vi "MultiOpto_1.4_Host.vi"() -> ()   [LabVIEW 2018]
uses:
  D:/NI LabVIEW/MultiOpto/MultiOpto_1.4/AT lib/Spels.AutomationTools.Utility.Wcf.dll
  AT lib/Spels.AutomationTools.Utility.Wcf.dll
  D:/NI LabVIEW/MultiOpto/MultiOpto_1.4/AT lib/AmateurStepperMotor.dll
  AT lib/AmateurStepperMotor.dll
  <instrlib>/niDCPower/nidcpower.llb/niDCPower Measurement Type.ctl
  <instrlib>/niDMM/nidmm.llb/niDMM Resolution in Digits.ctl
  <instrlib>/niDMM/nidmm.llb/niDMM Function.ctl
  <instrlib>/niDMM/nidmm.llb/niDMM Configure Measurement Digits.vi
  <instrlib>/niScope/Configure/Trigger/niScope Configure Trigger Window.vi
  <instrlib>/niScope/Acquire/Fetch/niScope Multi Fetch Cluster.vi
  <instrlib>/niScope/Acquire/Fetch/niScope Fetch.vi
panel:
  in  "POWER":bool
  in  "DC POWER 2":refnum<k15>="PXI1Slot3_3" caption="PRBS"
  in  "DC POWER 1":refnum<k15>="PXI1Slot2_2" caption="VСС_+5"
  in  "Tab DC Power 4":enum32{"DC Power 4", "System Panel"}(tab)
  in  "P4 CH2":bool
  out "P4 CH2_char":dbl(graph)=-2.6497095286784e-07
  in  "P4 CH2, V":dbl caption="voltage level" min=-20.0 max=0.0 format="%_6p"
  out "P4 CH2_cur, A":dbl=-2.6497095286784e-07 caption="measurement" format="%_6g"
  in  "P4 CH2_curlim, A":dbl=0.015 caption="current limit" min=0.01 max=1.0 format="%_6p"
  in  "P4 CH1":bool
  out "P4 CH1_char":dbl(graph)=-6.586231837824974e-06
  in  "P4 CH1, V":dbl=20.0 caption="voltage level" min=0.0 max=20.0 format="%_6p"
  out "P4 CH1_cur, A":dbl=-6.586231837824974e-06 caption="measurement" format="%_6g"
  in  "P4 CH1_curlim, A":dbl=0.1 caption="current limit" min=0.01 max=1.0 format="%_6p"
  in  "P4 CH0":bool
  out "P4 CH0_char":dbl(graph)=0.00011627237241327378
  in  "P4 CH0, V":dbl=1.2000000000000002 caption="voltage level" min=0.0 max=6.0 format="%_6p"
  out "P4 CH0_cur, A":dbl=0.00011627237241327378 caption="measurement" format="%_6g"
  in  "P4 CH0_curlim, A":dbl=0.04 caption="current limit" min=0.01 max=1.0 format="%_6p"
  in  "P4 CH0_selcur, A":dbl=0.2 caption="current limit" format="%_6p"
  out "P4 CH0_warning":bool caption="VCC_warning"
  out "P4 CH0_counter":u32 caption="VCC_counter"
  in  "P4 CH1_selcur, A":dbl=0.2 caption="current limit" format="%_6p"
  out "P4 CH1_warning":bool caption="VCC_warning"
  out "P4 CH1_counter":u32 caption="VCC_counter"
  in  "P4 CH2_selcur, A":dbl=0.2 caption="current limit" format="%_6p"
  out "P4 CH2_warning":bool caption="VCC_warning"
  out "P4 CH2_counter":u32 caption="VCC_counter"
  in  "P4 CH2 Used":bool caption="CH2"
  in  "P4 CH0 Used":bool caption="CH0"
  in  "P4 CH1 Used":bool caption="CH1"
  out "DC Power 4 error out":errorcluster
  in  "Tab DC Power 3":enum32{"DC Power 3", "System Panel"}(tab)
  in  "P3 CH2":bool
  out "P3 CH2_char":dbl(graph)=-2.6497095286784e-07
  in  "P3 CH2, V":dbl caption="voltage level" min=-20.0 max=0.0 format="%_6p"
  out "P3 CH2_cur, A":dbl=-2.6497095286784e-07 caption="measurement" format="%_6g"
  in  "P3 CH2_curlim, A":dbl=0.015 caption="current limit" min=0.01 max=1.0 format="%_6p"
  in  "P3 CH1":bool
  out "P3 CH1_char":dbl(graph)=-6.586231837824974e-06
  in  "P3 CH1, V":dbl=20.0 caption="voltage level" min=0.0 max=20.0 format="%_6p"
  out "P3 CH1_cur, A":dbl=-6.586231837824974e-06 caption="measurement" format="%_6g"
  in  "P3 CH1_curlim, A":dbl=0.1 caption="current limit" min=0.01 max=1.0 format="%_6p"
  in  "P3 CH0":bool
  out "P3 CH0_char":dbl(graph)=0.00011627237241327378
  in  "P3 CH0, V":dbl=1.2000000000000002 caption="voltage level" min=0.0 max=6.0 format="%_6p"
  out "P3 CH0_cur, A":dbl=0.00011627237241327378 caption="measurement" format="%_6g"
  in  "P3 CH0_curlim, A":dbl=0.04 caption="current limit" min=0.01 max=1.0 format="%_6p"
  in  "P3 CH2_selcur, A":dbl=0.2 caption="current limit" format="%_6p"
  out "P3 CH2_warning":bool caption="VCC_warning"
  out "P3 CH2_counter":u32 caption="VCC_counter"
  in  "P3 CH1_selcur, A":dbl=0.2 caption="current limit" format="%_6p"
  out "P3 CH1_warning":bool caption="VCC_warning"
  out "P3 CH1_counter":u32 caption="VCC_counter"
  in  "P3 CH0_selcur, A":dbl=0.2 caption="current limit" format="%_6p"
  out "P3 CH0_warning":bool caption="VCC_warning"
  out "P3 CH0_counter":u32 caption="VCC_counter"
  in  "P3 CH2 Used":bool caption="CH2"
  in  "P3 CH1 Used":bool caption="CH1"
  in  "P3 CH0 Used":bool caption="CH0"
  out "DC Power 3 error out":errorcluster
  in  "DC POWER 4":refnum<k15>="PXI1Slot5_3" caption="PRBS"
  in  "DC POWER 3":refnum<k15>="PXI1Slot4_3" caption="PRBS"
  in  "Desicion Panel":enum32{"Decision Panel", "System Panel"}(tab)
  in  "HMI Stop":bool
  out "SEU":bool caption="SEL"
  out "SEL":bool
  out "DC Power 4 Status":bool caption="DC Power 4"
  out "DC Power 3 Status":bool caption="DC Power 3"
  out "DC Power 1 Status":bool caption="DC Power 1"
  out "DC Power 2 Status":bool caption="DC Power 2"
  out "NI DMM 1 Status":bool caption="NI DMM 1"
  out "NI DMM 2 Status":bool caption="NI DMM 2"
  out "NI DMM 3 Status":bool caption="NI DMM 3"
  out "NI Scope Status":bool caption="NI Scope"
  out "Stepper Motor Status":bool caption="Stepper Motor"
  out "Ophir 2 Status":bool caption="Ophir 2"
  out "Ophir 1 Status":bool caption="Ophir 1"
  in  "SEL Time Cycle":u32=100
  in  "SEL path":path=path "D:/NI LabVIEW/MultiOpto/MultiOpto_1.2/Logs/SEL" caption="SEL Path"
  in  "SIM_SEL":bool
  in  "Считать SIM_SEL":bool
  in  "System Stop":bool
  out "Ready Status":bool
  out "Power OFF":bool
  in  "Tab DC Power 2":enum32{"DC Power 2", "System Panel"}(tab)
  in  "P2 CH2_selcur, A":dbl=0.2 caption="current limit" format="%_6p"
  out "P2 CH2_warning":bool caption="VCC_warning"
  out "P2 CH2_counter":u32 caption="VCC_counter"
  in  "P2 CH2 Used":bool caption="CH2"
  in  "P2 CH2_curlim, A":dbl=0.015 caption="current limit" min=0.01 max=1.0 format="%_6p"
  out "P2 CH2_cur, A":dbl=-2.6497095286784e-07 caption="measurement" format="%_6g"
  in  "P2 CH2, V":dbl caption="voltage level" min=-20.0 max=0.0 format="%_6p"
  out "P2 CH2_char":dbl(graph)=-2.6497095286784e-07
  in  "P2 CH2":bool
  in  "P2 CH0 Used":bool caption="CH0"
  out "P2 CH0_char":dbl(graph)=0.00011627237241327378
  in  "P2 CH0, V":dbl=1.2000000000000002 caption="voltage level" min=0.0 max=6.0 format="%_6p"
  out "P2 CH0_cur, A":dbl=0.00011627237241327378 caption="measurement" format="%_6g"
  in  "P2 CH0_curlim, A":dbl=0.04 caption="current limit" min=0.01 max=1.0 format="%_6p"
  in  "P2 CH0":bool
  out "P2 CH0_warning":bool caption="VCC_warning"
  out "P2 CH0_counter":u32 caption="VCC_counter"
  in  "P2 CH0_selcur, A":dbl=0.2 caption="current limit" format="%_6p"
  in  "P2 CH1_curlim, A":dbl=0.1 caption="current limit" min=0.01 max=1.0 format="%_6p"
  out "P2 CH1_cur, A":dbl=-6.586231837824974e-06 caption="measurement" format="%_6g"
  in  "P2 CH1, V":dbl=20.0 caption="voltage level" min=0.0 max=20.0 format="%_6p"
  out "P2 CH1_char":dbl(graph)=-6.586231837824974e-06
  in  "P2 CH1":bool
  in  "P2 CH1 Used":bool caption="CH1"
  in  "P2 CH1_selcur, A":dbl=0.2 caption="current limit" format="%_6p"
  out "P2 CH1_counter":u32 caption="VCC_counter"
  out "P2 CH1_warning":bool caption="VCC_warning"
  out "DC Power 2 error out":errorcluster
  in  "Tab DC Power 1":enum32{"DC Power 1", "System Panel"}(tab)
  out "P1 CH2_counter":u32 caption="VCC_counter"
  out "P1 CH2_warning":bool caption="VCC_warning"
  in  "P1 CH2_selcur, A":dbl=0.2 caption="current limit" format="%_6p"
  in  "P1 CH2 Used":bool caption="CH2"
  in  "P1 CH2_curlim, A":dbl=0.01 caption="current limit" min=0.01 max=1.0 format="%_6p"
  out "P1 CH2_cur, A":dbl=1.4003158139382402e-06 caption="measurement" format="%_6g"
  in  "P1 CH2, V":dbl=-5.0 caption="voltage level" min=-20.0 max=0.0 format="%_6p"
  out "P1 CH2_char":dbl(graph)=1.4003158139382402e-06
  in  "P1 CH2":bool
  in  "P1 CH1 Used":bool caption="CH1"
  in  "P1 CH0 Used":bool caption="CH0"
  out "P1 CH0_char":dbl(graph)=8.200132019086688e-05
  in  "P1 CH0, V":dbl=3.3000000000000003 caption="voltage level" min=0.0 max=6.0 format="%_6p"
  out "P1 CH0_cur, A":dbl=8.200132019086688e-05 caption="measurement" format="%_6g"
  in  "P1 CH0_curlim, A":dbl=0.08 caption="current limit" min=0.01 max=1.0 format="%_6p"
  out "P1 CH1_char":dbl(graph)=9.464711192498274e-07
  in  "P1 CH1, V":dbl=2.0 caption="voltage level" min=0.0 max=20.0 format="%_6p"
  out "P1 CH1_cur, A":dbl=9.464711192498274e-07 caption="measurement" format="%_6g"
  in  "P1 CH1_curlim, A":dbl=0.1 caption="current limit" min=0.01 max=1.0 format="%_6p"
  in  "P1 CH0":bool
  in  "P1 CH1":bool
  out "P1 CH0_warning":bool caption="VCC_warning"
  out "P1 CH0_counter":u32 caption="VCC_counter"
  out "P1 CH1_warning":bool caption="VCC_warning"
  out "P1 CH1_counter":u32 caption="VCC_counter"
  in  "P1 CH1_selcur, A":dbl=0.2 caption="current limit" format="%_6p"
  in  "P1 CH0_selcur, A":dbl=0.2 caption="current limit" format="%_6p"
  out "DC Power 1 error out":errorcluster
  out "SEL output file refnum":refnum<file>
  in  "Table Tab":enum32{"Glass Table", "Var", "Log"}(tab)
  in  "Add Log Remark":bool
  in  "Glass Table":string[][](table)=[["", "455 nm", "808 nm", "1550 nm"], ["Glass 1 (H-ZLaF90)", "", "", ""], ["Glass 2 (H-K9L)", "", "", ""], ["Glass 3 (H-ZF7LA)", "", "", ""], ["Glass 4 (H-LaK7A)", "", "", ""]]
  in  "Clear Table":bool
  out "Num of Meas":u32
  in  "Log Remark":string
  out "WL 808":dbl format="%#_4g"
  out "WL 455":dbl format="%#_4g"
  out "WL 1550":dbl format="%#_4g"
  out "WL 1550 Ref":dbl=1.0 format="%#_4g"
  out "WL 455 Ref":dbl=1.0 format="%#_4g"
  out "WL 808 Ref":dbl=1.0 format="%#_4g"
  out "WL 455 Absolute/Reference":string="-" caption="WL 455 Abs/Ref"
  out "WL 808 Absolute/Reference":string="-" caption="WL 808 Abs/Ref"
  out "WL 1550 Absolute/Reference":string="-" caption="WL 1550 Abs/Ref"
  in  "Set Last Meas As Ref":bool
  out "Образец №":string="0"
  in  "All Glass Path":path=path "D:/NI LabVIEW/MultiOpto/MultiOpto_1.2/Logs/All Glass"
  in  "NI Scope":refnum<k15>="PXI1Slot9_2" caption="Scope"
  in  "NI DMM 3":refnum<k15>="PXI1Slot6_3" caption="NI DMM 2"
  in  "Stepper Motor Control":enum32{"Stepper Motor", "System Panel", "Var"}(tab)
  out "Текущая позиция":dbl
  in  "Куда едем?":T1(ring)
  in  "Glass Meas":bool caption="Glass Measurement"
  out "Meas Running":bool
  out "Glass Meas Cycle Running":bool caption="Cycle Running"
  in  "Погнали!":bool
  out "Готово":bool
  in  "Glass Meas Cycle":bool caption="Glass Measament Cycle"
  out "Meas Progress Bar":u8(slide) caption="Measurement Progress Bar" scale=0.0..100.0
  in  "StepDivisor":i32(ring)=8 items=["D1"=1, "D2"=2, "D4"=4, "D8"=8, "D16"=16, "D32"=32]
  in  "Speed":dbl=1000.0
  in  "StepMultiplicationFactor":dbl=1.0
  in  "Стоп_тест":bool
  in  "Тест":bool
  in  "Стоп GoTo":bool
  in  "Meas Wait":u32=500
  out "Av Cur Data String":string="0,000016350563\t"
  out "Glass Num Output File":refnum<file>
  out "Glass 1 Output File":refnum<file>
  out "CH Data String":string="1,200000000000\t0,040047418764\t"
  out "All Cur Data String":string="0,000016366024\t0,000016373619\t0,000016386890\t0,000016310874\t0,000016315407\t"
  out "Meas Time String":string="19:17:01:,978\t"
  out "Glass Meas Path":refnum<file>
  out "Glass 2 Output File":refnum<file>
  out "Glass 3 Output File":refnum<file>
  out "Glass 4 Output File":refnum<file>
  out "Glass Full Log Output File":refnum<file>
  out "Save Glass Log Done":bool=TRUE
  in  "Save Glass Log Data":bool
  out "WL-i":i32
  out "Single Meas Output File":refnum<file>
  in  "NI DMM 3 Tab":enum32{"Amp", "Ohm", "System Panel", "Var"}(tab)
  in  "NI DMM 3 Ampermeter path":path=path "D:/NI LabVIEW/MultiOpto/MultiOpto_1.2/Logs/DMM 3" caption="Ampermeter Path"
  out "NI DMM 3 Current Char":dbl(graph)=0.00060711613514286
  in  "NI DMM 3 Current Wait":u32=100 caption="Wait"
  out "NI DMM 3 Current":dbl=0.00060711613514286 caption="Current" format="%_6g"
  in  "NI DMM 3 units":string(combo)="1000000" caption="Units"
  in  "NI DMM 3 Current Range":string(combo)="-1" caption="Range"
  in  "NI DMM 3 Ohmmeter path":path=path "D:/NI LabVIEW/MultiOpto/MultiOpto_1.2/Logs/DMM 3" caption="Ohmmeter Path"
  out "NI DMM 3 Resistance Char":dbl(graph)=6.67426339573744e-05
  in  "NI DMM 3 Resistance Wait":u32=100 caption="Wait"
  out "NI DMM 3 Resistance":dbl caption="Resistance" format="%_6g"
  in  "NI DMM 3 Resistance units":string(combo)="1" caption="Units"
  in  "NI DMM 3 Resistance Range":string(combo)="-1" caption="Range"
  out "NI DMM 3 Current output file":refnum<file>
  out "NI DMM 3 Resistance output file":refnum<file>
  in  "NI DMM 3 error in":errorcluster
  out "NI DMM 3 Option Return":enum32{"Ampermeter button", "Ohmmeter button"}(ring)
  out "NI DMM 3 error out":errorcluster
  out "DMM 3 Real Current":dbl=6.0711613514286e-10 format="%.15f"
  in  "NI DMM 1":refnum<k15>="PXI1Slot4"
  in  "NI DMM 2":refnum<k15>="PXI1Slot5"
  in  "Ophir 2 Tab":T2(tab)
  out "Ophir 2 Initialization":bool caption="Initialization"
  in  "Ophir 2 Clear":bool caption="Clear"
  out "Ophir 2 MAX":dbl caption="MAX" format="%#_5g"
  out "Ophir 2 Optical Power":dbl caption="Power" format="%#_4g"
  in  "Ophir 2 units":string(combo)="1000" caption="Units"
  in  "Ophir 2 Info":u16(ring)=1 caption="Info" items=["Device : JUNO; s/n:903794", "Head : PD300-IRG-v1; s/n:908004"]
  in  "Ophir 2 Wait":u32=100 caption="Wait"
  out "Ophir 2 Char":dbl(graph)=6.67426339573744e-05
  out "Ophir 2 Over Range":bool caption="Over Range"
  out "Ophir 2 dup Visa Session":refnum<visa-resource-name>="USB0::0x0BD3::0x0777::NI-VISA-10003::RAW" caption="dup Visa Session"
  in  "Ophir 2 GPIB Address (10)":string="10" caption="GPIB Address (10)"
  in  "Ophir 2 Select Communication Protocol":u16(ring) caption="Select Communication Protocol" items=["USB", "RS232", "GPIB"]
  in  "Ophir 2 usb channel":i16 caption="usb channel"
  in  "Ophir 2 Baud Rate (3:9600)":i16(ring)=3 caption="Baud Rate (3:9600)" items=["300", "1200", "4800", "9600", "19200", "38400"]
  in  "Ophir 2 Port Number (default 2)":i16=2 caption="Port Number (default 2)" min=0 max=20
  out "Ophir 2 Real Optical Power":dbl format="%.6e"
  out "Ophir 2 error out":errorcluster caption="error out"
  in  "Ophir 2 error in (no error)":errorcluster caption="error in (no error)"
  in  "Ophir 1 Tab":T3(tab)
  out "Ophir 1 Initialization":bool caption="Initialization"
  in  "Ophir 1 units":string(combo)="1000" caption="Units"
  out "Ophir 1 Optical Power":dbl caption="Power" format="%#_4g"
  out "Ophir 1 MAX":dbl caption="MAX" format="%#_5g"
  in  "Ophir 1 Clear":bool caption="Clear"
  in  "Ophir 1 Info":u16(ring)=1 caption="Info" items=["Device : JUNO; s/n:903795", "Head : PD300R-IR   ; s/n:873888"]
  in  "Ophir 1 Wait":u32=100 caption="Wait"
  out "Ophir 1 Char":dbl(graph)=6.67426339573744e-05
  out "Ophir 1 Over Range":bool caption="Over Range"
  in  "Ophir 1 Select Communication Protocol":u16(ring) caption="Select Communication Protocol" items=["USB", "RS232", "GPIB"]
  in  "Ophir 1 usb channel":i16 caption="usb channel"
  in  "Ophir 1 Port Number (default 2)":i16=1 caption="Port Number (default 2)" min=0 max=20
  in  "Ophir 1 Baud Rate (3:9600)":i16(ring)=3 caption="Baud Rate (3:9600)" items=["300", "1200", "4800", "9600", "19200", "38400"]
  in  "Ophir 1 GPIB Address (10)":string="10" caption="GPIB Address (10)"
  out "Ophir 1 dup Visa Session":refnum<visa-resource-name>="USB0::0x0BD3::0x0777::NI-VISA-10003::RAW" caption="dup Visa Session"
  out "Ophir 1 Real Optical Power":dbl format="%.6e"
  out "Ophir 1 error out":errorcluster caption="error out"
  in  "Ophir 1 error in (no error)":errorcluster caption="error in (no error)"
  in  "NI DMM 2 Tab":enum32{"Amp", "Ohm", "System Panel", "Var"}(tab)
  out "NI DMM 2 Current":dbl=0.7074877999002638 caption="Current" format="%_4g"
  out "NI DMM 2 Current Char":dbl(graph)=0.7074877999002638
  in  "NI DMM 2 Ampermeter path":path=path "D:/NI LabVIEW/MultiOpto/MultiOpto_1.2/Logs/DMM 2" caption="Ampermeter Path"
  in  "NI DMM 2 units":string(combo)="1000000" caption="Units"
  in  "NI DMM 2 Current Range":string(combo)="-1" caption="Range"
  in  "NI DMM 2 Current Wait":u32=100 caption="Wait"
  in  "NI DMM 2 Ohmmeter path":path=path "D:/NI LabVIEW/MultiOpto/MultiOpto_1.2/Logs/DMM 2" caption="Ohmmeter Path"
  out "NI DMM 2 Resistance":dbl caption="Resistance" format="%_6g"
  out "NI DMM 2 Resistance Char":dbl(graph)=6.67426339573744e-05
  in  "NI DMM 2 Resistance units":string(combo)="1" caption="Units"
  in  "NI DMM 2 Resistance Range":string(combo)="-1" caption="Range"
  in  "NI DMM 2 Resistance Wait":u32=100 caption="Wait"
  out "NI DMM 2 Current output file":refnum<file>
  out "NI DMM 2 error out":errorcluster
  in  "NI DMM 2 error in":errorcluster
  out "NI DMM 2 Option Return":enum32{"Ampermeter button", "Ohmmeter button"}(ring)
  out "NI DMM 2 Resistance output file":refnum<file>
  out "DMM 2 Real Current":dbl=7.074877999002638e-07 format="%.15f"
  in  "NI DMM 1 Tab":enum32{"Amp", "Ohm", "System Panel", "Var"}(tab)
  out "NI DMM 1 Current Char":dbl(graph)=0.6705812438667635
  out "NI DMM 1 Current":dbl=0.6705812438667635 caption="Current" format="%_6g"
  in  "NI DMM 1 Ampermeter path":path=path "D:/NI LabVIEW/MultiOpto/MultiOpto_1.2/Logs/DMM 1" caption="Ampermeter Path"
  in  "NI DMM 1 units":string(combo)="1000000" caption="Units"
  in  "NI DMM 1 Current Range":string(combo)="-1" caption="Range"
  in  "NI DMM 1 Current Wait":u32=100 caption="Wait"
  in  "NI DMM 1 Ohmmeter path":path=path "D:/NI LabVIEW/MultiOpto/MultiOpto_1.2/Logs/DMM 1" caption="Ohmmeter Path"
  out "NI DMM 1 Resistance":dbl caption="Resistance" format="%_6g"
  out "NI DMM 1 Resistance Char":dbl(graph)=6.67426339573744e-05
  in  "NI DMM 1 Resistance units":string(combo)="1" caption="Units"
  in  "NI DMM 1 Resistance Range":string(combo)="-1" caption="Range"
  in  "NI DMM 1 Resistance Wait":u32=100 caption="Wait"
  out "NI DMM 1 Current output file":refnum<file>
  out "NI DMM 1 error out":errorcluster
  in  "NI DMM 1 error in":errorcluster
  out "NI DMM 1 Option Return":enum32{"Ampermeter button", "Ohmmeter button"}(ring)
  out "NI DMM 1 Resistance output file":refnum<file>
  out "DMM 1 Real Current":dbl=6.705812438667635e-07 format="%.15f"
  in  "NI Scope Tab":enum32{"NI Scope", "System Panel"}(tab)
  in  "vertical range":dbl=2.0 caption="Vertical Range" format="%.2f"
  out "RealTime Waveform":T4(graph) caption="PC_MON Waveform"
  out "SEU Waveform":T4(graph) caption="SHUTDOWN Waveform"
  in  "Low Level":dbl=0.35 format="%.2f"
  in  "High Level":dbl=0.65 format="%.2f"
  in  "AC/DC/Groun":i32(ring)=1 items=["AC", "DC", "Ground"]
  in  "Trigger Source":string(combo)="0"
  in  "SEU path":path=path "D:/NI LabVIEW/MultiOpto 1.1/Logs/SEU" caption="SEU Path"
  in  "Channel for SEU":T5(radio)
  out "SEU Last Level":dbl
  out "SEU_Counter":u32 caption="SEU counter"
  out "SEU_warning":bool caption="Find SEL"
  out "SEU output file refnum":refnum<file>
  out "NI Scope error out":errorcluster
  in  "NI Scope error in":errorcluster
  # "Отожми кнопку для\nединичного промера!"
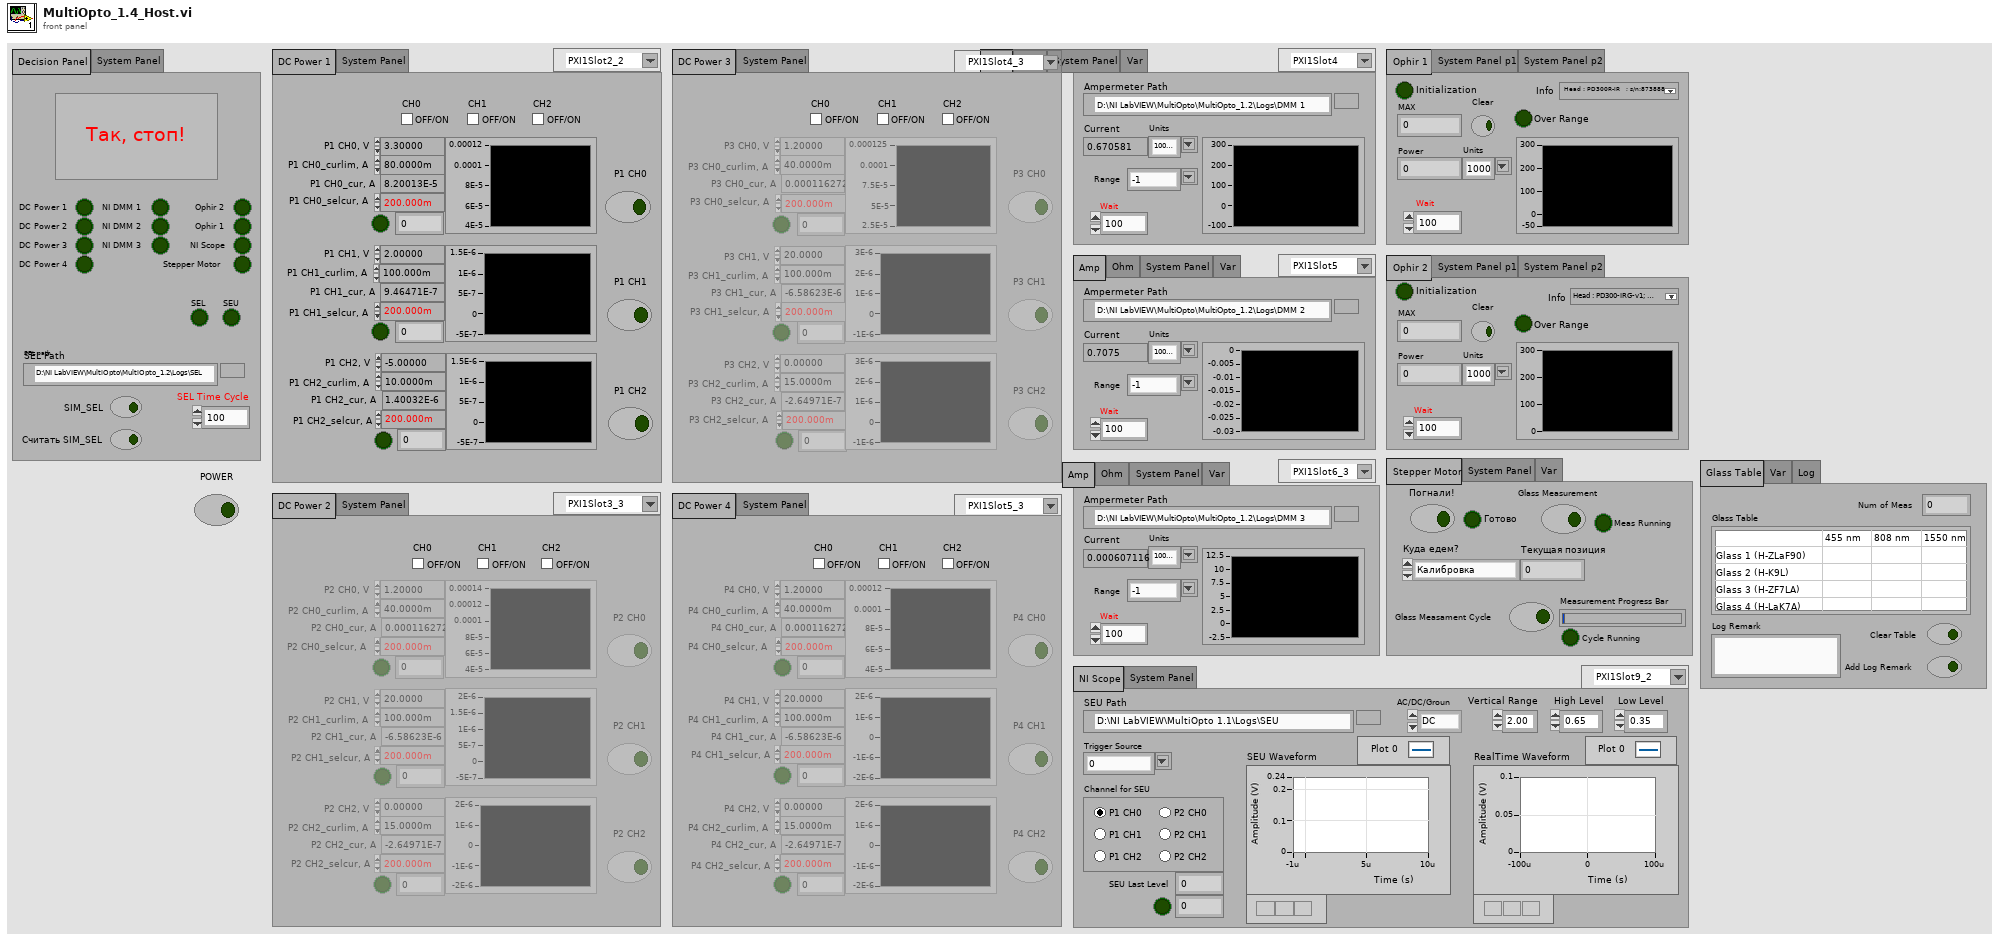
[diagram p1: front panel]
types:
  T1 = enum16{"Калибровка", "Первое стекло", "Второе стекло", "Третье стекло", "Четвертое стекло"}
  T2 = enum32{"Ophir 2", "System Panel p1", "System Panel p2"}
  T3 = enum32{"Ophir 1", "System Panel p1", "System Panel p2"}
  T4 = cluster{"relativeInitialX":dbl, "xIncrement":dbl, "wfm":dbl[]}[]
  T5 = enum32{"Radio Selection P1 CH0", "Radio Selection P1 CH1", "Radio Selection P2 CH0", "Radio Selection P2 CH1", "Radio Selection P2 CH2", "Radio Selection P1 CH2"}
  T6 = enum16{"open", "replace", "create", "open or create", "replace or create", "replace or create with confirmation"}
  T7 = enum8{"Enabled", "Disabled", "Disabled and Grayed Out"}
  T8 = typedef "niDMM Function.ctl" = enum16{"DC Volts", "AC Volts", "DC Current", "AC Current", "2-wire Resistance", "4-wire Resistance", "Diode", "Frequency", "Period", "AC Volts DC Coupled", "Capacitance", "Inductance", "Temperature"}
  T9 = typedef "niDMM Resolution in Digits.ctl" = dbl
  T10 = typedef "niDCPower Measurement Type.ctl" = i32
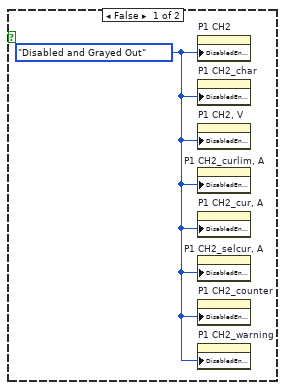
[diagram p3: hidden frame]
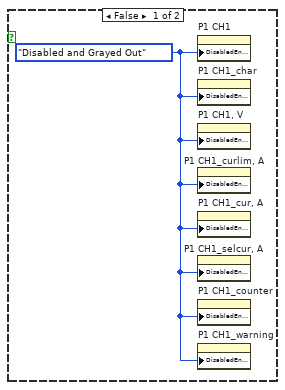
[diagram p4: hidden frame]
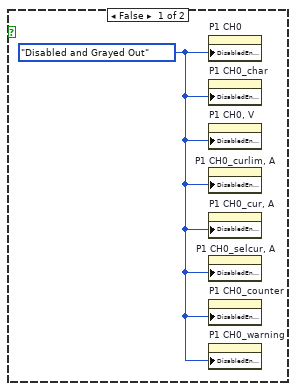
[diagram p5: hidden frame]
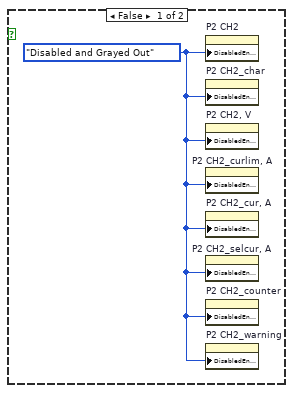
[diagram p7: hidden frame]
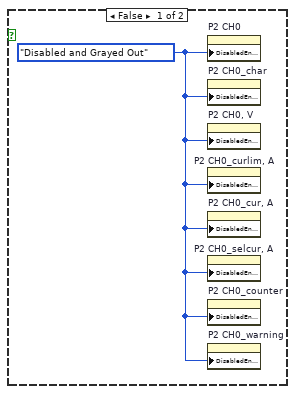
[diagram p8: hidden frame]
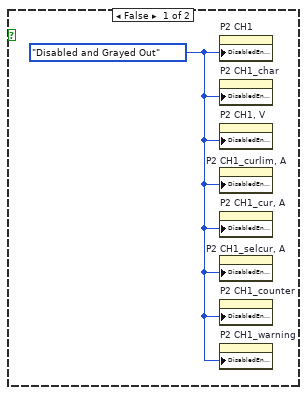
[diagram p9: hidden frame]
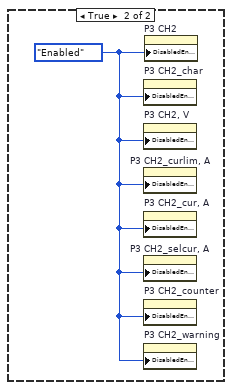
[diagram p11: hidden frame]
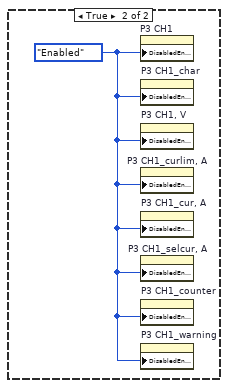
[diagram p12: hidden frame]
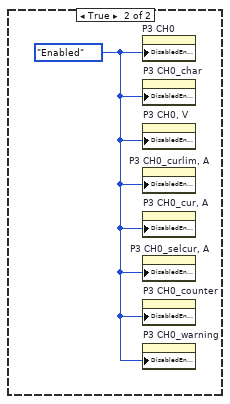
[diagram p13: hidden frame]
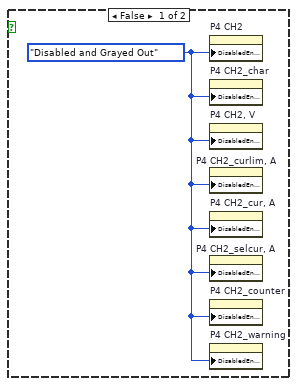
[diagram p15: hidden frame]
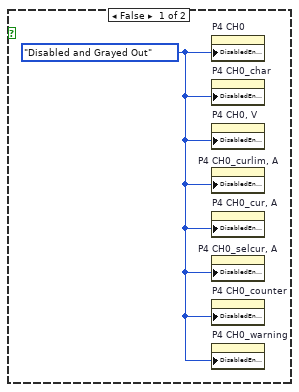
[diagram p16: hidden frame]
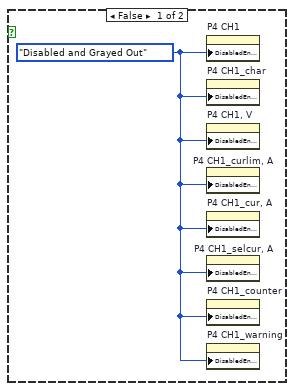
[diagram p17: hidden frame]
diagram:
  w12 = FALSE ("P1 CH0")
  w7 = FALSE
  # "DMM 3"
  # "DMM 2"
  # "DMM 1"
  n1 = stacked-sequence {
    tunnel: [_ _ _ _ _ w354 _ _ _ _ _ _] -> w50
    tunnel: [_ _ _ _ _ w353 _ _ _ _ _ _] -> w48
    tunnel: [_ _ _ _ _ w352 _ _ _ _ _ _] -> w29
    tunnel: [_ _ _ _ _ _ _ _ _ _ _ w727] -> w1
    tunnel: [_ _ _ _ _ _ _ _ _ _ _ w727] -> w2
    tunnel: [_ _ _ _ _ _ w401 _ _ _ _ _] -> w47
    tunnel: [_ _ _ _ _ _ _ w460 _ _ _ _] -> w46
    tunnel: [_ _ _ _ _ _ _ w463 _ _ _ _] -> w45
    tunnel: [_ _ _ _ _ _ w400 _ _ _ _ _] -> w44
    tunnel: [_ _ _ _ _ _ _ w459 _ _ _ _] -> w43
    tunnel: [_ _ _ _ _ _ _ w458 _ _ _ _] -> w42
    tunnel: [_ _ _ _ _ _ w399 _ _ _ _ _] -> w41
    tunnel: [_ _ _ _ _ _ _ w462 _ _ _ _] -> w40
    tunnel: [_ _ _ _ _ _ _ w461 _ _ _ _] -> w39
    tunnel: [_ _ _ _ _ _ _ _ w656 _ _ _] -> w38
    tunnel: [_ _ _ _ _ _ _ _ _ w679 _ _] -> w37
    tunnel: [_ _ _ _ _ _ _ w457 _ _ _ _] -> w30
    tunnel: [_ _ _ _ _ _ _ w456 _ _ _ _] -> w36
    tunnel: [_ _ _ _ _ _ _ w455 _ _ _ _] -> w35
    tunnel: [_ _ _ _ _ _ _ _ _ _ w705 _] -> w34
    tunnel: [_ _ _ _ _ _ _ _ _ _ w704 _] -> w33
    tunnel: [_ _ _ _ _ _ _ _ _ _ w703 _] -> w32
    tunnel: [_ _ _ _ _ _ _ _ _ _ w702 _] -> w31
    tunnel: [_ _ _ _ _ w351 _ _ _ _ _ _] -> w28
    tunnel: [_ _ _ _ _ w346 _ _ _ _ _ _] -> w25
    tunnel: [_ _ _ _ _ w345 _ _ _ _ _ _] -> w24
    tunnel: [_ _ _ _ _ w350 _ _ _ _ _ _] -> w22
    tunnel: [_ _ _ _ _ w349 _ _ _ _ _ _] -> w21
    tunnel: [_ _ _ _ _ w344 _ _ _ _ _ _] -> w16
    tunnel: [_ _ _ _ _ w348 _ _ _ _ _ _] -> w15
    tunnel: [_ _ _ _ _ w347 _ _ _ _ _ _] -> w14
    tunnel: [_ _ _ _ _ w343 _ _ _ _ _ _] -> w13
    tunnel: [_ _ _ _ _ w346 _ _ _ _ _ _] -> w3
    tunnel: [_ _ _ _ _ w345 _ _ _ _ _ _] -> w4
    tunnel: [_ _ _ _ _ w344 _ _ _ _ _ _] -> w5
    tunnel: [_ _ _ _ _ w343 _ _ _ _ _ _] -> w6
    frame #0 {
      w53 = FALSE ("Ready Status")
      w55 = FALSE ("Clear Table")
      w58 = "-" ("WL 455 Absolute/Reference")
      w59 = 0.0 ("WL 455 Ref")
      w60 = 1.0 ("WL 455")
      w62 = "\t" ("Meas Time String")
      w63 = FALSE ("Save Glass Log Done")
      w65 = FALSE ("Погнали!")
      w69 = FALSE
      w68 = FALSE ("NI Scope Status")
      w72 = u32 0 ("SEU_Counter")
      w54 = FALSE ("STOP")
      # "Начальная конфигурация переменных"
      n2 = local write "Текущая позиция"(0.0 ("Текущая позиция")) -> ()
      n3 = local write "Куда едем?"(T1."Калибровка" ("Куда едем?")) -> ()
      n4 = local write "Погнали!"(w65) -> ()
      n5 = local write "Тест"(w65) -> ()
      n6 = local write "Стоп GoTo"(w65) -> ()
      n7 = local write "Стоп_тест"(w65) -> ()
      n8 = local write "Готово"(w65) -> ()
      n9 = local write "Num of Meas"(u32 0 ("Num of Meas")) -> ()
      n10 = local write "WL 455"(w60) -> ()
      n11 = local write "WL 808"(w60) -> ()
      n12 = local write "WL 1550"(w60) -> ()
      n13 = local write "WL 455 Ref"(w59) -> ()
      n14 = local write "WL 808 Ref"(w59) -> ()
      n15 = local write "WL 1550 Ref"(w59) -> ()
      n16 = local write "WL 455 Absolute/Reference"(w58) -> ()
      n17 = local write "WL 808 Absolute/Reference"(w58) -> ()
      n18 = local write "WL 1550 Absolute/Reference"(w58) -> ()
      n19 = local write "Ophir 2 Over Range"(w69) -> ()
      n20 = local write "Ophir 1 Over Range"(w69) -> ()
      n21 = local write "Ophir 1 Initialization"(w69) -> ()
      n22 = local write "Ophir 2 Initialization"(w69) -> ()
      n23 = local write "Ophir 1 Clear"(w69) -> ()
      n24 = local write "Ophir 2 Clear"(w69) -> ()
      n25 = local write "Meas Time String"(w62) -> ()
      n26 = local write "All Cur Data String"(w62) -> ()
      n27 = local write "Av Cur Data String"(w62) -> ()
      n28 = local write "CH Data String"(w62) -> ()
      n29 = local write "WL-i"(0 ("i-WL")) -> ()
      n30 = local write "Save Glass Log Data"(w63) -> ()
      n31 = local write "Save Glass Log Done"(w63) -> ()
      n32 = local write "Glass Meas Cycle"(w63) -> ()
      n33 = local write "Glass Meas"(w63) -> ()
      n34 = local write "Meas Running"(w63) -> ()
      n35 = local write "Glass Meas Cycle Running"(w63) -> ()
      n36 = local write "P2 CH2_warning"(w54) -> ()
      n37 = local write "HMI Stop"(w54) -> ()
      n38 = local write "System Stop"(w54) -> ()
      n39 = local write "P1 CH0"(w54) -> ()
      n40 = local write "P1 CH1"(w54) -> ()
      n41 = local write "P1 CH2"(w54) -> ()
      n42 = local write "P2 CH0"(w54) -> ()
      n43 = local write "P2 CH1"(w54) -> ()
      n44 = local write "P2 CH2"(w54) -> ()
      n45 = local write "Power OFF"(w54) -> ()
      n46 = local write "P1 CH0 Used"(w54) -> ()
      n47 = local write "P1 CH1 Used"(w54) -> ()
      n48 = local write "P1 CH2 Used"(w54) -> ()
      n49 = local write "P2 CH0 Used"(w54) -> ()
      n50 = local write "P2 CH1 Used"(w54) -> ()
      n51 = local write "P2 CH2 Used"(w54) -> ()
      n52 = local write "SEL"(w54) -> ()
      n53 = local write "Считать SIM_SEL"(w54) -> ()
      n54 = local write "SEU"(w54) -> ()
      n55 = local write "SEU_warning"(w54) -> ()
      n56 = local write "P1 CH0_warning"(w54) -> ()
      n57 = local write "P1 CH1_warning"(w54) -> ()
      n58 = local write "P1 CH2_warning"(w54) -> ()
      n59 = local write "P2 CH0_warning"(w54) -> ()
      n60 = local write "P2 CH1_warning"(w54) -> ()
      n61 = local write "SEU_warning"(w54) -> ()
      n62 = local write "Log Remark"("" ("Log Remark")) -> ()
      n63 = local write "Set Last Meas As Ref"(w55) -> ()
      n64 = local write "Clear Table"(w55) -> ()
      n65 = local write "Add Log Remark"(w55) -> ()
      n66 = local write "SEU Last Level"(0.0 ("SEU Level")) -> ()
      n67 = local write "SEU_Counter"(w72) -> ()
      n68 = local write "P1 CH0_counter"(w72) -> ()
      n69 = local write "P1 CH1_counter"(w72) -> ()
      n70 = local write "P2 CH0_counter"(w72) -> ()
      n71 = local write "P2 CH1_counter"(w72) -> ()
      n72 = local write "Образец №"("" ("Образец №")) -> ()
      n73 = local write "Ready Status"(FALSE ("Ready Status")) -> ()
      n74 = local write "NI Scope Status"(w68) -> ()
      n75 = local write "NI DMM 2 Status"(w68) -> ()
      n76 = local write "NI DMM 1 Status"(w68) -> ()
      n77 = local write "NI DMM 3 Status"(w68) -> ()
      n78 = local write "Ophir 1 Status"(w68) -> ()
      n79 = local write "Ophir 2 Status"(w68) -> ()
      n80 = local write "Stepper Motor Status"(w68) -> ()
      n81 = local write "P3 CH0"(w53) -> ()
      n82 = local write "P3 CH1"(w53) -> ()
      n83 = local write "P3 CH2"(w53) -> ()
      n84 = local write "P4 CH0"(w53) -> ()
      n85 = local write "P4 CH1"(w53) -> ()
      n86 = local write "P4 CH2"(w53) -> ()
      n87 = local write "P3 CH0 Used"(w53) -> ()
      n88 = local write "P3 CH1 Used"(w53) -> ()
      n89 = local write "P3 CH2 Used"(w53) -> ()
      n90 = local write "P4 CH0 Used"(w53) -> ()
      n91 = local write "P4 CH1 Used"(w53) -> ()
      n92 = local write "P4 CH2 Used"(w53) -> ()
      n93 = local write "P3 CH0_warning"(w53) -> ()
      n94 = local write "P3 CH1_warning"(w53) -> ()
      n95 = local write "P4 CH0_warning"(w53) -> ()
      n96 = local write "P4 CH1_warning"(w53) -> ()
      n97 = local write "P3 CH2_warning"(w53) -> ()
      n98 = local write "P4 CH2_warning"(w53) -> ()
      "Meas Progress Bar" <- u8 0 ("Measuering Progress Bar")
    }
    frame #1 {
      n99 = stacked-sequence {
        frame #0 {
          w74 = T7."Disabled and Grayed Out" ("Disabled")
          n100 = property on="P3 CH0" class="Bool (strict)"("DisabledEnum"=w74) -> ()  [unwired: 2 in, 2 out]
          n101 = property on="P3 CH0_char" class="WFChart (strict)"("DisabledEnum"=w74) -> ()  [unwired: 2 in, 2 out]
          n102 = property on="P3 CH0, V" class="DigNum (strict)"("DisabledEnum"=w74) -> ()  [unwired: 2 in, 2 out]
          n103 = property on="P3 CH0_curlim, A" class="DigNum (strict)"("DisabledEnum"=w74) -> ()  [unwired: 2 in, 2 out]
          n104 = property on="P3 CH0_cur, A" class="DigNum (strict)"("DisabledEnum"=w74) -> ()  [unwired: 2 in, 2 out]
          n105 = property on="P3 CH0_selcur, A" class="DigNum (strict)"("DisabledEnum"=w74) -> ()  [unwired: 2 in, 2 out]
          n106 = property on="P3 CH0_counter" class="DigNum (strict)"("DisabledEnum"=w74) -> ()  [unwired: 2 in, 2 out]
          n107 = property on="P3 CH0_warning" class="Bool (strict)"("DisabledEnum"=w74) -> ()  [unwired: 2 in, 2 out]
        }
        frame #1 {
          w75 = T7."Disabled and Grayed Out" ("Disabled")
          n108 = property on="P3 CH1" class="Bool (strict)"("DisabledEnum"=w75) -> ()  [unwired: 2 in, 2 out]
          n109 = property on="P3 CH1_char" class="WFChart (strict)"("DisabledEnum"=w75) -> ()  [unwired: 2 in, 2 out]
          n110 = property on="P3 CH1, V" class="DigNum (strict)"("DisabledEnum"=w75) -> ()  [unwired: 2 in, 2 out]
          n111 = property on="P3 CH1_curlim, A" class="DigNum (strict)"("DisabledEnum"=w75) -> ()  [unwired: 2 in, 2 out]
          n112 = property on="P3 CH1_cur, A" class="DigNum (strict)"("DisabledEnum"=w75) -> ()  [unwired: 2 in, 2 out]
          n113 = property on="P3 CH1_selcur, A" class="DigNum (strict)"("DisabledEnum"=w75) -> ()  [unwired: 2 in, 2 out]
          n114 = property on="P3 CH1_counter" class="DigNum (strict)"("DisabledEnum"=w75) -> ()  [unwired: 2 in, 2 out]
          n115 = property on="P3 CH1_warning" class="Bool (strict)"("DisabledEnum"=w75) -> ()  [unwired: 2 in, 2 out]
        }
        frame #2 {
          w76 = T7."Disabled and Grayed Out" ("Disabled")
          n116 = property on="P3 CH2_char" class="WFChart (strict)"("DisabledEnum"=w76) -> ()  [unwired: 2 in, 2 out]
          n117 = property on="P3 CH2, V" class="DigNum (strict)"("DisabledEnum"=w76) -> ()  [unwired: 2 in, 2 out]
          n118 = property on="P3 CH2_curlim, A" class="DigNum (strict)"("DisabledEnum"=w76) -> ()  [unwired: 2 in, 2 out]
          n119 = property on="P3 CH2_cur, A" class="DigNum (strict)"("DisabledEnum"=w76) -> ()  [unwired: 2 in, 2 out]
          n120 = property on="P3 CH2_selcur, A" class="DigNum (strict)"("DisabledEnum"=w76) -> ()  [unwired: 2 in, 2 out]
          n121 = property on="P3 CH2_counter" class="DigNum (strict)"("DisabledEnum"=w76) -> ()  [unwired: 2 in, 2 out]
          n122 = property on="P3 CH2_warning" class="Bool (strict)"("DisabledEnum"=w76) -> ()  [unwired: 2 in, 2 out]
          n123 = property on="P3 CH2" class="Bool (strict)"("DisabledEnum"=w76) -> ()  [unwired: 2 in, 2 out]
        }
        frame #3 {
          w77 = T7."Disabled and Grayed Out" ("Disabled")
          n124 = property on="P4 CH0" class="Bool (strict)"("DisabledEnum"=w77) -> ()  [unwired: 2 in, 2 out]
          n125 = property on="P4 CH0_char" class="WFChart (strict)"("DisabledEnum"=w77) -> ()  [unwired: 2 in, 2 out]
          n126 = property on="P4 CH0, V" class="DigNum (strict)"("DisabledEnum"=w77) -> ()  [unwired: 2 in, 2 out]
          n127 = property on="P4 CH0_curlim, A" class="DigNum (strict)"("DisabledEnum"=w77) -> ()  [unwired: 2 in, 2 out]
          n128 = property on="P4 CH0_cur, A" class="DigNum (strict)"("DisabledEnum"=w77) -> ()  [unwired: 2 in, 2 out]
          n129 = property on="P4 CH0_selcur, A" class="DigNum (strict)"("DisabledEnum"=w77) -> ()  [unwired: 2 in, 2 out]
          n130 = property on="P4 CH0_counter" class="DigNum (strict)"("DisabledEnum"=w77) -> ()  [unwired: 2 in, 2 out]
          n131 = property on="P4 CH0_warning" class="Bool (strict)"("DisabledEnum"=w77) -> ()  [unwired: 2 in, 2 out]
        }
        frame #4 {
          w78 = T7."Disabled and Grayed Out" ("Disabled")
          n132 = property on="P4 CH1" class="Bool (strict)"("DisabledEnum"=w78) -> ()  [unwired: 2 in, 2 out]
          n133 = property on="P4 CH1_char" class="WFChart (strict)"("DisabledEnum"=w78) -> ()  [unwired: 2 in, 2 out]
          n134 = property on="P4 CH1, V" class="DigNum (strict)"("DisabledEnum"=w78) -> ()  [unwired: 2 in, 2 out]
          n135 = property on="P4 CH1_curlim, A" class="DigNum (strict)"("DisabledEnum"=w78) -> ()  [unwired: 2 in, 2 out]
          n136 = property on="P4 CH1_cur, A" class="DigNum (strict)"("DisabledEnum"=w78) -> ()  [unwired: 2 in, 2 out]
          n137 = property on="P4 CH1_selcur, A" class="DigNum (strict)"("DisabledEnum"=w78) -> ()  [unwired: 2 in, 2 out]
          n138 = property on="P4 CH1_counter" class="DigNum (strict)"("DisabledEnum"=w78) -> ()  [unwired: 2 in, 2 out]
          n139 = property on="P4 CH1_warning" class="Bool (strict)"("DisabledEnum"=w78) -> ()  [unwired: 2 in, 2 out]
        }
        frame #5 {
          w79 = T7."Disabled and Grayed Out" ("Disabled")
          n140 = property on="P4 CH2" class="Bool (strict)"("DisabledEnum"=w79) -> ()  [unwired: 2 in, 2 out]
          n141 = property on="P4 CH2_char" class="WFChart (strict)"("DisabledEnum"=w79) -> ()  [unwired: 2 in, 2 out]
          n142 = property on="P4 CH2, V" class="DigNum (strict)"("DisabledEnum"=w79) -> ()  [unwired: 2 in, 2 out]
          n143 = property on="P4 CH2_curlim, A" class="DigNum (strict)"("DisabledEnum"=w79) -> ()  [unwired: 2 in, 2 out]
          n144 = property on="P4 CH2_cur, A" class="DigNum (strict)"("DisabledEnum"=w79) -> ()  [unwired: 2 in, 2 out]
          n145 = property on="P4 CH2_selcur, A" class="DigNum (strict)"("DisabledEnum"=w79) -> ()  [unwired: 2 in, 2 out]
          n146 = property on="P4 CH2_counter" class="DigNum (strict)"("DisabledEnum"=w79) -> ()  [unwired: 2 in, 2 out]
          n147 = property on="P4 CH2_warning" class="Bool (strict)"("DisabledEnum"=w79) -> ()  [unwired: 2 in, 2 out]
        }
        frame #6 {
          w80 = T7."Enabled" ("Disabled")
          n148 = property on="P3 CH0 Used" class="Bool (strict)"("DisabledEnum"=w80) -> ()  [unwired: 2 in, 2 out]
          n149 = property on="P3 CH1 Used" class="Bool (strict)"("DisabledEnum"=w80) -> ()  [unwired: 2 in, 2 out]
          n150 = property on="P3 CH2 Used" class="Bool (strict)"("DisabledEnum"=w80) -> ()  [unwired: 2 in, 2 out]
          n151 = property on="P4 CH0 Used" class="Bool (strict)"("DisabledEnum"=w80) -> ()  [unwired: 2 in, 2 out]
          n152 = property on="P4 CH1 Used" class="Bool (strict)"("DisabledEnum"=w80) -> ()  [unwired: 2 in, 2 out]
          n153 = property on="P4 CH2 Used" class="Bool (strict)"("DisabledEnum"=w80) -> ()  [unwired: 2 in, 2 out]
        }
      }
      n154 = stacked-sequence {
        frame #0 {
          w81 = T7."Disabled and Grayed Out" ("Disabled")
          n155 = property on="P1 CH0" class="Bool (strict)"("DisabledEnum"=w81) -> ()  [unwired: 2 in, 2 out]
          n156 = property on="P1 CH0_char" class="WFChart (strict)"("DisabledEnum"=w81) -> ()  [unwired: 2 in, 2 out]
          n157 = property on="P1 CH0, V" class="DigNum (strict)"("DisabledEnum"=w81) -> ()  [unwired: 2 in, 2 out]
          n158 = property on="P1 CH0_curlim, A" class="DigNum (strict)"("DisabledEnum"=w81) -> ()  [unwired: 2 in, 2 out]
          n159 = property on="P1 CH0_cur, A" class="DigNum (strict)"("DisabledEnum"=w81) -> ()  [unwired: 2 in, 2 out]
          n160 = property on="P1 CH0_selcur, A" class="DigNum (strict)"("DisabledEnum"=w81) -> ()  [unwired: 2 in, 2 out]
          n161 = property on="P1 CH0_counter" class="DigNum (strict)"("DisabledEnum"=w81) -> ()  [unwired: 2 in, 2 out]
          n162 = property on="P1 CH0_warning" class="Bool (strict)"("DisabledEnum"=w81) -> ()  [unwired: 2 in, 2 out]
        }
        frame #1 {
          w82 = T7."Disabled and Grayed Out" ("Disabled")
          n163 = property on="P1 CH1" class="Bool (strict)"("DisabledEnum"=w82) -> ()  [unwired: 2 in, 2 out]
          n164 = property on="P1 CH1_char" class="WFChart (strict)"("DisabledEnum"=w82) -> ()  [unwired: 2 in, 2 out]
          n165 = property on="P1 CH1, V" class="DigNum (strict)"("DisabledEnum"=w82) -> ()  [unwired: 2 in, 2 out]
          n166 = property on="P1 CH1_curlim, A" class="DigNum (strict)"("DisabledEnum"=w82) -> ()  [unwired: 2 in, 2 out]
          n167 = property on="P1 CH1_cur, A" class="DigNum (strict)"("DisabledEnum"=w82) -> ()  [unwired: 2 in, 2 out]
          n168 = property on="P1 CH1_selcur, A" class="DigNum (strict)"("DisabledEnum"=w82) -> ()  [unwired: 2 in, 2 out]
          n169 = property on="P1 CH1_counter" class="DigNum (strict)"("DisabledEnum"=w82) -> ()  [unwired: 2 in, 2 out]
          n170 = property on="P1 CH1_warning" class="Bool (strict)"("DisabledEnum"=w82) -> ()  [unwired: 2 in, 2 out]
        }
        frame #2 {
          w83 = T7."Disabled and Grayed Out" ("Disabled")
          n171 = property on="P1 CH2" class="Bool (strict)"("DisabledEnum"=w83) -> ()  [unwired: 2 in, 2 out]
          n172 = property on="P1 CH2_char" class="WFChart (strict)"("DisabledEnum"=w83) -> ()  [unwired: 2 in, 2 out]
          n173 = property on="P1 CH2, V" class="DigNum (strict)"("DisabledEnum"=w83) -> ()  [unwired: 2 in, 2 out]
          n174 = property on="P1 CH2_curlim, A" class="DigNum (strict)"("DisabledEnum"=w83) -> ()  [unwired: 2 in, 2 out]
          n175 = property on="P1 CH2_cur, A" class="DigNum (strict)"("DisabledEnum"=w83) -> ()  [unwired: 2 in, 2 out]
          n176 = property on="P1 CH2_selcur, A" class="DigNum (strict)"("DisabledEnum"=w83) -> ()  [unwired: 2 in, 2 out]
          n177 = property on="P1 CH2_counter" class="DigNum (strict)"("DisabledEnum"=w83) -> ()  [unwired: 2 in, 2 out]
          n178 = property on="P1 CH2_warning" class="Bool (strict)"("DisabledEnum"=w83) -> ()  [unwired: 2 in, 2 out]
        }
        frame #3 {
          w84 = T7."Disabled and Grayed Out" ("Disabled")
          n179 = property on="P2 CH0" class="Bool (strict)"("DisabledEnum"=w84) -> ()  [unwired: 2 in, 2 out]
          n180 = property on="P2 CH0_char" class="WFChart (strict)"("DisabledEnum"=w84) -> ()  [unwired: 2 in, 2 out]
          n181 = property on="P2 CH0, V" class="DigNum (strict)"("DisabledEnum"=w84) -> ()  [unwired: 2 in, 2 out]
          n182 = property on="P2 CH0_curlim, A" class="DigNum (strict)"("DisabledEnum"=w84) -> ()  [unwired: 2 in, 2 out]
          n183 = property on="P2 CH0_cur, A" class="DigNum (strict)"("DisabledEnum"=w84) -> ()  [unwired: 2 in, 2 out]
          n184 = property on="P2 CH0_selcur, A" class="DigNum (strict)"("DisabledEnum"=w84) -> ()  [unwired: 2 in, 2 out]
          n185 = property on="P2 CH0_counter" class="DigNum (strict)"("DisabledEnum"=w84) -> ()  [unwired: 2 in, 2 out]
          n186 = property on="P2 CH0_warning" class="Bool (strict)"("DisabledEnum"=w84) -> ()  [unwired: 2 in, 2 out]
        }
        frame #4 {
          w85 = T7."Disabled and Grayed Out" ("Disabled")
          n187 = property on="P2 CH1" class="Bool (strict)"("DisabledEnum"=w85) -> ()  [unwired: 2 in, 2 out]
          n188 = property on="P2 CH1_char" class="WFChart (strict)"("DisabledEnum"=w85) -> ()  [unwired: 2 in, 2 out]
          n189 = property on="P2 CH1, V" class="DigNum (strict)"("DisabledEnum"=w85) -> ()  [unwired: 2 in, 2 out]
          n190 = property on="P2 CH1_curlim, A" class="DigNum (strict)"("DisabledEnum"=w85) -> ()  [unwired: 2 in, 2 out]
          n191 = property on="P2 CH1_cur, A" class="DigNum (strict)"("DisabledEnum"=w85) -> ()  [unwired: 2 in, 2 out]
          n192 = property on="P2 CH1_selcur, A" class="DigNum (strict)"("DisabledEnum"=w85) -> ()  [unwired: 2 in, 2 out]
          n193 = property on="P2 CH1_counter" class="DigNum (strict)"("DisabledEnum"=w85) -> ()  [unwired: 2 in, 2 out]
          n194 = property on="P2 CH1_warning" class="Bool (strict)"("DisabledEnum"=w85) -> ()  [unwired: 2 in, 2 out]
        }
        frame #5 {
          w86 = T7."Disabled and Grayed Out" ("Disabled")
          n195 = property on="P2 CH2" class="Bool (strict)"("DisabledEnum"=w86) -> ()  [unwired: 2 in, 2 out]
          n196 = property on="P2 CH2_char" class="WFChart (strict)"("DisabledEnum"=w86) -> ()  [unwired: 2 in, 2 out]
          n197 = property on="P2 CH2, V" class="DigNum (strict)"("DisabledEnum"=w86) -> ()  [unwired: 2 in, 2 out]
          n198 = property on="P2 CH2_curlim, A" class="DigNum (strict)"("DisabledEnum"=w86) -> ()  [unwired: 2 in, 2 out]
          n199 = property on="P2 CH2_cur, A" class="DigNum (strict)"("DisabledEnum"=w86) -> ()  [unwired: 2 in, 2 out]
          n200 = property on="P2 CH2_selcur, A" class="DigNum (strict)"("DisabledEnum"=w86) -> ()  [unwired: 2 in, 2 out]
          n201 = property on="P2 CH2_counter" class="DigNum (strict)"("DisabledEnum"=w86) -> ()  [unwired: 2 in, 2 out]
          n202 = property on="P2 CH2_warning" class="Bool (strict)"("DisabledEnum"=w86) -> ()  [unwired: 2 in, 2 out]
        }
        frame #6 {
          w87 = T7."Enabled" ("Disabled")
          n203 = property on="P1 CH0 Used" class="Bool (strict)"("DisabledEnum"=w87) -> ()  [unwired: 2 in, 2 out]
          n204 = property on="P1 CH1 Used" class="Bool (strict)"("DisabledEnum"=w87) -> ()  [unwired: 2 in, 2 out]
          n205 = property on="P1 CH2 Used" class="Bool (strict)"("DisabledEnum"=w87) -> ()  [unwired: 2 in, 2 out]
          n206 = property on="P2 CH0 Used" class="Bool (strict)"("DisabledEnum"=w87) -> ()  [unwired: 2 in, 2 out]
          n207 = property on="P2 CH1 Used" class="Bool (strict)"("DisabledEnum"=w87) -> ()  [unwired: 2 in, 2 out]
          n208 = property on="P2 CH2 Used" class="Bool (strict)"("DisabledEnum"=w87) -> ()  [unwired: 2 in, 2 out]
          n209 = property on="Glass Meas" class="Bool (strict)"("DisabledEnum"=w87) -> ()  [unwired: 2 in, 2 out]
        }
      }
    }
    frame #2 {
      n210 = call "MultiOpto_1.4_Begin.vi"() -> ("NI DMM 3 option return"=→"NI DMM 3 Option Return":enum32{"Ampermeter button", "Ohmmeter button"}, "NI DMM 2 option return"=→"NI DMM 2 Option Return":enum32{"Ampermeter button", "Ohmmeter button"}, "NI DMM 1 option return"=→"NI DMM 1 Option Return":enum32{"Ampermeter button", "Ohmmeter button"}, "Stepper Motor Status"=→"Stepper Motor Status":bool, "Ophir 2 Status"=→"Ophir 2 Status":bool, "Текущий Образец №"=→"Образец №":string, "Ophir 1 Status"=→"Ophir 1 Status":bool, "DC Power 1 Status"=→"DC Power 1 Status":bool, "DC Power 2 Status"=→"DC Power 2 Status":bool, "DC Power 3 Status"=→"DC Power 3 Status":bool, "DC Power 4 Status"=→"DC Power 4 Status":bool, "NI DMM 1 Status"=→"NI DMM 1 Status":bool, "NI DMM 2 Status"=→"NI DMM 2 Status":bool, "NI DMM 3 Status"=→"NI DMM 3 Status":bool, "NI Scope Status"=→"NI Scope Status":bool)  [unwired: 13 in]
    }
    frame #3 {
      n211 = disable-structure shown="Disabled" {
        frame Disabled {
          n212 = local read "Образец №"() -> (w108:string)
          n213 = Build Path(base path="All Glass Path", name or relative path=w108) -> (appended path=w105:path)
          n214 = call <vilib>:"Check if File or Folder Exists.vi"("path"=w105) -> ("file or folder exists?"=w106:bool, "dup path"=w107:path)  [unwired: 8 in, 1 out]
          n215 = case shown="False" w106 {
            tunnel: w107 -> [w110 w111]
            tunnel: [w109 w111] -> w104
            frame False {
              n216 = Create Folder(path (use dialog)=w110) -> (created path=w109:path)  [unwired: 2 in, 2 out]
            }
            frame True {
            }
          }
          n217 = stacked-sequence {
            tunnel: w104 -> [w164 w194 w241]
            frame #0 {
              w162 = "\t"
              w114 = "\t"
              n218 = local read "Glass Table"() -> (w120:string[][])
              n219 = Index Array(array=w120, index (row)=4 ("disabled index (row)"), index (col)=0 ("disabled index (col)")) -> (element=w118:string)
              n220 = local read "Glass Table"() -> (w125:string[][])
              n221 = Index Array(array=w125, index (row)=3 ("disabled index (row)"), index (col)=0 ("disabled index (col)")) -> (element=w119:string)
              n222 = local read "Glass Table"() -> (w131:string[][])
              n223 = Index Array(array=w131, index (row)=2 ("disabled index (row)"), index (col)=0 ("disabled index (col)")) -> (element=w130:string)
              n224 = Build Path(base path=w164, name or relative path="Full Log") -> (appended path=w181:path)
              n225 = Get Date/Time In Seconds() -> (seconds since 1Jan1904=w177:timestamp)
              n226 = local read "Glass Table"() -> (w129:string[][])
              n227 = call <vilib>:"Check if File or Folder Exists.vi"("path"=w181) -> ("file or folder exists?"=w180:bool, "dup path"=w179:path)  [unwired: 8 in, 1 out]
              n228 = Index Array(array=w129, index (row)=1 ("disabled index (row)"), index (col)=0 ("disabled index (col)")) -> (element=w126:string)
              n229 = Format Date/Time String(time format string (%c)="Full Log %d %m %y %H.%M.%S", seconds (now)=w177) -> (date/time string=w176:string)  [unwired: 1 in]
              n230 = case shown="False" w180 {
                tunnel: w179 -> [w183 w184]
                tunnel: [w182 w184] -> w178
                frame False {
                  n231 = Create Folder(path (use dialog)=w183) -> (created path=w182:path)  [unwired: 2 in, 2 out]
                }
                frame True {
                }
              }
              n232 = Concatenate Strings(w176, ".xls" ("string")) -> (w175:string)
              n233 = Build Path(base path=w178, name or relative path=w175) -> (appended path=w174:path)
              n234 = Concatenate Strings("P1 CH0, V" ("string"), w114, "P1 CH0 Current, A" ("string"), w114, "DMM1_1" ("string"), w114, "DMM1_2" ("string"), w114, "DMM1_3" ("string"), w114, "DMM1_4" ("string"), w114, "DMM1_5" ("string"), w114, "Time" ("string"), w114, "455 nm Current Averaged, A" ("string"), w114, "P2 CH0, V" ("string"), w114, "P2 CH0 Current, A" ("string"), w114, "DMM2_1" ("string"), w114, "DMM2_2" ("string"), w114, "DMM2_3" ("string"), w114, "DMM2_4" ("string"), w114, "DMM2_5" ("string"), w114, "Time" ("string"), w114, "808 nm Current Averaged, A" ("string"), w114, "P2 CH1, V" ("string"), w114, "P2 CH2 Current, A" ("string"), w114, "DMM3_1" ("string"), w114, "DMM3_2" ("string"), w114, "DMM3_3" ("string"), w114, "DMM3_4" ("string"), w114, "DMM3_5" ("string"), w114, "Time" ("string"), w114, "1550 nm Current Averaged, A" ("string"), w114, "455 nm Absolute/Reference" ("string"), w114, "808 nm Absolute/Reference" ("string"), w114, "1550 nm Absolute/Reference" ("string"), w114) -> (w161:string)
              n235 = Open/Create/Replace File(file path (use dialog)=w174, operation (0:open)=T6."open or create", access (0:read/write)=enum16{"read/write", "read-only", "write-only"}."read/write") -> (refnum out=w173:refnum<file>)  [unwired: 3 in, 2 out]
              n236 = Set File Position(refnum=w173, from (0:start)=enum16{"start", "end", "current"}."end") -> (refnum out=w171:refnum<file>)  [unwired: 2 in, 1 out]
              n237 = Concatenate Strings(w161, w126, w162, w161, w130, w162, w161, w119, w162, w161, w118, w162, w161, "Log Remarks" ("string"), "\r\n") -> (w170:string)
              n238 = Format Into String(initial string=w171, w170) -> (resulting string=→"Glass Full Log Output File":refnum<file>)  [unwired: 2 in, 1 out]
            }
            frame #1 {
              w187 = "\t"
              n239 = Build Path(base path=w194, name or relative path="Single Measurements") -> (appended path=w236:path)
              n240 = Get Date/Time In Seconds() -> (seconds since 1Jan1904=w232:timestamp)
              n241 = call <vilib>:"Check if File or Folder Exists.vi"("path"=w236) -> ("file or folder exists?"=w235:bool, "dup path"=w234:path)  [unwired: 8 in, 1 out]
              n242 = Format Date/Time String(time format string (%c)="Single Measurements %d %m %y %H.%M.%S", seconds (now)=w232) -> (date/time string=w231:string)  [unwired: 1 in]
              n243 = case shown="False" w235 {
                tunnel: w234 -> [w238 w239]
                tunnel: [w237 w239] -> w233
                frame False {
                  n244 = Create Folder(path (use dialog)=w238) -> (created path=w237:path)  [unwired: 2 in, 2 out]
                }
                frame True {
                }
              }
              n245 = Concatenate Strings(w231, ".xls" ("string")) -> (w230:string)
              n246 = Build Path(base path=w233, name or relative path=w230) -> (appended path=w229:path)
              n247 = Concatenate Strings("P1 CH0, V" ("string"), w187, "P1 CH0 Current, A" ("string"), w187, "DMM1_1" ("string"), w187, "DMM1_2" ("string"), w187, "DMM1_3" ("string"), w187, "DMM1_4" ("string"), w187, "DMM1_5" ("string"), w187, "Time" ("string"), w187, "455 nm Current Averaged, A" ("string"), w187, "P1 CH1, V" ("string"), w187, "P1 CH1 Current, A" ("string"), w187, "DMM2_1" ("string"), w187, "DMM2_2" ("string"), w187, "DMM2_3" ("string"), w187, "DMM2_4" ("string"), w187, "DMM2_5" ("string"), w187, "Time" ("string"), w187, "808 nm Current Averaged, A" ("string"), w187, "P2 CH0, V" ("string"), w187, "P2 CH0 Current, A" ("string"), w187, "DMM3_1" ("string"), w187, "DMM3_2" ("string"), w187, "DMM3_3" ("string"), w187, "DMM3_4" ("string"), w187, "DMM3_5" ("string"), w187, "Time" ("string"), w187, "1550 nm Current Averaged, A" ("string"), w187, "455 nm Absolute/Reference" ("string"), w187, "808 nm Absolute/Reference" ("string"), w187, "1550 nm Absolute/Reference" ("string"), w187, "Log Remarks" ("string"), "\r\n") -> (w192:string)
              n248 = Open/Create/Replace File(file path (use dialog)=w229, operation (0:open)=T6."open or create", access (0:read/write)=enum16{"read/write", "read-only", "write-only"}."read/write") -> (refnum out=w228:refnum<file>)  [unwired: 3 in, 2 out]
              n249 = Set File Position(refnum=w228, from (0:start)=enum16{"start", "end", "current"}."end") -> (refnum out=w227:refnum<file>)  [unwired: 2 in, 1 out]
              n250 = Format Into String(initial string=w227, w192) -> (resulting string=→"Single Meas Output File":refnum<file>)  [unwired: 2 in, 1 out]
            }
            frame #2 {
              n251 = for {
                N: 4 -> [_]
                tunnel: w241 -> [w260]
                i -> [w252]
                w244 = "\t"
                w249 = "\t"
                n252 = local read "Glass Table"() -> (w255:string[][])
                n253 = Increment(x=w252) -> (x+1=w251:i32)
                n254 = Index Array(array=w255, index (row)=w251, index (col)=0 ("disabled index (col)")) -> (element=w254:string)
                n255 = Concatenate Strings(w254, " %d %m %y %H.%M.%S" ("time format string (%c)")) -> (w256:string)
                n256 = Build Path(base path=w260, name or relative path=w254) -> (appended path=w287:path)
                n257 = Get Date/Time In Seconds() -> (seconds since 1Jan1904=w283:timestamp)
                n258 = call <vilib>:"Check if File or Folder Exists.vi"("path"=w287) -> ("file or folder exists?"=w286:bool, "dup path"=w285:path)  [unwired: 8 in, 1 out]
                n259 = Format Date/Time String(time format string (%c)=w256, seconds (now)=w283) -> (date/time string=w282:string)  [unwired: 1 in]
                n260 = case shown="False" w286 {
                  tunnel: w285 -> [w293 w294]
                  tunnel: [w292 w294] -> w284
                  frame False {
                    n261 = Create Folder(path (use dialog)=w293) -> (created path=w292:path)  [unwired: 2 in, 2 out]
                  }
                  frame True {
                  }
                }
                n262 = Concatenate Strings("P1 CH0, V" ("string"), w249, "P1 CH0 Current, A" ("string"), w249, "Time" ("string"), w249, "455 nm Current Averaged, A" ("string"), w249, "P1 CH1, V" ("string"), w249, "P1 CH1 Current, A" ("string"), w249, "Time" ("string"), w249, "808 nm Current Averaged, A" ("string"), w249, "P2 CH0, V" ("string"), w249, "P2 CH0 Current, A" ("string"), w249, "Time" ("string"), w249, "1550 nm Current Averaged, A" ("string"), w249) -> (w250:string)
                n263 = Concatenate Strings(w282, ".xls" ("string")) -> (w281:string)
                n264 = Build Path(base path=w284, name or relative path=w281) -> (appended path=w280:path)
                n265 = Open/Create/Replace File(file path (use dialog)=w280, operation (0:open)=T6."open or create", access (0:read/write)=enum16{"read/write", "read-only", "write-only"}."read/write") -> (refnum out=w279:refnum<file>)  [unwired: 3 in, 2 out]
                n266 = Concatenate Strings(w250, "455 nm Absolute/Reference" ("string"), w244, "808 nm Absolute/Reference" ("string"), w244, "1550 nm Absolute/Reference" ("string"), w244) -> (w245:string)
                n267 = Set File Position(refnum=w279, from (0:start)=enum16{"start", "end", "current"}."end") -> (refnum out=w274:refnum<file>)  [unwired: 2 in, 1 out]
                n268 = Concatenate Strings(w245, w254, "\t", w245, "Log Remarks" ("string"), "\r\n") -> (w261:string)
                n269 = Format Into String(initial string=w274, w261) -> (resulting string=w259:refnum<file>)  [unwired: 2 in, 1 out]
                n270 = case shown="3" w252 {
                  tunnel: w259 -> [w288 w289 w290 w291]
                  frame 0, Default {
                    "Glass 1 Output File" <- w288
                  }
                  frame 1 {
                    "Glass 2 Output File" <- w289
                  }
                  frame 2 {
                    "Glass 3 Output File" <- w290
                  }
                  frame 3 {
                    "Glass 4 Output File" <- w291
                  }
                }
              }
            }
          }
        }
        frame Enabled {
        }
      }
    }
    frame #4 {
      w297 = "\t"
      # "Инициализация файла SEL"
      n271 = local read "Образец №"() -> (w324:string)
      n272 = Build Path(base path="SEL path", name or relative path=w324) -> (appended path=w339:path)
      n273 = Get Date/Time In Seconds() -> (seconds since 1Jan1904=w335:timestamp)
      n274 = call <vilib>:"Check if File or Folder Exists.vi"("path"=w339) -> ("file or folder exists?"=w338:bool, "dup path"=w337:path)  [unwired: 8 in, 1 out]
      n275 = Format Date/Time String(time format string (%c)="SEL %d %m %y %H.%M.%S", seconds (now)=w335) -> (date/time string=w334:string)  [unwired: 1 in]
      n276 = case shown="False" w338 {
        tunnel: w337 -> [w341 w342]
        tunnel: [w340 w342] -> w336
        frame False {
          n277 = Create Folder(path (use dialog)=w341) -> (created path=w340:path)  [unwired: 2 in, 2 out]
        }
        frame True {
        }
      }
      n278 = Concatenate Strings(w334, ".xls" ("string")) -> (w331:string)
      n279 = Build Path(base path=w336, name or relative path=w331) -> (appended path=w328:path)
      n280 = Open/Create/Replace File(file path (use dialog)=w328, operation (0:open)=T6."open or create", access (0:read/write)=enum16{"read/write", "read-only", "write-only"}."read/write") -> (refnum out=w327:refnum<file>)  [unwired: 3 in, 2 out]
      n281 = Set File Position(refnum=w327, from (0:start)=enum16{"start", "end", "current"}."end") -> (refnum out=w308:refnum<file>)  [unwired: 2 in, 1 out]
      n282 = Format Into String(initial string=w308, "Time" ("string"), w297, "P1 CH0, V" ("string"), w297, "P1 CH0_cur, A" ("string"), w297, "P1 CH0_counter" ("string"), w297, "!!!1_0" ("input 7"), w297, "P1 CH1, V" ("string"), w297, "P1 CH1_cur, A" ("string"), w297, "P1 CH1_counter" ("string"), w297, "!!!1_1" ("input 7"), w297, "P1 CH2, V" ("string"), w297, "P1 CH2_cur, A" ("string"), w297, "P1 CH2_counter" ("string"), w297, "!!!1_2" ("input 7"), w297, "P2 CH0, V" ("string"), w297, "P2 CH0_cur, A" ("string"), w297, "P2 CH0_counter" ("string"), w297, "!!!2_0" ("input 7"), w297, "P2 CH1, V" ("string"), w297, "P2 CH1_cur, A" ("string"), w297, "P2 CH1_counter" ("string"), w297, "!!!2_1" ("input 7"), w297, "P2 CH2, V" ("string"), w297, "P2 CH2_cur, A" ("string"), w297, "P2 CH2_counter" ("string"), w297, "!!!2_2" ("input 7"), "\r\n") -> (resulting string=→"SEL output file refnum":refnum<file>)  [unwired: 2 in, 1 out]
    }
    frame #5 {
      # "Инициализация источника"
      n283 = local read "DC Power 4 Status"() -> (w343:bool)
      n284 = case shown="True" w343 {
        tunnel: [refnum<k15> refnum ("instrument handle out") w360] -> w348
        tunnel: [errorcluster {"status"=FALSE, "code"=0, "source"=""} ("error out") w359] -> w347
        frame False {
          n285 = property on="Tab DC Power 4" class="TabCtl (strict)"("DisabledEnum"=T7."Disabled and Grayed Out" ("Disabled")) -> ()  [unwired: 2 in, 2 out]
        }
        frame True {
          n286 = call <instrlib>:"niDCPower Initialize.vi"("resource name"="DC POWER 4") -> ("error out"=w364:errorcluster, "instrument handle out"=w365:refnum<k15>)  [unwired: 3 in, 6 out]
          n287 = property on="Tab DC Power 4" class="TabCtl (strict)"("DisabledEnum"=T7."Enabled" ("Disabled")) -> ()  [unwired: 2 in, 2 out]
          n288 = call <instrlib>:"niDCPower Configure Voltage Level.vi"("error in (no error)"=w364, "voltage level"=0.0, "channel name"="0,1", "instrument handle"=w365) -> ("error out"=w359:errorcluster, "instrument handle out"=w360:refnum<k15>)  [unwired: 6 in]
        }
      }
      n289 = local read "DC Power 1 Status"() -> (w346:bool)
      n290 = local read "DC Power 2 Status"() -> (w345:bool)
      n291 = local read "DC Power 3 Status"() -> (w344:bool)
      n292 = case shown="True" w346 {
        tunnel: [refnum<k15> refnum ("instrument handle out") w382] -> w354
        tunnel: [errorcluster {"status"=FALSE, "code"=0, "source"=""} ("error out") w381] -> w353
        frame False {
          n293 = property on="Tab DC Power 1" class="TabCtl (strict)"("DisabledEnum"=T7."Disabled and Grayed Out" ("Disabled")) -> ()  [unwired: 2 in, 2 out]
        }
        frame True {
          n294 = property on="Tab DC Power 1" class="TabCtl (strict)"("DisabledEnum"=T7."Enabled" ("Disabled")) -> ()  [unwired: 2 in, 2 out]
          n295 = call <instrlib>:"niDCPower Initialize.vi"("resource name"="DC POWER 1") -> ("error out"=w386:errorcluster, "instrument handle out"=w387:refnum<k15>)  [unwired: 3 in, 6 out]
          n296 = call <instrlib>:"niDCPower Configure Voltage Level.vi"("error in (no error)"=w386, "voltage level"=0.0, "channel name"="0,1", "instrument handle"=w387) -> ("error out"=w381:errorcluster, "instrument handle out"=w382:refnum<k15>)  [unwired: 6 in]
        }
      }
      n297 = case shown="True" w345 {
        tunnel: [refnum<k15> refnum ("instrument handle out") w393] -> w351
        tunnel: [errorcluster {"status"=FALSE, "code"=0, "source"=""} ("error out") w392] -> w352
        frame False {
          n298 = property on="Tab DC Power 2" class="TabCtl (strict)"("DisabledEnum"=T7."Disabled and Grayed Out" ("Disabled")) -> ()  [unwired: 2 in, 2 out]
        }
        frame True {
          n299 = property on="Tab DC Power 2" class="TabCtl (strict)"("DisabledEnum"=T7."Enabled" ("Disabled")) -> ()  [unwired: 2 in, 2 out]
          n300 = call <instrlib>:"niDCPower Initialize.vi"("resource name"="DC POWER 2") -> ("error out"=w397:errorcluster, "instrument handle out"=w398:refnum<k15>)  [unwired: 3 in, 6 out]
          n301 = call <instrlib>:"niDCPower Configure Voltage Level.vi"("error in (no error)"=w397, "voltage level"=0.0, "channel name"="0,1", "instrument handle"=w398) -> ("error out"=w392:errorcluster, "instrument handle out"=w393:refnum<k15>)  [unwired: 6 in]
        }
      }
      n302 = case shown="True" w344 {
        tunnel: [refnum<k15> refnum ("instrument handle out") w371] -> w350
        tunnel: [errorcluster {"status"=FALSE, "code"=0, "source"=""} ("error out") w370] -> w349
        frame False {
          n303 = property on="Tab DC Power 3" class="TabCtl (strict)"("DisabledEnum"=T7."Disabled and Grayed Out" ("Disabled")) -> ()  [unwired: 2 in, 2 out]
        }
        frame True {
          n304 = call <instrlib>:"niDCPower Initialize.vi"("resource name"="DC POWER 3") -> ("error out"=w375:errorcluster, "instrument handle out"=w376:refnum<k15>)  [unwired: 3 in, 6 out]
          n305 = property on="Tab DC Power 3" class="TabCtl (strict)"("DisabledEnum"=T7."Enabled" ("Disabled")) -> ()  [unwired: 2 in, 2 out]
          n306 = call <instrlib>:"niDCPower Configure Voltage Level.vi"("error in (no error)"=w375, "voltage level"=0.0, "channel name"="0,1", "instrument handle"=w376) -> ("error out"=w370:errorcluster, "instrument handle out"=w371:refnum<k15>)  [unwired: 6 in]
        }
      }
    }
    frame #6 {
      n307 = local read "NI Scope Status"() -> (w399:bool)
      n308 = case shown="True" w399 {
        tunnel: [refnum<k15> refnum ("instrument handle out") w407] -> w401
        tunnel: [errorcluster {"status"=FALSE, "code"=0, "source"=""} ("error out") w406] -> w400
        frame False {
          n309 = Wait (ms)(milliseconds to wait=u32 1) -> ()  [unwired: 1 out]
          n310 = property on="NI Scope Tab" class="TabCtl (strict)"("DisabledEnum"=T7."Disabled and Grayed Out" ("Disabled")) -> ()  [unwired: 2 in, 2 out]
        }
        frame True {
          n311 = stacked-sequence {
            tunnel: [_ w439] -> w407
            tunnel: [_ w438] -> w406
            frame #0 {
              w418 = "\t"
              # "Инициализация файла SEU"
              n312 = local read "Образец №"() -> (w423:string)
              n313 = Build Path(base path="SEU path", name or relative path=w423) -> (appended path=w433:path)
              n314 = Get Date/Time In Seconds() -> (seconds since 1Jan1904=w429:timestamp)
              n315 = call <vilib>:"Check if File or Folder Exists.vi"("path"=w433) -> ("file or folder exists?"=w432:bool, "dup path"=w431:path)  [unwired: 8 in, 1 out]
              n316 = Format Date/Time String(time format string (%c)="SEU %d %m %y %H.%M.%S", seconds (now)=w429) -> (date/time string=w428:string)  [unwired: 1 in]
              n317 = case shown="True" w432 {
                tunnel: w431 -> [w435 w436]
                tunnel: [w434 w436] -> w430
                frame False {
                  n318 = Create Folder(path (use dialog)=w435) -> (created path=w434:path)  [unwired: 2 in, 2 out]
                }
                frame True {
                }
              }
              n319 = Concatenate Strings(w428, ".xls" ("string")) -> (w427:string)
              n320 = Build Path(base path=w430, name or relative path=w427) -> (appended path=w426:path)
              n321 = Open/Create/Replace File(file path (use dialog)=w426, operation (0:open)=T6."open or create", access (0:read/write)=enum16{"read/write", "read-only", "write-only"}."read/write") -> (refnum out=w425:refnum<file>)  [unwired: 3 in, 2 out]
              n322 = property on="NI Scope Tab" class="TabCtl (strict)"("DisabledEnum"=T7."Enabled" ("Disabled")) -> ()  [unwired: 2 in, 2 out]
              n323 = Set File Position(refnum=w425, from (0:start)=enum16{"start", "end", "current"}."end") -> (refnum out=w422:refnum<file>)  [unwired: 2 in, 1 out]
              n324 = Format Into String(initial string=w422, "Time" ("string"), w418, "Voltage, V" ("string"), w418, "Current, A" ("string"), w418, "SEU counter" ("string"), w418, "!!!" ("input 7"), "\r\n") -> (resulting string=→"SEU output file refnum":refnum<file>)  [unwired: 2 in, 1 out]
            }
            frame #1 {
              w444 = 2 items=["None"=1, "Auto Trigger"=2] ("Triggering:Trigger Modifier")
              w442 = u32 0 items=["1 mega ohm"=0, "50 ohms"=2] ("Input Impedance")
              w440 = FALSE  # Reset Device
              n325 = call <instrlib>:"niScope Initialize.vi"("resource name"="NI Scope", "reset device"=w440, "error in"="NI Scope error in") -> ("instrument handle"=w451:refnum<k15>, "error out"=w450:errorcluster)  [unwired: 11 in]
              n326 = call <instrlib>:"niScope Configure Chan Characteristics.vi"("instrument handle"=w451, "channels"="0" ("Channel Name"), "input impedance"=w442, "maximum input frequency"=20000000.0 ("Maximum Input Frequency"), "error in"=w450) -> ("instrument handle out"=w453:refnum<k15>, "error out"=w449:errorcluster)  [unwired: 9 in]
              n327 = call <instrlib>:"niScope Configure Horizontal Timing.vi"("instrument handle"=w453, "enforce realtime"=TRUE ("Enforce Realtime"), "min sample rate"=250000000.0 ("Min Sample Rate"), "reference position"=50.0 ("Reference\nPosition"), "error in"=w449, "min record length"=1000000 ("Min Record Length")) -> ("instrument handle out"=w452:refnum<k15>, "error out"=w438:errorcluster)  [unwired: 8 in]
              n328 = property on="Property Node" class="niScope"(reference=w452, "Trigger Modifier"=w444) -> (reference out=w439:refnum<k15>)  [unwired: 1 in, 1 out]
            }
          }
        }
      }
    }
    frame #7 {
      # "Инициализация DMM"
      n329 = local read "NI DMM 1 Status"() -> (w462:bool)
      n330 = local read "NI DMM 2 Status"() -> (w461:bool)
      n331 = local read "NI DMM 3 Status"() -> (w457:bool)
      n332 = case shown="True" w457 {
        tunnel: [refnum<k15> refnum ("instrument handle out") w468] -> w455
        tunnel: [errorcluster {"status"=FALSE, "code"=0, "source"=""} ("error out") w469] -> w456
        frame False {
          n333 = property on="NI DMM 3 Tab" class="TabCtl (strict)"("DisabledEnum"=T7."Disabled and Grayed Out" ("Disabled")) -> ()  [unwired: 2 in, 2 out]
        }
        frame True {
          n334 = local read "NI DMM 3 Option Return"() -> (w470:enum32{"Ampermeter button", "Ohmmeter button"})
          n335 = property on="NI DMM 3 Tab" class="TabCtl (strict)"("DisabledEnum"=T7."Enabled" ("Disabled")) -> ()  [unwired: 2 in, 2 out]
          n336 = stacked-sequence {
            tunnel: w470 -> [w471 _]
            tunnel: [_ w525] -> w469
            tunnel: [_ w524] -> w468
            frame #0 {
              n337 = case shown="\"Ampermeter button\", Default" w471 {
                frame "Ampermeter button", Default {
                  # "Инициализация файла SEU"
                  n338 = local read "Образец №"() -> (w487:string)
                  n339 = Build Path(base path="NI DMM 3 Ampermeter path", name or relative path=w487) -> (appended path=w494:path)
                  n340 = Get Date/Time In Seconds() -> (seconds since 1Jan1904=w490:timestamp)
                  n341 = call <vilib>:"Check if File or Folder Exists.vi"("path"=w494) -> ("file or folder exists?"=w493:bool, "dup path"=w492:path)  [unwired: 8 in, 1 out]
                  n342 = Format Date/Time String(time format string (%c)="NI DMM 3 %d %m %y %H.%M.%S", seconds (now)=w490) -> (date/time string=w489:string)  [unwired: 1 in]
                  n343 = case shown="True" w493 {
                    tunnel: w492 -> [w496 w497]
                    tunnel: [w495 w497] -> w491
                    frame False {
                      n344 = Create Folder(path (use dialog)=w496) -> (created path=w495:path)  [unwired: 2 in, 2 out]
                    }
                    frame True {
                    }
                  }
                  n345 = Concatenate Strings(w489, ".xls" ("string")) -> (w488:string)
                  n346 = Build Path(base path=w491, name or relative path=w488) -> (appended path=w473:path)
                  n347 = Open/Create/Replace File(file path (use dialog)=w473, operation (0:open)=T6."open or create", access (0:read/write)=enum16{"read/write", "read-only", "write-only"}."read/write") -> (refnum out=w484:refnum<file>)  [unwired: 3 in, 2 out]
                  n348 = Set File Position(refnum=w484, from (0:start)=enum16{"start", "end", "current"}."end") -> (refnum out=w476:refnum<file>)  [unwired: 2 in, 1 out]
                  n349 = Format Into String(initial string=w476, "Time" ("string"), "\t", "Current, A" ("string"), "\r\n") -> (resulting string=→"NI DMM 3 Current output file":refnum<file>)  [unwired: 2 in, 1 out]
                  n350 = local write "NI DMM 3 Tab"(enum32{"Amp", "Ohm", "System Panel"}."Amp" ("NI DMM 2 Tab")) -> ()
                }
                frame "Ohmmeter button" {
                  n351 = local read "Образец №"() -> (w513:string)
                  n352 = Build Path(base path="NI DMM 3 Ohmmeter path", name or relative path=w513) -> (appended path=w520:path)
                  n353 = Get Date/Time In Seconds() -> (seconds since 1Jan1904=w516:timestamp)
                  n354 = call <vilib>:"Check if File or Folder Exists.vi"("path"=w520) -> ("file or folder exists?"=w519:bool, "dup path"=w518:path)  [unwired: 8 in, 1 out]
                  n355 = Format Date/Time String(time format string (%c)="NI DMM 3 %d %m %y %H.%M.%S", seconds (now)=w516) -> (date/time string=w515:string)  [unwired: 1 in]
                  n356 = case shown="True" w519 {
                    tunnel: w518 -> [w522 w523]
                    tunnel: [w521 w523] -> w517
                    frame False {
                      n357 = Create Folder(path (use dialog)=w522) -> (created path=w521:path)  [unwired: 2 in, 2 out]
                    }
                    frame True {
                    }
                  }
                  n358 = Concatenate Strings(w515, ".xls" ("string")) -> (w514:string)
                  n359 = Build Path(base path=w517, name or relative path=w514) -> (appended path=w499:path)
                  n360 = Open/Create/Replace File(file path (use dialog)=w499, operation (0:open)=T6."open or create", access (0:read/write)=enum16{"read/write", "read-only", "write-only"}."read/write") -> (refnum out=w510:refnum<file>)  [unwired: 3 in, 2 out]
                  n361 = Set File Position(refnum=w510, from (0:start)=enum16{"start", "end", "current"}."end") -> (refnum out=w502:refnum<file>)  [unwired: 2 in, 1 out]
                  n362 = Format Into String(initial string=w502, "Time" ("string"), "\t", "Current, A" ("string"), "\r\n") -> (resulting string=→"NI DMM 3 Resistance output file":refnum<file>)  [unwired: 2 in, 1 out]
                  n363 = local write "NI DMM 3 Tab"(enum32{"Amp", "Ohm", "System Panel"}."Ohm" ("NI DMM 2 Tab")) -> ()
                }
              }
            }
            frame #1 {
              n364 = call <instrlib>:"niDMM Initialize.vi"("error in (no error)"="NI DMM 3 error in", "Instrument Descriptor"="NI DMM 3") -> ("error out"=w525:errorcluster, "instrument handle out"=w524:refnum<k15>)  [unwired: 8 in]
            }
          }
        }
      }
      "NI DMM 3 error out" <- w456
      n365 = case shown="True" w462 {
        tunnel: [refnum<k15> refnum ("instrument handle out") w596] -> w460
        tunnel: [errorcluster {"status"=FALSE, "code"=0, "source"=""} ("error out") w595] -> w459
        frame False {
          n366 = property on="NI DMM 1 Tab" class="TabCtl (strict)"("DisabledEnum"=T7."Disabled and Grayed Out" ("Disabled")) -> ()  [unwired: 2 in, 2 out]
        }
        frame True {
          n367 = local read "NI DMM 1 Option Return"() -> (w598:enum32{"Ampermeter button", "Ohmmeter button"})
          n368 = property on="NI DMM 1 Tab" class="TabCtl (strict)"("DisabledEnum"=T7."Enabled" ("Disabled")) -> ()  [unwired: 2 in, 2 out]
          n369 = stacked-sequence {
            tunnel: w598 -> [w599 _]
            tunnel: [_ w653] -> w596
            tunnel: [_ w652] -> w595
            frame #0 {
              n370 = case shown="\"Ampermeter button\", Default" w599 {
                frame "Ampermeter button", Default {
                  n371 = local read "Образец №"() -> (w615:string)
                  n372 = Build Path(base path="NI DMM 1 Ampermeter path", name or relative path=w615) -> (appended path=w622:path)
                  n373 = Get Date/Time In Seconds() -> (seconds since 1Jan1904=w618:timestamp)
                  n374 = call <vilib>:"Check if File or Folder Exists.vi"("path"=w622) -> ("file or folder exists?"=w621:bool, "dup path"=w620:path)  [unwired: 8 in, 1 out]
                  n375 = Format Date/Time String(time format string (%c)="NI DMM 1 %d %m %y %H.%M.%S", seconds (now)=w618) -> (date/time string=w617:string)  [unwired: 1 in]
                  n376 = case shown="True" w621 {
                    tunnel: w620 -> [w624 w625]
                    tunnel: [w623 w625] -> w619
                    frame False {
                      n377 = Create Folder(path (use dialog)=w624) -> (created path=w623:path)  [unwired: 2 in, 2 out]
                    }
                    frame True {
                    }
                  }
                  n378 = Concatenate Strings(w617, ".xls" ("string")) -> (w616:string)
                  n379 = Build Path(base path=w619, name or relative path=w616) -> (appended path=w601:path)
                  n380 = Open/Create/Replace File(file path (use dialog)=w601, operation (0:open)=T6."open or create", access (0:read/write)=enum16{"read/write", "read-only", "write-only"}."read/write") -> (refnum out=w612:refnum<file>)  [unwired: 3 in, 2 out]
                  n381 = local write "NI DMM 1 Tab"(enum32{"Amp", "Ohm", "System Panel"}."Amp" ("NI DMM 1 Tab")) -> ()
                  n382 = Set File Position(refnum=w612, from (0:start)=enum16{"start", "end", "current"}."end") -> (refnum out=w604:refnum<file>)  [unwired: 2 in, 1 out]
                  n383 = Format Into String(initial string=w604, "Time" ("string"), "\t", "Current, A" ("string"), "\r\n") -> (resulting string=→"NI DMM 1 Current output file":refnum<file>)  [unwired: 2 in, 1 out]
                }
                frame "Ohmmeter button" {
                  # "Инициализация файла SEU"
                  n384 = local read "Образец №"() -> (w641:string)
                  n385 = Build Path(base path="NI DMM 1 Ohmmeter path", name or relative path=w641) -> (appended path=w648:path)
                  n386 = Get Date/Time In Seconds() -> (seconds since 1Jan1904=w644:timestamp)
                  n387 = call <vilib>:"Check if File or Folder Exists.vi"("path"=w648) -> ("file or folder exists?"=w647:bool, "dup path"=w646:path)  [unwired: 8 in, 1 out]
                  n388 = Format Date/Time String(time format string (%c)="NI DMM 1 %d %m %y %H.%M.%S", seconds (now)=w644) -> (date/time string=w643:string)  [unwired: 1 in]
                  n389 = case shown="False" w647 {
                    tunnel: w646 -> [w650 w651]
                    tunnel: [w649 w651] -> w645
                    frame False {
                      n390 = Create Folder(path (use dialog)=w650) -> (created path=w649:path)  [unwired: 2 in, 2 out]
                    }
                    frame True {
                    }
                  }
                  n391 = Concatenate Strings(w643, ".xls" ("string")) -> (w642:string)
                  n392 = Build Path(base path=w645, name or relative path=w642) -> (appended path=w627:path)
                  n393 = Open/Create/Replace File(file path (use dialog)=w627, operation (0:open)=T6."open or create", access (0:read/write)=enum16{"read/write", "read-only", "write-only"}."read/write") -> (refnum out=w638:refnum<file>)  [unwired: 3 in, 2 out]
                  n394 = local write "NI DMM 1 Tab"(enum32{"Amp", "Ohm", "System Panel"}."Ohm" ("NI DMM 1 Tab")) -> ()
                  n395 = Set File Position(refnum=w638, from (0:start)=enum16{"start", "end", "current"}."end") -> (refnum out=w630:refnum<file>)  [unwired: 2 in, 1 out]
                  n396 = Format Into String(initial string=w630, "Time" ("string"), "\t", "Current, A" ("string"), "\r\n") -> (resulting string=→"NI DMM 1 Resistance output file":refnum<file>)  [unwired: 2 in, 1 out]
                }
              }
            }
            frame #1 {
              n397 = call <instrlib>:"niDMM Initialize.vi"("error in (no error)"="NI DMM 1 error in", "Instrument Descriptor"="NI DMM 1") -> ("error out"=w652:errorcluster, "instrument handle out"=w653:refnum<k15>)  [unwired: 8 in]
            }
          }
        }
      }
      "NI DMM 1 error out" <- w459
      n398 = case shown="True" w461 {
        tunnel: [refnum<k15> refnum ("instrument handle out") w531] -> w463
        tunnel: [errorcluster {"status"=FALSE, "code"=0, "source"=""} ("error out") w532] -> w458
        frame False {
          n399 = property on="NI DMM 2 Tab" class="TabCtl (strict)"("DisabledEnum"=T7."Disabled and Grayed Out" ("Disabled")) -> ()  [unwired: 2 in, 2 out]
        }
        frame True {
          n400 = local read "NI DMM 2 Option Return"() -> (w534:enum32{"Ampermeter button", "Ohmmeter button"})
          n401 = property on="NI DMM 2 Tab" class="TabCtl (strict)"("DisabledEnum"=T7."Enabled" ("Disabled")) -> ()  [unwired: 2 in, 2 out]
          n402 = stacked-sequence {
            tunnel: w534 -> [w535 _]
            tunnel: [_ w589] -> w532
            tunnel: [_ w588] -> w531
            frame #0 {
              n403 = case shown="\"Ampermeter button\", Default" w535 {
                frame "Ampermeter button", Default {
                  n404 = local read "Образец №"() -> (w551:string)
                  n405 = Build Path(base path="NI DMM 2 Ampermeter path", name or relative path=w551) -> (appended path=w558:path)
                  n406 = Get Date/Time In Seconds() -> (seconds since 1Jan1904=w554:timestamp)
                  n407 = call <vilib>:"Check if File or Folder Exists.vi"("path"=w558) -> ("file or folder exists?"=w557:bool, "dup path"=w556:path)  [unwired: 8 in, 1 out]
                  n408 = Format Date/Time String(time format string (%c)="NI DMM 2 %d %m %y %H.%M.%S", seconds (now)=w554) -> (date/time string=w553:string)  [unwired: 1 in]
                  n409 = case shown="True" w557 {
                    tunnel: w556 -> [w560 w561]
                    tunnel: [w559 w561] -> w555
                    frame False {
                      n410 = Create Folder(path (use dialog)=w560) -> (created path=w559:path)  [unwired: 2 in, 2 out]
                    }
                    frame True {
                    }
                  }
                  n411 = Concatenate Strings(w553, ".xls" ("string")) -> (w552:string)
                  n412 = Build Path(base path=w555, name or relative path=w552) -> (appended path=w537:path)
                  n413 = Open/Create/Replace File(file path (use dialog)=w537, operation (0:open)=T6."open or create", access (0:read/write)=enum16{"read/write", "read-only", "write-only"}."read/write") -> (refnum out=w548:refnum<file>)  [unwired: 3 in, 2 out]
                  n414 = Set File Position(refnum=w548, from (0:start)=enum16{"start", "end", "current"}."end") -> (refnum out=w540:refnum<file>)  [unwired: 2 in, 1 out]
                  n415 = Format Into String(initial string=w540, "Time" ("string"), "\t", "Current, A" ("string"), "\r\n") -> (resulting string=→"NI DMM 2 Current output file":refnum<file>)  [unwired: 2 in, 1 out]
                  n416 = local write "NI DMM 2 Tab"(enum32{"Amp", "Ohm", "System Panel"}."Amp" ("NI DMM 2 Tab")) -> ()
                }
                frame "Ohmmeter button" {
                  # "Инициализация файла SEU"
                  n417 = local read "Образец №"() -> (w577:string)
                  n418 = Build Path(base path="NI DMM 2 Ohmmeter path", name or relative path=w577) -> (appended path=w584:path)
                  n419 = Get Date/Time In Seconds() -> (seconds since 1Jan1904=w580:timestamp)
                  n420 = call <vilib>:"Check if File or Folder Exists.vi"("path"=w584) -> ("file or folder exists?"=w583:bool, "dup path"=w582:path)  [unwired: 8 in, 1 out]
                  n421 = Format Date/Time String(time format string (%c)="NI DMM 2 %d %m %y %H.%M.%S", seconds (now)=w580) -> (date/time string=w579:string)  [unwired: 1 in]
                  n422 = case shown="True" w583 {
                    tunnel: w582 -> [w586 w587]
                    tunnel: [w585 w587] -> w581
                    frame False {
                      n423 = Create Folder(path (use dialog)=w586) -> (created path=w585:path)  [unwired: 2 in, 2 out]
                    }
                    frame True {
                    }
                  }
                  n424 = Concatenate Strings(w579, ".xls" ("string")) -> (w578:string)
                  n425 = Build Path(base path=w581, name or relative path=w578) -> (appended path=w563:path)
                  n426 = Open/Create/Replace File(file path (use dialog)=w563, operation (0:open)=T6."open or create", access (0:read/write)=enum16{"read/write", "read-only", "write-only"}."read/write") -> (refnum out=w574:refnum<file>)  [unwired: 3 in, 2 out]
                  n427 = Set File Position(refnum=w574, from (0:start)=enum16{"start", "end", "current"}."end") -> (refnum out=w566:refnum<file>)  [unwired: 2 in, 1 out]
                  n428 = Format Into String(initial string=w566, "Time" ("string"), "\t", "Current, A" ("string"), "\r\n") -> (resulting string=→"NI DMM 2 Resistance output file":refnum<file>)  [unwired: 2 in, 1 out]
                  n429 = local write "NI DMM 2 Tab"(enum32{"Amp", "Ohm", "System Panel"}."Ohm" ("NI DMM 2 Tab")) -> ()
                }
              }
            }
            frame #1 {
              n430 = call <instrlib>:"niDMM Initialize.vi"("error in (no error)"="NI DMM 2 error in", "Instrument Descriptor"="NI DMM 2") -> ("error out"=w589:errorcluster, "instrument handle out"=w588:refnum<k15>)  [unwired: 8 in]
            }
          }
        }
      }
      "NI DMM 2 error out" <- w458
    }
    frame #8 {
      n431 = local read "Ophir 1 Status"() -> (w656:bool)
      n432 = case shown="True" w656 {
        frame False {
          n433 = property on="Ophir 1 Tab" class="TabCtl (strict)"("DisabledEnum"=T7."Disabled and Grayed Out" ("Disabled")) -> ()  [unwired: 2 in, 2 out]
        }
        frame True {
          n434 = call "Ophir InitCom.vi"("GPIB Address (default 10)"="Ophir 1 GPIB Address (10)", "Communication (default USB 0)"="Ophir 1 Select Communication Protocol", "USB Channel number (default 0)"="Ophir 1 usb channel", "Port Number (default 2)"="Ophir 1 Port Number (default 2)", "error in (no error)"="Ophir 1 error in (no error)", "Baud Rate (3:9600)"="Ophir 1 Baud Rate (3:9600)") -> ("dup Visa Session"=w664:refnum<visa-resource-name>, "error out"=w663:errorcluster)  [unwired: 1 out]
          n435 = call "Ophir InstrInfo.vi"("Visa Session"=w664, "error in (no error)"=w663) -> ("dup Visa Session"=w677:refnum<visa-resource-name>, "Instrument Info"=w673:string, "error out"=w675:errorcluster)
          n436 = call "Ophir HeadInfo.vi"("Visa Session"=w677, "error in (no error)"=w675) -> ("error out"=w674:errorcluster, "dup Visa Session"=w676:refnum<visa-resource-name>, "Head Info"=w672:string)  [unwired: 6 out]
          n437 = call "Ophir InfoStrings.vi"("error in (no error)"=w674, "Head Info"=w672, "Instrument Info"=w673) -> ("error out"=w671:errorcluster, "Strings Array"=w670:string[])
          n438 = property on="Ophir 1 Info" class="Ring (strict)"("Strings []"=w670) -> ()  [unwired: 2 in, 2 out]
          n439 = property on="Ophir 1 Tab" class="TabCtl (strict)"("DisabledEnum"=T7."Enabled" ("Disabled")) -> ()  [unwired: 2 in, 2 out]
          n440 = call "Ophir ConfigDevice.vi"("Visa Session"=w676, "Measure Choice (0:Power)"=u16 0, "error in (no error)"=w671) -> ("dup Visa Session"=→"Ophir 1 dup Visa Session":refnum<visa-resource-name>, "OK ?"=→"Ophir 1 Initialization":bool, "error out"=→"Ophir 1 error out":errorcluster)  [unwired: 1 out]
        }
      }
    }
    frame #9 {
      n441 = local read "Ophir 2 Status"() -> (w679:bool)
      n442 = case shown="True" w679 {
        frame False {
          n443 = property on="Ophir 2 Tab" class="TabCtl (strict)"("DisabledEnum"=T7."Disabled and Grayed Out" ("Disabled")) -> ()  [unwired: 2 in, 2 out]
        }
        frame True {
          n444 = call "Ophir InitCom.vi"("GPIB Address (default 10)"="Ophir 2 GPIB Address (10)", "Communication (default USB 0)"="Ophir 2 Select Communication Protocol", "USB Channel number (default 0)"="Ophir 2 usb channel", "Port Number (default 2)"="Ophir 2 Port Number (default 2)", "error in (no error)"="Ophir 2 error in (no error)", "Baud Rate (3:9600)"="Ophir 2 Baud Rate (3:9600)") -> ("dup Visa Session"=w687:refnum<visa-resource-name>, "error out"=w686:errorcluster)  [unwired: 1 out]
          n445 = call "Ophir InstrInfo.vi"("Visa Session"=w687, "error in (no error)"=w686) -> ("dup Visa Session"=w700:refnum<visa-resource-name>, "Instrument Info"=w696:string, "error out"=w698:errorcluster)
          n446 = call "Ophir HeadInfo.vi"("Visa Session"=w700, "error in (no error)"=w698) -> ("error out"=w697:errorcluster, "dup Visa Session"=w699:refnum<visa-resource-name>, "Head Info"=w695:string)  [unwired: 6 out]
          n447 = call "Ophir InfoStrings.vi"("error in (no error)"=w697, "Head Info"=w695, "Instrument Info"=w696) -> ("error out"=w694:errorcluster, "Strings Array"=w693:string[])
          n448 = property on="Ophir 2 Info" class="Ring (strict)"("Strings []"=w693) -> ()  [unwired: 2 in, 2 out]
          n449 = property on="Ophir 2 Tab" class="TabCtl (strict)"("DisabledEnum"=T7."Enabled" ("Disabled")) -> ()  [unwired: 2 in, 2 out]
          n450 = call "Ophir ConfigDevice.vi"("Visa Session"=w699, "Measure Choice (0:Power)"=u16 0, "error in (no error)"=w694) -> ("dup Visa Session"=→"Ophir 2 dup Visa Session":refnum<visa-resource-name>, "OK ?"=→"Ophir 2 Initialization":bool, "error out"=→"Ophir 2 error out":errorcluster)  [unwired: 1 out]
        }
      }
    }
    frame #10 {
      n451 = local read "Stepper Motor Status"() -> (w705:bool)
      n452 = case shown="True" w705 {
        tunnel: [_ w714] -> w704
        tunnel: [_ w713] -> w703
        tunnel: [_ w712] -> w702
        frame False {
          n453 = property on="Stepper Motor Control" class="TabCtl (strict)"("DisabledEnum"=T7."Disabled and Grayed Out" ("Disabled")) -> ()  [unwired: 2 in, 2 out]
          n454 = property on="Table Tab" class="TabCtl (strict)"("DisabledEnum"=T7."Disabled and Grayed Out" ("Disabled")) -> ()  [unwired: 2 in, 2 out]
        }
        frame True {
          n455 = property on="Stepper Motor Control" class="TabCtl (strict)"("DisabledEnum"=T7."Enabled" ("Disabled")) -> ()  [unwired: 2 in, 2 out]
          n456 = constructor class="NetTcpUrl"("host"="localhost", "port"=u32 8001, "urlPath"="AmateurStepperMotorInternal") -> (reference out=w725:refnum<k24>)  [unwired: 3 in, 5 out]
          n457 = constructor class="AmateurStepperMotorWcfClient"("serviceUrl"=w725) -> (reference out=w726:refnum<k24>)  [unwired: 3 in, 3 out]
          n458 = invoke class="AmateurStepperMotorWcfClient" method="RefreshParameters"(reference=w726) -> (reference out=w715:refnum<k24>)  [unwired: 2 in, 2 out]
          n459 = property on="Table Tab" class="TabCtl (strict)"("DisabledEnum"=T7."Enabled" ("Disabled")) -> ()  [unwired: 2 in, 2 out]
          n460 = property on="Glass Meas" class="Bool (strict)"("DisabledEnum"=T7."Enabled" ("Disabled")) -> ()  [unwired: 2 in, 2 out]
          n461 = property on="Погнали!" class="Bool (strict)"("DisabledEnum"=T7."Enabled" ("Disabled")) -> ()  [unwired: 2 in, 2 out]
          n462 = property class="AmateurStepperMotorWcfClient"(reference=w715, "Speed"="Speed", "StepDivisor"="StepDivisor", "StepMultiplicationFactor"="StepMultiplicationFactor", "AccelerationTime"=0.5, "DecelerationTime"=0.5, "HoldOn"=FALSE) -> (reference out=w714:refnum<k24>, "Position"=w713:dbl, "PositioningPrecision"=w712:dbl)  [unwired: 1 in, 1 out]
        }
      }
    }
    frame #11 {
      w727 = TRUE ("Boolean")
      "Ready Status" <- w727
    }
  }
  n463 = case shown="True" w34 {
    tunnel: w33 -> [_ w733]
    tunnel: w32 -> [_ w732]
    tunnel: w31 -> [_ w731]
    tunnel: w2 -> [_ _]
    frame False {
    }
    frame True {
      n464 = flat-sequence {
        frame #0 {
          n465 = local read "WL 455 Ref"() -> (w754:dbl)
          n466 = local read "WL 808 Ref"() -> (w753:dbl)
          n467 = local read "WL 1550 Ref"() -> (w752:dbl)
          n468 = while {
            shift-right: ["Save Glass Log Data"] -> _
            shift-left: FALSE ("Погнали!") -> [w764]
            shift-right: [w761] -> _
            shift-left: w754 -> [w757]
            shift-right: [w760] -> _
            shift-left: w753 -> [w758]
            shift-right: [w759] -> _
            shift-left: w752 -> [w756]
            stop <- w762 stop-if-true
            n469 = Wait (ms)(milliseconds to wait=u32 1) -> ()  [unwired: 1 out]
            n470 = Greater?(x="Save Glass Log Data", y=w764) -> (0:w765:bool)
            n471 = case shown="True" w765 {
              tunnel: [w769 w778] -> w761
              tunnel: [w768 w777] -> w760
              tunnel: [w767 w776] -> w759
              tunnel: w758 -> [w768 w775]
              tunnel: w757 -> [w769 w774]
              tunnel: w756 -> [w767 w773]
              frame False {
              }
              frame True {
                n472 = flat-sequence {
                  tunnel: w774 -> [w786]
                  tunnel: w775 -> [w785]
                  tunnel: w773 -> [w784]
                  tunnel: [w782] -> w772
                  tunnel: [w781] -> w771
                  tunnel: [w780] -> w770
                  tunnel: [w975] -> w778
                  tunnel: [w974] -> w777
                  tunnel: [w973] -> w776
                  tunnel: w772 -> [w975]
                  tunnel: w771 -> [w974]
                  tunnel: w770 -> [w973]
                  frame #0 {
                    "Save Glass Log Done" <- FALSE ("Save Glass Log Done")
                  }
                  frame #1 {
                    n473 = local read "Glass Meas Cycle Running"() -> (w787:bool)
                    n474 = case shown="True" w787 {
                      tunnel: w786 -> [w794 w839]
                      tunnel: w785 -> [w793 w838]
                      tunnel: w784 -> [w792 w837]
                      tunnel: "Set Last Meas As Ref" -> [w791 _]
                      tunnel: [w790 w839] -> w782
                      tunnel: [w789 w838] -> w781
                      tunnel: [w788 w837] -> w780
                      frame False {
                        n475 = local read "WL-i"() -> (w795:i32)
                        n476 = case shown="False" w791 {
                          tunnel: w794 -> [_ w808]
                          tunnel: w793 -> [_ w807]
                          tunnel: w792 -> [_ w806]
                          tunnel: [w805 w808] -> w790
                          tunnel: [w804 w807] -> w789
                          tunnel: [w803 w806] -> w788
                          frame False {
                            n477 = local read "WL 455"() -> (w805:dbl)
                            n478 = local read "WL 808"() -> (w804:dbl)
                            n479 = local read "WL 1550"() -> (w803:dbl)
                          }
                          frame True {
                            n480 = local write "WL 455 Ref"(w808) -> ()
                            n481 = local write "WL 808 Ref"(w807) -> ()
                            n482 = local write "WL 1550 Ref"(w806) -> ()
                          }
                        }
                        n483 = Wait (ms)(milliseconds to wait=u32 5) -> ()  [unwired: 1 out]
                        n484 = local read "Single Meas Output File"() -> (w799:refnum<file>)
                        n485 = local read "CH Data String"() -> (w800:string)
                        n486 = local read "All Cur Data String"() -> (w801:string)
                        n487 = local read "Meas Time String"() -> (w802:string)
                        n488 = local read "Av Cur Data String"() -> (w797:string)
                        n489 = case shown="0, Default" w795 {
                          tunnel: [w811 w817 w832] -> w796
                          tunnel: w797 -> [w811 w817 w826]
                          frame 0, Default {
                            n490 = local read "WL 455 Ref"() -> (w809:dbl)
                            n491 = local read "WL 455"() -> (w812:dbl)
                            n492 = Divide(x=w812, y=w809) -> (x/y=w814:dbl)
                            n493 = Number To Fractional String(number=w814, precision (6)=i16 3) -> (F-format string=w810:string)  [unwired: 2 in]
                            n494 = local write "WL 455 Absolute/Reference"(w810) -> ()
                          }
                          frame 1 {
                            n495 = local read "WL 808 Ref"() -> (w815:dbl)
                            n496 = local read "WL 808"() -> (w820:dbl)
                            n497 = Divide(x=w820, y=w815) -> (x/y=w819:dbl)
                            n498 = Number To Fractional String(number=w819, precision (6)=i16 3) -> (F-format string=w816:string)  [unwired: 2 in]
                            n499 = local write "WL 808 Absolute/Reference"(w816) -> ()
                          }
                          frame 2 {
                            w823 = "\t"
                            n500 = local read "Add Log Remark"() -> (w824:bool)
                            n501 = case shown="True" w824 {
                              tunnel: ["\r\n" w836] -> w822
                              frame False {
                              }
                              frame True {
                                n502 = local read "Log Remark"() -> (w834:string)
                                n503 = Concatenate Strings(w834, "\r\n") -> (w836:string)
                              }
                            }
                            n504 = local read "WL 455 Absolute/Reference"() -> (w828:string)
                            n505 = local read "WL 808 Absolute/Reference"() -> (w827:string)
                            n506 = local read "WL 1550 Ref"() -> (w821:dbl)
                            n507 = local read "WL 1550"() -> (w831:dbl)
                            n508 = Divide(x=w831, y=w821) -> (x/y=w830:dbl)
                            n509 = Number To Fractional String(number=w830, precision (6)=i16 3) -> (F-format string=w825:string)  [unwired: 2 in]
                            n510 = Concatenate Strings(w826, w828, w823, w827, w823, w825, w823, w822) -> (w832:string)
                            n511 = local write "WL 1550 Absolute/Reference"(w825) -> ()
                          }
                        }
                        n512 = Format Into String(initial string=w799, w800, w801, w802, w796) -> ()  [unwired: 2 in, 2 out]
                      }
                      frame True {
                        n513 = local read "WL-i"() -> (w844:i32)
                        n514 = local read "Куда едем?"() -> (w843:T1)
                        n515 = Wait (ms)(milliseconds to wait=u32 1) -> ()  [unwired: 1 out]
                        n516 = Equal?(x=w843, y=T1."Калибровка") -> (x = y?=w842:bool)
                        n517 = case shown="False" w842 {
                          tunnel: w844 -> [w845 w925]
                          tunnel: w843 -> [w846 _]
                          frame False {
                            n518 = stacked-sequence {
                              tunnel: w846 -> [w849 w886]
                              tunnel: w845 -> [w848 w887]
                              frame #0 {
                                n519 = case shown="2" w848 {
                                tunnel: [w863 w869 w881] -> w854
                                tunnel: [w860 w864 w873] -> w847
                                frame 0, Default {
                                n520 = local read "Av Cur Data String"() -> (w863:string)
                                n521 = local read "WL 455 Ref"() -> (w858:dbl)
                                n522 = local read "WL 455"() -> (w859:dbl)
                                n523 = Divide(x=w859, y=w858) -> (x/y=w862:dbl)
                                n524 = Number To Fractional String(number=w862, precision (6)=i16 3) -> (F-format string=w860:string)  [unwired: 2 in]
                                "WL 455 Absolute/Reference" <- w860
                                }
                                frame 1 {
                                n525 = local read "Av Cur Data String"() -> (w869:string)
                                n526 = local read "WL 808"() -> (w868:dbl)
                                n527 = local read "WL 808 Ref"() -> (w867:dbl)
                                n528 = Divide(x=w868, y=w867) -> (x/y=w866:dbl)
                                n529 = Number To Fractional String(number=w866, precision (6)=i16 3) -> (F-format string=w864:string)  [unwired: 2 in]
                                "WL 808 Absolute/Reference" <- w864
                                }
                                frame 2 {
                                w872 = "\t"
                                n530 = local read "Add Log Remark"() -> (w870:bool)
                                n531 = local read "Av Cur Data String"() -> (w876:string)
                                n532 = local read "WL 455 Absolute/Reference"() -> (w875:string)
                                n533 = local read "WL 808 Absolute/Reference"() -> (w874:string)
                                n534 = case shown="True" w870 {
                                tunnel: ["\r\n" w885] -> w871
                                frame False {
                                }
                                frame True {
                                n535 = local read "Log Remark"() -> (w883:string)
                                n536 = Concatenate Strings(w883, "\r\n") -> (w885:string)
                                }
                                }
                                n537 = local read "WL 1550 Ref"() -> (w879:dbl)
                                n538 = local read "WL 1550"() -> (w880:dbl)
                                n539 = Divide(x=w880, y=w879) -> (x/y=w878:dbl)
                                n540 = Number To Fractional String(number=w878, precision (6)=i16 3) -> (F-format string=w873:string)  [unwired: 2 in]
                                "WL 1550 Absolute/Reference" <- w873
                                n541 = Concatenate Strings(w876, w875, w872, w874, w872, w873, w872, w871) -> (w881:string)
                                }
                                }
                                n542 = local read "CH Data String"() -> (w857:string)
                                n543 = local read "Meas Time String"() -> (w856:string)
                                n544 = local read "Glass Meas Path"() -> (w855:refnum<file>)
                                n545 = Format Into String(initial string=w855, w857, w856, w854) -> ()  [unwired: 2 in, 2 out]
                                n546 = To Long Integer(number=w849) -> (32bit integer=w851:i32)
                                n547 = Increment(x=w848) -> (x+1=w850:i32)
                                n548 = Replace Array Subset(array="Glass Table", new element=w847, index (row)=w851, index (col)=w850) -> (w852:string[][])
                                n549 = local write "Glass Table"(w852) -> ()
                              }
                              frame #1 {
                                n550 = local read "Av Cur Data String"() -> (w889:string)
                                n551 = case shown="2" w887 {
                                tunnel: w886 -> [_ _ w904]
                                tunnel: [w894 w895 w903] -> w888
                                tunnel: w889 -> [w894 w895 w899]
                                frame 0, Default {
                                }
                                frame 1 {
                                }
                                frame 2 {
                                w896 = "\t"
                                n552 = local read "WL 1550 Absolute/Reference"() -> (w902:string)
                                n553 = local read "WL 455 Absolute/Reference"() -> (w900:string)
                                n554 = local read "WL 808 Absolute/Reference"() -> (w901:string)
                                n555 = Equal?(x=w904, y=T1."Четвертое стекло") -> (x = y?=w906:bool)
                                n556 = case shown="True" w906 {
                                tunnel: ["\t" w910] -> w905
                                frame False {
                                }
                                frame True {
                                n557 = case shown="True" "Add Log Remark" {
                                selector: "Add Log Remark" -> [_ w915]
                                tunnel: ["\r\n" w916] -> w910
                                tunnel: [w912 w914] -> w909
                                frame False {
                                n558 = local read "Add Log Remark"() -> (w912:bool)
                                }
                                frame True {
                                n559 = Not(x=w915) -> (.not. x?=w914:bool)
                                n560 = Concatenate Strings("Log Remark", "\r\n") -> (w916:string)
                                }
                                }
                                n561 = local write "Add Log Remark"(w909) -> ()
                                }
                                }
                                n562 = Concatenate Strings(w900, w896, w901, w896, w902, w896) -> (w898:string)
                                n563 = Concatenate Strings(w899, w898) -> (w897:string)
                                n564 = Concatenate Strings(w897, w905) -> (w903:string)
                                }
                                }
                                n565 = local read "Glass Full Log Output File"() -> (w892:refnum<file>)
                                n566 = local read "CH Data String"() -> (w890:string)
                                n567 = local read "All Cur Data String"() -> (w891:string)
                                n568 = local read "Meas Time String"() -> (w893:string)
                                n569 = Format Into String(initial string=w892, w890, w891, w893, w888) -> ()  [unwired: 2 in, 2 out]
                              }
                            }
                          }
                          frame True {
                            n570 = local read "CH Data String"() -> (w933:string)
                            n571 = local read "Meas Time String"() -> (w932:string)
                            n572 = local read "Glass 1 Output File"() -> (w931:refnum<file>)
                            n573 = local read "Glass 2 Output File"() -> (w930:refnum<file>)
                            n574 = local read "Glass 3 Output File"() -> (w929:refnum<file>)
                            n575 = local read "Glass 4 Output File"() -> (w928:refnum<file>)
                            n576 = local read "Glass Full Log Output File"() -> (w923:refnum<file>)
                            n577 = local read "CH Data String"() -> (w921:string)
                            n578 = local read "All Cur Data String"() -> (w922:string)
                            n579 = local read "Meas Time String"() -> (w924:string)
                            n580 = local read "Av Cur Data String"() -> (w920:string)
                            n581 = case shown="0, Default" w925 {
                              tunnel: [w937 w948 w956] -> w926
                              tunnel: w920 -> [w935 w947 w957]
                              tunnel: [w935 w947 w956] -> w919
                              frame 0, Default {
                                n582 = local read "Av Cur Data String"() -> (w937:string)
                                n583 = flat-sequence {
                                tunnel: [w938] -> w936
                                tunnel: w936 -> [w944]
                                tunnel: [w940] -> w934
                                frame #0 {
                                n584 = local read "WL 455 Ref"() -> (w938:dbl)
                                n585 = Wait (ms)(milliseconds to wait=u32 1) -> ()  [unwired: 1 out]
                                }
                                frame #1 {
                                n586 = local read "WL 455"() -> (w943:dbl)
                                "WL 455 Ref" <- w943
                                n587 = Divide(x=w944, y=w943) -> (x/y=w941:dbl)
                                n588 = Number To Fractional String(number=w941, precision (6)=i16 3) -> (F-format string=w940:string)  [unwired: 2 in]
                                }
                                }
                                n589 = local write "WL 455 Absolute/Reference"(w934) -> ()
                              }
                              frame 1 {
                                n590 = local read "Av Cur Data String"() -> (w948:string)
                                n591 = flat-sequence {
                                tunnel: [w949] -> w946
                                tunnel: w946 -> [w953]
                                tunnel: [w951] -> w945
                                frame #0 {
                                n592 = local read "WL 808 Ref"() -> (w949:dbl)
                                n593 = Wait (ms)(milliseconds to wait=u32 1) -> ()  [unwired: 1 out]
                                }
                                frame #1 {
                                n594 = local read "WL 808"() -> (w952:dbl)
                                "WL 808 Ref" <- w952
                                n595 = Divide(x=w953, y=w952) -> (x/y=w954:dbl)
                                n596 = Number To Fractional String(number=w954, precision (6)=i16 3) -> (F-format string=w951:string)  [unwired: 2 in]
                                }
                                }
                                n597 = local write "WL 808 Absolute/Reference"(w945) -> ()
                              }
                              frame 2 {
                                n598 = flat-sequence {
                                tunnel: [w959] -> w958
                                tunnel: w958 -> [w963]
                                tunnel: w957 -> [w968]
                                tunnel: [w967] -> w956
                                frame #0 {
                                n599 = local read "WL 1550 Ref"() -> (w959:dbl)
                                n600 = Wait (ms)(milliseconds to wait=u32 1) -> ()  [unwired: 1 out]
                                }
                                frame #1 {
                                n601 = local read "WL 1550"() -> (w962:dbl)
                                "WL 1550 Ref" <- w962
                                n602 = Divide(x=w963, y=w962) -> (x/y=w964:dbl)
                                n603 = Number To Fractional String(number=w964, precision (6)=i16 3) -> (F-format string=w961:string)  [unwired: 2 in]
                                n604 = local write "WL 1550 Absolute/Reference"(w961) -> ()
                                }
                                frame #2 {
                                w966 = "\t"
                                w969 = "\t"
                                n605 = local read "WL 455 Absolute/Reference"() -> (w972:string)
                                n606 = local read "WL 808 Absolute/Reference"() -> (w971:string)
                                n607 = local read "WL 1550 Absolute/Reference"() -> (w970:string)
                                n608 = Concatenate Strings(w968, w972, w969, w971, w969, w970, w966, w966) -> (w967:string)
                                }
                                }
                              }
                            }
                            n609 = Concatenate Strings(w933, w932, w926) -> (w927:string)
                            n610 = Format Into String(initial string=w931, w927) -> ()  [unwired: 2 in, 2 out]
                            n611 = Format Into String(initial string=w930, w927) -> ()  [unwired: 2 in, 2 out]
                            n612 = Format Into String(initial string=w929, w927) -> ()  [unwired: 2 in, 2 out]
                            n613 = Format Into String(initial string=w928, w927) -> ()  [unwired: 2 in, 2 out]
                            n614 = Format Into String(initial string=w923, w921, w922, w924, w919) -> ()  [unwired: 2 in, 2 out]
                          }
                        }
                      }
                    }
                  }
                  frame #2 {
                    n615 = local write "Save Glass Log Done"(TRUE ("Save Glass Log Done")) -> ()
                  }
                }
              }
            }
            n616 = local read "System Stop"() -> (w762:bool)
          }
        }
        frame #1 {
          n617 = local read "Glass Full Log Output File"() -> (w978:refnum<file>)
          n618 = local read "Glass 1 Output File"() -> (w982:refnum<file>)
          n619 = local read "Glass 2 Output File"() -> (w981:refnum<file>)
          n620 = local read "Glass 3 Output File"() -> (w980:refnum<file>)
          n621 = local read "Glass 4 Output File"() -> (w979:refnum<file>)
          n622 = local read "Single Meas Output File"() -> (w977:refnum<file>)
          n623 = Close File(refnum=w978) -> ()  [unwired: 1 in, 2 out]
          n624 = Close File(refnum=w982) -> ()  [unwired: 1 in, 2 out]
          n625 = Close File(refnum=w981) -> ()  [unwired: 1 in, 2 out]
          n626 = Close File(refnum=w980) -> ()  [unwired: 1 in, 2 out]
          n627 = Close File(refnum=w979) -> ()  [unwired: 1 in, 2 out]
          n628 = Close File(refnum=w977) -> ()  [unwired: 1 in, 2 out]
        }
      }
      n629 = while {
        stop <- w984 stop-if-true
        n630 = Wait (ms)(milliseconds to wait=u32 1) -> ()  [unwired: 1 out]
        n631 = case shown="True" "Glass Meas Cycle" {
          frame False {
          }
          frame True {
            n632 = while {
              stop <- w989 stop-if-true
              n633 = stacked-sequence {
                tunnel: [_ _ _ w1052] -> w987
                frame #0 {
                  n634 = flat-sequence {
                    tunnel: [w998] -> w993
                    tunnel: [w997] -> w990
                    tunnel: [w1001] -> w994
                    tunnel: w993 -> [w1001]
                    tunnel: [w1000] -> w991
                    tunnel: w990 -> [w1000]
                    tunnel: [w1005] -> w995
                    tunnel: w994 -> [w1005]
                    tunnel: [w1004] -> w992
                    tunnel: w991 -> [w1004]
                    tunnel: w995 -> [w1009]
                    tunnel: w992 -> [w1008]
                    frame #0 {
                      n635 = local read "P2 CH1 Used"() -> (w998:bool)
                      n636 = local read "P2 CH1"() -> (w997:bool)
                      "Glass Meas Cycle Running" <- TRUE ("Cycle Running")
                    }
                    frame #1 {
                      n637 = local write "Meas Progress Bar"(u8 0 ("Measuering Progress Bar")) -> ()
                      n638 = property on="Glass Meas" class="Bool (strict)"("DisabledEnum"=T7."Disabled and Grayed Out" ("Disabled")) -> ()  [unwired: 2 in, 2 out]
                      n639 = property on="Погнали!" class="Bool (strict)"("DisabledEnum"=T7."Disabled and Grayed Out" ("Disabled")) -> ()  [unwired: 2 in, 2 out]
                    }
                    frame #2 {
                      n640 = local write "P2 CH1 Used"(TRUE ("P1 CH0 Used")) -> ()
                      n641 = local write "P2 CH1"(TRUE ("P1 CH0")) -> ()
                    }
                    frame #3 {
                      n642 = Not(x=w1009) -> (.not. x?=w1011:bool)
                      n643 = Not(x=w1008) -> (.not. x?=w1010:bool)
                      n644 = Or(x=w1011, y=w1010) -> (x .or. y?=w1012:bool)
                      n645 = case shown="True" w1012 {
                        frame False {
                        }
                        frame True {
                          n646 = Wait (ms)(milliseconds to wait=u32 100) -> ()  [unwired: 1 out]
                        }
                      }
                    }
                  }
                }
                frame #1 {
                  n647 = for {
                    N: 5 -> [_]
                    i -> [w1015]
                    n648 = flat-sequence {
                      tunnel: w1015 -> [w1016]
                      tunnel: w1015 -> [w1025]
                      tunnel: w1015 -> [w1039]
                      frame #0 {
                        n649 = local write "Куда едем?"(w1016) -> ()
                      }
                      frame #1 {
                        n650 = local write "Погнали!"(TRUE ("Погнали!")) -> ()
                        n651 = Wait (ms)(milliseconds to wait=u32 200) -> ()  [unwired: 1 out]
                      }
                      frame #2 {
                        n652 = while {
                          stop <- w1020 stop-if-true
                          n653 = local read "System Stop"() -> (w1021:bool)
                          n654 = local read "Готово"() -> (w1022:bool)
                          n655 = Wait (ms)(milliseconds to wait=u32 1) -> ()  [unwired: 1 out]
                          n656 = Compound Arithmetic op=OR(w1022, w1021) -> (w1020:bool)
                        }
                      }
                      frame #3 {
                        n657 = local write "Погнали!"(FALSE ("Погнали!")) -> ()
                        n658 = Wait (ms)(milliseconds to wait=u32 200) -> ()  [unwired: 1 out]
                      }
                      frame #4 {
                        n659 = case shown="1" w1025 {
                          frame 0, Default {
                          }
                          frame 1 {
                            n660 = local read "Glass 1 Output File"() -> (→"Glass Num Output File":refnum<file>)
                          }
                          frame 2 {
                            n661 = local read "Glass 2 Output File"() -> (w1027:refnum<file>)
                            n662 = local write "Glass Num Output File"(w1027) -> ()
                          }
                          frame 3 {
                            n663 = local read "Glass 3 Output File"() -> (w1028:refnum<file>)
                            n664 = local write "Glass Num Output File"(w1028) -> ()
                          }
                          frame 4 {
                            n665 = local read "Glass 4 Output File"() -> (w1029:refnum<file>)
                            n666 = local write "Glass Num Output File"(w1029) -> ()
                          }
                        }
                      }
                      frame #5 {
                        n667 = local write "Glass Meas"(TRUE ("Glass Measure")) -> ()
                        n668 = Wait (ms)(milliseconds to wait=u32 50) -> ()  [unwired: 1 out]
                      }
                      frame #6 {
                        n669 = while {
                          stop <- w1035 stop-if-true
                          n670 = local read "Meas Running"() -> (w1032:bool)
                          n671 = local read "System Stop"() -> (w1036:bool)
                          n672 = Wait (ms)(milliseconds to wait=u32 1) -> ()  [unwired: 1 out]
                          n673 = Not(x=w1032) -> (.not. x?=w1033:bool)
                          n674 = Compound Arithmetic op=OR(w1033, w1036) -> (w1035:bool)
                        }
                      }
                      frame #7 {
                        n675 = local write "Glass Meas"(FALSE ("Glass Measure")) -> ()
                      }
                      frame #8 {
                        n676 = Increment(x=w1039) -> (x+1=w1040:i32)
                        n677 = Multiply(x=w1040, y=18) -> (x*y=w1041:i32)
                        n678 = To Unsigned Byte Integer(number=w1041) -> (unsigned 8bit integer=w1042:u8)
                        n679 = local write "Meas Progress Bar"(w1042) -> ()
                        n680 = Wait (ms)(milliseconds to wait=u32 100) -> ()  [unwired: 1 out]
                      }
                    }
                  }
                }
                frame #2 {
                  n681 = flat-sequence {
                    frame #0 {
                      n682 = local write "Куда едем?"(T1."Калибровка" ("Куда едем?")) -> ()
                    }
                    frame #1 {
                      n683 = local write "Погнали!"(TRUE ("Погнали!")) -> ()
                    }
                    frame #2 {
                      n684 = Wait (ms)(milliseconds to wait=u32 100) -> ()  [unwired: 1 out]
                    }
                    frame #3 {
                      n685 = local write "Погнали!"(FALSE ("Погнали!")) -> ()
                    }
                    frame #4 {
                      n686 = while {
                        stop <- w1048 stop-if-true
                        n687 = local read "System Stop"() -> (w1049:bool)
                        n688 = local read "Готово"() -> (w1050:bool)
                        n689 = Compound Arithmetic op=OR(w1050, w1049) -> (w1048:bool)
                      }
                    }
                    frame #5 {
                      n690 = Wait (ms)(milliseconds to wait=u32 200) -> ()  [unwired: 1 out]
                    }
                  }
                }
                frame #3 {
                  n691 = flat-sequence {
                    tunnel: [w1064] -> w1052
                    frame #0 {
                      n692 = local read "Glass Meas Cycle"() -> (w1053:bool)
                      n693 = case shown="False" w1053 {
                        frame False {
                          n694 = local write "P2 CH1 Used"(FALSE ("P1 CH0 Used")) -> ()
                        }
                        frame True {
                        }
                      }
                    }
                    frame #1 {
                      n695 = local read "Num of Meas"() -> (w1056:u32)
                      n696 = local read "Meas Progress Bar"() -> (w1060:u8)
                      n697 = Increment(x=w1056) -> (x+1=→"Num of Meas":u32)
                      n698 = Add(x=w1060, y=u8 10) -> (x+y=w1059:u8)
                      n699 = local write "Meas Progress Bar"(w1059) -> ()
                      n700 = Wait (ms)(milliseconds to wait=u32 100) -> ()  [unwired: 1 out]
                    }
                    frame #2 {
                      n701 = local write "Glass Meas Cycle Running"(FALSE ("Glass Meas Cycle Running")) -> ()
                      n702 = property on="Glass Meas" class="Bool (strict)"("DisabledEnum"=T7."Enabled" ("Disabled")) -> ()  [unwired: 2 in, 2 out]
                      n703 = property on="Погнали!" class="Bool (strict)"("DisabledEnum"=T7."Enabled" ("Disabled")) -> ()  [unwired: 2 in, 2 out]
                    }
                    frame #3 {
                      n704 = local read "Glass Meas Cycle"() -> (w1065:bool)
                      n705 = Not(x=w1065) -> (.not. x?=w1064:bool)
                    }
                  }
                }
              }
              n706 = Wait (ms)(milliseconds to wait=u32 1) -> ()  [unwired: 1 out]
              n707 = local read "System Stop"() -> (w988:bool)
              n708 = Or(x=w987, y=w988) -> (x .or. y?=w989:bool)
            }
          }
        }
        n709 = local read "System Stop"() -> (w984:bool)
      }
      n710 = while {
        shift-right: ["Glass Meas"] -> _
        shift-left: FALSE ("Glass Measure") -> [w1067]
        stop <- w1070 stop-if-true
        n711 = Wait (ms)(milliseconds to wait=u32 1) -> ()  [unwired: 1 out]
        n712 = Greater?(x="Glass Meas", y=w1067) -> (0:w1068:bool)
        n713 = case shown="True" w1068 {
          frame False {
          }
          frame True {
            n714 = stacked-sequence {
              frame #0 {
                n715 = flat-sequence {
                  frame #0 {
                    w1071 = T7."Disabled and Grayed Out" ("Disabled")
                    n716 = property on="P1 CH0 Used" class="Bool (strict)"("DisabledEnum"=w1071) -> ()  [unwired: 2 in, 2 out]
                    n717 = property on="P1 CH1 Used" class="Bool (strict)"("DisabledEnum"=w1071) -> ()  [unwired: 2 in, 2 out]
                    n718 = property on="P1 CH2 Used" class="Bool (strict)"("DisabledEnum"=w1071) -> ()  [unwired: 2 in, 2 out]
                    n719 = property on="P2 CH0 Used" class="Bool (strict)"("DisabledEnum"=w1071) -> ()  [unwired: 2 in, 2 out]
                    n720 = property on="P2 CH1 Used" class="Bool (strict)"("DisabledEnum"=w1071) -> ()  [unwired: 2 in, 2 out]
                    n721 = property on="P2 CH2 Used" class="Bool (strict)"("DisabledEnum"=w1071) -> ()  [unwired: 2 in, 2 out]
                    "Meas Running" <- TRUE ("Done")
                  }
                  frame #1 {
                    n722 = local write "P1 CH2 Used"(TRUE ("P1 CH0 Used")) -> ()
                    n723 = local write "P1 CH2"(TRUE ("P1 CH2")) -> ()
                    n724 = Wait (ms)(milliseconds to wait=u32 100) -> ()  [unwired: 1 out]
                  }
                }
              }
              frame #1 {
                n725 = for {
                  N: 3 -> [_]
                  i -> [w1078]
                  n726 = flat-sequence {
                    tunnel: w1078 -> [w1083]
                    tunnel: w1078 -> [w1087]
                    tunnel: w1078 -> [w1096]
                    tunnel: [w1094] -> w1077
                    tunnel: [w1114] -> w1081
                    tunnel: [w1113] -> w1080
                    tunnel: [w1112] -> w1079
                    tunnel: w1078 -> [w1110]
                    tunnel: w1077 -> [w1109]
                    tunnel: w1081 -> [w1149]
                    tunnel: w1080 -> [w1147]
                    tunnel: w1079 -> [w1138]
                    tunnel: w1078 -> [w1136]
                    tunnel: w1078 -> [w1155]
                    frame #0 {
                      n727 = case shown="0, Default" w1083 {
                        frame 0, Default {
                          n728 = local write "P1 CH0 Used"(TRUE ("P1 CH0 Used")) -> ()
                        }
                        frame 1 {
                          n729 = local write "P1 CH1 Used"(TRUE ("P1 CH0 Used")) -> ()
                        }
                        frame 2 {
                          n730 = local write "P2 CH0 Used"(TRUE ("P1 CH0 Used")) -> ()
                        }
                      }
                      n731 = Wait (ms)(milliseconds to wait=u32 100) -> ()  [unwired: 1 out]
                    }
                    frame #1 {
                      n732 = case shown="2" w1087 {
                        frame 0, Default {
                          n733 = local write "P1 CH0"(TRUE ("P1 CH0")) -> ()
                          n734 = Wait (ms)(milliseconds to wait=u32 2000) -> ()  [unwired: 1 out]
                        }
                        frame 1 {
                          n735 = local write "P1 CH1"(TRUE ("P1 CH0")) -> ()
                          n736 = Wait (ms)(milliseconds to wait=u32 2000) -> ()  [unwired: 1 out]
                        }
                        frame 2 {
                          n737 = local write "P2 CH0"(TRUE ("P1 CH0")) -> ()
                          n738 = Wait (ms)(milliseconds to wait=u32 12000) -> ()  [unwired: 1 out]
                        }
                      }
                    }
                    frame #2 {
                      w1102 = "\t"
                      w1097 = i16 12 ("precision (6)")
                      n739 = case shown="0, Default" w1096 {
                        tunnel: [w1104 w1106 w1108] -> w1101
                        tunnel: [w1103 w1105 w1107] -> w1099
                        frame 0, Default {
                          n740 = local read "P1 CH0, V"() -> (w1104:dbl)
                          n741 = local read "P1 CH0_cur, A"() -> (w1103:dbl)
                        }
                        frame 1 {
                          n742 = local read "P1 CH1_cur, A"() -> (w1105:dbl)
                          n743 = local read "P1 CH1, V"() -> (w1106:dbl)
                        }
                        frame 2 {
                          n744 = local read "P2 CH0_cur, A"() -> (w1107:dbl)
                          n745 = local read "P2 CH0, V"() -> (w1108:dbl)
                        }
                      }
                      n746 = local read "Glass Meas Cycle Running"() -> (w1094:bool)
                      n747 = Number To Fractional String(number=w1101, precision (6)=w1097) -> (F-format string=w1100:string)  [unwired: 2 in]
                      n748 = Number To Fractional String(number=w1099, precision (6)=w1097) -> (F-format string=w1098:string)  [unwired: 2 in]
                      n749 = Concatenate Strings(w1100, w1102, w1098, w1102) -> (→"CH Data String":string)
                    }
                    frame #3 {
                      w1113 = 5
                      n750 = for {
                        N: w1113 -> [_]
                        shift-right: [w1130] -> w1112
                        shift-left: "" -> [w1129]
                        shift-right: [w1126] -> w1114
                        shift-left: 0.0 -> [w1124]
                        tunnel: w1110 -> [w1123]
                        n751 = case shown="0, Default" w1123 {
                          tunnel: [w1132 w1133 w1134] -> w1125
                          frame 0, Default {
                            n752 = local read "DMM 1 Real Current"() -> (w1132:dbl)
                          }
                          frame 1 {
                            n753 = local read "DMM 2 Real Current"() -> (w1133:dbl)
                          }
                          frame 2 {
                            n754 = local read "DMM 3 Real Current"() -> (w1134:dbl)
                          }
                        }
                        n755 = Wait (ms)(milliseconds to wait="Meas Wait") -> ()  [unwired: 1 out]
                        n756 = Add(x=w1124, y=w1125) -> (x+y=w1126:dbl)
                        n757 = Number To Fractional String(number=w1125, precision (6)=i16 12) -> (F-format string=w1128:string)  [unwired: 2 in]
                        n758 = Concatenate Strings(w1129, w1128, "\t") -> (w1130:string)
                      }
                      n759 = case shown="False" w1109 {
                        tunnel: w1110 -> [w1116 _]
                        frame False {
                          n760 = local read "Set Last Meas As Ref"() -> (w1117:bool)
                          n761 = case shown="False" w1117 {
                            tunnel: w1116 -> [w1118 _]
                            frame False {
                              n762 = case shown="0, Default" w1118 {
                                frame 0, Default {
                                n763 = local read "WL 455"() -> (w1119:dbl)
                                n764 = local write "WL 455 Ref"(w1119) -> ()
                                }
                                frame 1 {
                                n765 = local read "WL 808"() -> (w1120:dbl)
                                n766 = local write "WL 808 Ref"(w1120) -> ()
                                }
                                frame 2 {
                                n767 = local read "WL 1550"() -> (w1121:dbl)
                                n768 = local write "WL 1550 Ref"(w1121) -> ()
                                }
                              }
                            }
                            frame True {
                            }
                          }
                        }
                        frame True {
                        }
                      }
                    }
                    frame #4 {
                      n769 = local read "Glass Meas Cycle Running"() -> (w1137:bool)
                      n770 = To Double Precision Float(number=w1147) -> (double precision float=w1148:dbl)
                      n771 = Divide(x=w1149, y=w1148) -> (x/y=w1146:dbl)
                      n772 = Wait (ms)(milliseconds to wait=u32 1) -> ()  [unwired: 1 out]
                      n773 = Number To Fractional String(number=w1146, precision (6)=i16 12) -> (F-format string=w1141:string)  [unwired: 2 in]
                      n774 = case shown="2" w1136 {
                        tunnel: w1146 -> [w1151 w1152 w1153]
                        frame 0, Default {
                          "WL 455" <- w1151
                        }
                        frame 1 {
                          "WL 808" <- w1152
                        }
                        frame 2 {
                          "WL 1550" <- w1153
                        }
                      }
                      n775 = case shown="True" w1137 {
                        frame False {
                        }
                        frame True {
                          n776 = local read "Glass Num Output File"() -> (→"Glass Meas Path":refnum<file>)
                        }
                      }
                      n777 = Concatenate Strings(w1141, "\t") -> (→"Av Cur Data String":string)
                      n778 = Format Date/Time String(time format string (%c)="%H:%M:%S:%3u") -> (date/time string=w1144:string)  [unwired: 2 in]
                      n779 = Concatenate Strings(w1144, "\t") -> (→"Meas Time String":string)
                      "All Cur Data String" <- w1138
                    }
                    frame #5 {
                      n780 = case shown="0, Default" w1155 {
                        frame 0, Default {
                          n781 = local write "P1 CH0 Used"(FALSE ("P1 CH0 Used")) -> ()
                        }
                        frame 1 {
                          n782 = local write "P1 CH1 Used"(FALSE ("P1 CH0 Used")) -> ()
                        }
                        frame 2 {
                          n783 = local write "P2 CH0 Used"(FALSE ("P1 CH0 Used")) -> ()
                        }
                      }
                      n784 = Wait (ms)(milliseconds to wait=u32 500) -> ()  [unwired: 1 out]
                    }
                    frame #6 {
                      n785 = local write "Save Glass Log Data"(TRUE ("Save Glass Log Data")) -> ()
                      n786 = Wait (ms)(milliseconds to wait=u32 50) -> ()  [unwired: 1 out]
                    }
                    frame #7 {
                      n787 = while {
                        stop <- w1163 stop-if-true
                        n788 = local read "System Stop"() -> (w1164:bool)
                        n789 = local read "Save Glass Log Done"() -> (w1165:bool)
                        n790 = Wait (ms)(milliseconds to wait=u32 1) -> ()  [unwired: 1 out]
                        n791 = Compound Arithmetic op=OR(w1165, w1164) -> (w1163:bool)
                      }
                    }
                    frame #8 {
                      n792 = local write "Save Glass Log Data"(FALSE ("Save Glass Log Data")) -> ()
                    }
                  }
                  "WL-i" <- w1078
                }
              }
              frame #2 {
                n793 = flat-sequence {
                  frame #0 {
                    n794 = local write "P1 CH2 Used"(FALSE ("P1 CH0 Used")) -> ()
                    n795 = Wait (ms)(milliseconds to wait=u32 100) -> ()  [unwired: 1 out]
                  }
                  frame #1 {
                    w1169 = T7."Enabled" ("Disabled")
                    n796 = local write "Meas Running"(FALSE ("Done")) -> ()
                    n797 = property on="P1 CH0 Used" class="Bool (strict)"("DisabledEnum"=w1169) -> ()  [unwired: 2 in, 2 out]
                    n798 = property on="P1 CH1 Used" class="Bool (strict)"("DisabledEnum"=w1169) -> ()  [unwired: 2 in, 2 out]
                    n799 = property on="P1 CH2 Used" class="Bool (strict)"("DisabledEnum"=w1169) -> ()  [unwired: 2 in, 2 out]
                    n800 = property on="P2 CH0 Used" class="Bool (strict)"("DisabledEnum"=w1169) -> ()  [unwired: 2 in, 2 out]
                    n801 = property on="P2 CH1 Used" class="Bool (strict)"("DisabledEnum"=w1169) -> ()  [unwired: 2 in, 2 out]
                    n802 = property on="P2 CH2 Used" class="Bool (strict)"("DisabledEnum"=w1169) -> ()  [unwired: 2 in, 2 out]
                  }
                }
              }
            }
          }
        }
        n803 = local read "System Stop"() -> (w1070:bool)
      }
      n804 = while {
        tunnel: w733 -> [w1217]
        shift-right: [w1207] -> _
        shift-left: FALSE ("Погнали!") -> [w1218]
        tunnel: [w1216] -> w734
        shift-right: [w1214] -> _
        shift-left: w732 -> [w1215]
        tunnel: w731 -> [w1213]
        stop <- w1210 stop-if-true
        n805 = Wait (ms)(milliseconds to wait=u32 1) -> ()  [unwired: 1 out]
        n806 = case shown="True" "Погнали!" {
          selector: "Погнали!" -> [w1219 _]
          tunnel: [w1219 w1220] -> w1207
          frame False {
          }
          frame True {
            n807 = local read "P2 CH1"() -> (w1221:bool)
            n808 = case shown="True" w1221 {
              selector: w1221 -> [_ w1225]
              tunnel: [w1222 w1225] -> w1220
              frame False {
                n809 = One Button Dialog(message="Power up the stepper motor.") -> (true=w1223:bool)  [unwired: 1 in]
                n810 = Not(x=w1223) -> (.not. x?=w1222:bool)
                n811 = local write "Погнали!"(w1222) -> ()
              }
              frame True {
              }
            }
          }
        }
        n812 = local read "System Stop"() -> (w1210:bool)
        n813 = case shown="\"Первое стекло\"" "Куда едем?" {
          tunnel: [0.0 -1550.0 -2700.0 -4100.0 -5250.0] -> w1211
          frame "Калибровка", Default {
          }
          frame "Первое стекло" {
          }
          frame "Второе стекло" {
          }
          frame "Третье стекло" {
          }
          frame "Четвертое стекло" {
          }
        }
        n814 = Greater?(x=w1207, y=w1218) -> (0:w1206:bool)
        n815 = case shown="True" w1206 {
          tunnel: w1211 -> [_ w1238]
          tunnel: w1217 -> [w1232 w1237]
          tunnel: [w1232 w1236] -> w1216
          tunnel: w1215 -> [w1231 _]
          tunnel: [w1231 w1235] -> w1214
          tunnel: w1213 -> [_ w1234]
          frame False {
            n816 = Wait (ms)(milliseconds to wait=u32 1) -> ()  [unwired: 1 out]
            "Текущая позиция" <- w1231
          }
          frame True {
            n817 = while {
              tunnel: w1238 -> [w1243]
              tunnel: w1237 -> [w1246]
              tunnel: [w1240] -> w1236
              tunnel: [w1245] -> w1235
              tunnel: w1234 -> [w1242]
              stop <- w1244 stop-if-true
              n818 = invoke class="AmateurStepperMotorWcfClient" method="GoTo"(reference=w1246, "destinationPosition"=w1243) -> (reference out=w1248:refnum<k24>, "GoTo"=w1249:refnum<k24>)  [unwired: 2 in, 2 out]
              n819 = invoke class="Task" method="ConfigureAwait"(reference=w1249, "continueOnCapturedContext"=FALSE) -> ()  [unwired: 2 in, 4 out]
              n820 = Wait (ms)(milliseconds to wait=u32 1) -> ()  [unwired: 1 out]
              n821 = while {
                tunnel: [w1252] -> w1245
                tunnel: w1248 -> [w1260]
                tunnel: [w1259] -> w1241
                tunnel: [w1251] -> w1244
                tunnel: w1243 -> [w1257]
                tunnel: w1242 -> [w1255]
                stop <- w1251 stop-if-true
                n822 = property class="AmateurStepperMotorWcfClient"(reference=w1260) -> (reference out=w1259:refnum<k24>, "Position"=w1252:dbl)  [unwired: 1 in, 1 out]
                n823 = Subtract(x=w1252, y=w1257) -> (x-y=w1258:dbl)
                n824 = Wait (ms)(milliseconds to wait=u32 1) -> ()  [unwired: 1 out]
                n825 = Absolute Value(x=w1258) -> (abs(x)=w1256:dbl)
                n826 = Less Or Equal?(x=w1256, y=w1255) -> (x <= y?=w1254:bool)
                n827 = local write "Текущая позиция"(w1252) -> ()
                n828 = Or(x=w1254, y="Стоп GoTo") -> (x .or. y?=w1251:bool)
                "Готово" <- w1251
              }
              n829 = invoke class="AmateurStepperMotorWcfClient" method="Stop"(reference=w1241) -> (reference out=w1240:refnum<k24>)  [unwired: 2 in, 2 out]
            }
          }
        }
      }
      n830 = while {
        stop <- w740 stop-if-true
        n831 = Wait (ms)(milliseconds to wait=u32 1) -> ()  [unwired: 1 out]
        n832 = case shown="True" "Clear Table" {
          frame False {
          }
          frame True {
            n833 = for {
              N: 4 -> [_]
              i -> [w743]
              n834 = for {
                N: 3 -> [_]
                tunnel: w743 -> [w745]
                i -> [w748]
                n835 = Increment(x=w745) -> (x+1=w746:i32)
                n836 = local read "Glass Table"() -> (w750:string[][])
                n837 = Increment(x=w748) -> (x+1=w747:i32)
                n838 = Replace Array Subset(array=w750, new element="" ("new element/subarray"), index (row)=w746, index (col)=w747) -> (w749:string[][])
                n839 = local write "Glass Table"(w749) -> ()
              }
            }
          }
        }
        n840 = local read "System Stop"() -> (w740:bool)
      }
      n841 = while {
        shift-right: [w1171] -> _
        shift-left: 0 ("t") -> [w1172]
        stop <- w1175 stop-if-true
        n842 = Wait (ms)(milliseconds to wait=u32 5) -> ()  [unwired: 1 out]
        n843 = case shown="True" "Тест" {
          tunnel: w1172 -> [w1178 w1185]
          tunnel: [w1178 w1182] -> w1171
          frame False {
          }
          frame True {
            n844 = flat-sequence {
              tunnel: w1185 -> [w1187]
              tunnel: [w1186] -> w1180
              tunnel: [w1192] -> w1181
              tunnel: w1180 -> [w1192]
              tunnel: [w1194] -> w1183
              tunnel: w1181 -> [w1194]
              tunnel: [w1195] -> w1184
              tunnel: w1183 -> [w1195]
              tunnel: w1184 -> [w1200]
              tunnel: [w1198] -> w1179
              tunnel: [w1205] -> w1182
              tunnel: w1179 -> [w1205]
              frame #0 {
                n845 = while {
                  tunnel: w1187 -> [w1190]
                  tunnel: [w1190] -> w1186
                  stop <- w1189 stop-if-true
                  n846 = local read "Готово"() -> (w1189:bool)
                  n847 = Wait (ms)(milliseconds to wait=u32 1) -> ()  [unwired: 1 out]
                }
              }
              frame #1 {
                n848 = local write "Куда едем?"(w1192) -> ()
                n849 = Wait (ms)(milliseconds to wait=u32 500) -> ()  [unwired: 1 out]
              }
              frame #2 {
                n850 = local write "Погнали!"(TRUE ("Погнали!")) -> ()
              }
              frame #3 {
                n851 = Wait (ms)(milliseconds to wait=u32 50) -> ()  [unwired: 1 out]
              }
              frame #4 {
                n852 = local write "Погнали!"(FALSE ("Погнали!")) -> ()
                n853 = Equal?(x=4, y=w1200) -> (x = y?=w1202:bool)
                n854 = Increment(x=w1200) -> (x+1=w1199:i32)
                n855 = Select(t=0, s=w1202, f=w1199) -> (s? t:f=w1198:i32)
              }
              frame #5 {
                n856 = Wait (ms)(milliseconds to wait=u32 50) -> ()  [unwired: 1 out]
              }
            }
          }
        }
        n857 = local read "System Stop"() -> (w1174:bool)
        n858 = Or(x=w1174, y="Стоп_тест") -> (x .or. y?=w1175:bool)
      }
      n859 = invoke class="AmateurStepperMotorWcfClient" method="Stop"(reference=w734) -> (reference out=w737:refnum<k24>, "Stop"=w738:refnum<k24>)  [unwired: 2 in, 1 out]
      n860 = invoke class="Task" method="Wait"(reference=w738) -> ()  [unwired: 2 in, 3 out]
      n861 = property class="AmateurStepperMotorWcfClient"(reference=w737, "HoldOn"=FALSE) -> (reference out=w736:refnum<k24>)  [unwired: 1 in, 1 out]
      n862 = invoke class="AmateurStepperMotorWcfClient" method="Dispose"(reference=w736) -> ()  [unwired: 2 in, 3 out]
    }
  }
  n863 = case shown="True" w40 {
    tunnel: w46 -> [_ w1267]
    tunnel: w2 -> [_ _]
    tunnel: w43 -> [_ w1264]
    frame False {
    }
    frame True {
      n864 = local read "NI DMM 1 Option Return"() -> (w1261:enum32{"Ampermeter button", "Ohmmeter button"})
      n865 = case shown="\"Ohmmeter button\"" w1261 {
        tunnel: w1267 -> [w1272 w1318]
        tunnel: [w1271 w1317] -> w1266
        tunnel: [w1270 w1316] -> w1265
        tunnel: w1264 -> [w1269 w1319]
        tunnel: [w1268 w1315] -> w1263
        frame "Ampermeter button", Default {
          n866 = while {
            tunnel: w1272 -> [w1284]
            tunnel: [w1282] -> w1271
            tunnel: [w1281] -> w1270
            tunnel: w1269 -> [w1279]
            tunnel: [w1275] -> w1268
            stop <- w1280 stop-if-true
            n867 = flat-sequence {
              tunnel: [w1290] -> w1285
              tunnel: w1284 -> [w1288]
              tunnel: w1279 -> [w1292]
              tunnel: [w1289] -> w1278
              tunnel: w1285 -> [w1295]
              tunnel: [w1300] -> w1283
              tunnel: w1278 -> [w1299]
              tunnel: [w1298] -> w1277
              tunnel: [w1294] -> w1273
              tunnel: w1283 -> [w1305]
              tunnel: [w1306] -> w1282
              tunnel: [w1305] -> w1281
              tunnel: [w1304] -> w1280
              tunnel: w1277 -> [w1303]
              tunnel: [w1303] -> w1276
              tunnel: w1273 -> [w1302]
              frame #0 {
                w1286 = T9 6.5 items=["3 1/2"=3.5, "4 1/2"=4.5, "5 1/2"=5.5, "6 1/2"=6.5, "7 1/2"=7.5] ("Resolution in Digits")
                n868 = Fract/Exp String To Number(string="NI DMM 1 Current Range") -> (number=w1291:dbl)  [unwired: 3 in, 1 out]
                n869 = call-poly <instrlib>:"niDMM Config Measurement.vi"("Range"=w1291, "Resolution in Digits"=w1286, "error in (no error)"=w1292, "Function"=niDMM_Function."DC Current" ("Measurement Type"), "instrument handle"=w1288) -> ("error out"=w1289:errorcluster, "instrument handle out"=w1290:refnum<k15>)  [unwired: 5 in]
              }
              frame #1 {
                n870 = call <instrlib>:"niDMM Read.vi"("error in (no error)"=w1299, "instrument handle"=w1295) -> ("error out"=w1298:errorcluster, "Measurement"=w1294:dbl, "instrument handle out"=w1300:refnum<k15>)  [unwired: 7 in]
                "DMM 1 Real Current" <- w1294
                n871 = Fract/Exp String To Number(string="NI DMM 1 units") -> (number=w1296:dbl)  [unwired: 3 in, 1 out]
                n872 = Multiply(x=w1296, y=w1294) -> (x*y=→"NI DMM 1 Current" →"NI DMM 1 Current Char":dbl)
              }
              frame #2 {
                w1314 = 15
                n873 = local read "NI DMM 1 Current output file"() -> (w1307:refnum<file>)
                n874 = Format Date/Time String(time format string (%c)="%H:%M:%S:%3u") -> (date/time string=w1312:string)  [unwired: 2 in]
                n875 = Number To Fractional String(number=w1302, width (-)=w1314, precision (6)=w1314) -> (F-format string=w1309:string)  [unwired: 1 in]
                n876 = local read "System Stop"() -> (w1304:bool)
                n877 = Concatenate Strings(w1312, "\t", w1309, "\r\n") -> (w1310:string)
                n878 = Format Into String(initial string=w1307, w1310) -> (resulting string=w1306:refnum<file>)  [unwired: 2 in, 1 out]
              }
            }
            n879 = Wait (ms)(milliseconds to wait="NI DMM 1 Current Wait") -> ()  [unwired: 1 out]
            n880 = call <vilib>:"Simple Error Handler.vi"("error in (no error)"=w1276) -> ("error out"=w1275:errorcluster)  [unwired: 1 in, 7 out]
          }
        }
        frame "Ohmmeter button" {
          n881 = while {
            tunnel: w1318 -> [w1331]
            tunnel: [w1329] -> w1317
            tunnel: [w1328] -> w1316
            tunnel: w1319 -> [w1326]
            tunnel: [w1322] -> w1315
            stop <- w1327 stop-if-true
            n882 = flat-sequence {
              tunnel: [w1338] -> w1332
              tunnel: w1331 -> [w1337]
              tunnel: w1326 -> [w1336]
              tunnel: [w1335] -> w1325
              tunnel: w1332 -> [w1348]
              tunnel: [w1346] -> w1330
              tunnel: w1325 -> [w1345]
              tunnel: [w1344] -> w1324
              tunnel: [w1341] -> w1320
              tunnel: w1330 -> [w1353]
              tunnel: [w1354] -> w1329
              tunnel: [w1353] -> w1328
              tunnel: [w1352] -> w1327
              tunnel: [w1351] -> w1323
              tunnel: w1324 -> [w1351]
              tunnel: w1320 -> [w1350]
              frame #0 {
                w1340 = T9 6.5 items=["3 1/2"=3.5, "4 1/2"=4.5, "5 1/2"=5.5, "6 1/2"=6.5, "7 1/2"=7.5] ("Resolution in Digits")
                n883 = Fract/Exp String To Number(string="NI DMM 1 Resistance Range") -> (number=w1333:dbl)  [unwired: 3 in, 1 out]
                n884 = call-poly <instrlib>:"niDMM Config Measurement.vi"("Range"=w1333, "Resolution in Digits"=w1340, "error in (no error)"=w1336, "Function"=niDMM_Function."2-wire Resistance" ("Measurement Type"), "instrument handle"=w1337) -> ("error out"=w1335:errorcluster, "instrument handle out"=w1338:refnum<k15>)  [unwired: 5 in]
              }
              frame #1 {
                n885 = call <instrlib>:"niDMM Read.vi"("error in (no error)"=w1345, "instrument handle"=w1348) -> ("error out"=w1344:errorcluster, "Measurement"=w1341:dbl, "instrument handle out"=w1346:refnum<k15>)  [unwired: 7 in]
                n886 = Fract/Exp String To Number(string="NI DMM 1 Resistance units") -> (number=w1342:dbl)  [unwired: 3 in, 1 out]
                n887 = Multiply(x=w1342, y=w1341) -> (x*y=→"NI DMM 1 Resistance" →"NI DMM 1 Resistance Char":dbl)
              }
              frame #2 {
                w1355 = 15
                n888 = local read "NI DMM 1 Resistance output file"() -> (w1361:refnum<file>)
                n889 = Format Date/Time String(time format string (%c)="%H:%M:%S:%3u") -> (date/time string=w1357:string)  [unwired: 2 in]
                n890 = Number To Fractional String(number=w1350, width (-)=w1355, precision (6)=w1355) -> (F-format string=w1349:string)  [unwired: 1 in]
                n891 = Concatenate Strings(w1357, "\t", w1349, "\r\n") -> (w1359:string)
                n892 = local read "System Stop"() -> (w1352:bool)
                n893 = Format Into String(initial string=w1361, w1359) -> (resulting string=w1354:refnum<file>)  [unwired: 2 in, 1 out]
              }
            }
            n894 = Wait (ms)(milliseconds to wait="NI DMM 1 Resistance Wait") -> ()  [unwired: 1 out]
            n895 = call <vilib>:"Simple Error Handler.vi"("error in (no error)"=w1323) -> ("error out"=w1322:errorcluster)  [unwired: 1 in, 7 out]
          }
        }
      }
      n896 = call <instrlib>:"niDMM Close.vi"("error in (no error)"=w1263, "instrument handle"=w1265) -> ("error out"=w1262:errorcluster)  [unwired: 9 in]
      n897 = local write "NI DMM 1 error out"(w1262) -> ()
      n898 = Close File(refnum=w1266) -> ()  [unwired: 1 in, 2 out]
      n899 = call <vilib>:"Simple Error Handler.vi"("error in (no error)"=w1262) -> ()  [unwired: 1 in, 8 out]
    }
  }
  n900 = case shown="True" w39 {
    tunnel: w45 -> [_ w1368]
    tunnel: w2 -> [_ _]
    tunnel: w42 -> [_ w1365]
    frame False {
    }
    frame True {
      n901 = local read "NI DMM 2 Option Return"() -> (w1362:enum32{"Ampermeter button", "Ohmmeter button"})
      n902 = case shown="\"Ohmmeter button\"" w1362 {
        tunnel: w1368 -> [w1373 w1420]
        tunnel: [w1372 w1418] -> w1367
        tunnel: [w1371 w1417] -> w1366
        tunnel: w1365 -> [w1370 w1419]
        tunnel: [w1369 w1416] -> w1364
        frame "Ampermeter button", Default {
          n903 = while {
            tunnel: w1373 -> [w1385]
            tunnel: [w1383] -> w1372
            tunnel: [w1382] -> w1371
            tunnel: w1370 -> [w1380]
            tunnel: [w1376] -> w1369
            stop <- w1381 stop-if-true
            n904 = flat-sequence {
              tunnel: [w1389] -> w1386
              tunnel: w1385 -> [w1387]
              tunnel: w1380 -> [w1393]
              tunnel: [w1388] -> w1379
              tunnel: w1386 -> [w1396]
              tunnel: [w1401] -> w1384
              tunnel: w1379 -> [w1400]
              tunnel: [w1399] -> w1378
              tunnel: [w1395] -> w1374
              tunnel: w1384 -> [w1406]
              tunnel: [w1407] -> w1383
              tunnel: [w1406] -> w1382
              tunnel: [w1405] -> w1381
              tunnel: [w1404] -> w1377
              tunnel: w1378 -> [w1404]
              tunnel: w1374 -> [w1403]
              frame #0 {
                w1390 = T9 6.5 items=["3 1/2"=3.5, "4 1/2"=4.5, "5 1/2"=5.5, "6 1/2"=6.5, "7 1/2"=7.5] ("Resolution in Digits")
                n905 = Fract/Exp String To Number(string="NI DMM 2 Current Range") -> (number=w1392:dbl)  [unwired: 3 in, 1 out]
                n906 = call-poly <instrlib>:"niDMM Config Measurement.vi"("Range"=w1392, "Resolution in Digits"=w1390, "error in (no error)"=w1393, "Function"=niDMM_Function."DC Current" ("Measurement Type"), "instrument handle"=w1387) -> ("error out"=w1388:errorcluster, "instrument handle out"=w1389:refnum<k15>)  [unwired: 5 in]
              }
              frame #1 {
                n907 = call <instrlib>:"niDMM Read.vi"("error in (no error)"=w1400, "instrument handle"=w1396) -> ("error out"=w1399:errorcluster, "Measurement"=w1395:dbl, "instrument handle out"=w1401:refnum<k15>)  [unwired: 7 in]
                "DMM 2 Real Current" <- w1395
                n908 = Fract/Exp String To Number(string="NI DMM 2 units") -> (number=w1397:dbl)  [unwired: 3 in, 1 out]
                n909 = Multiply(x=w1397, y=w1395) -> (x*y=→"NI DMM 2 Current" →"NI DMM 2 Current Char":dbl)
              }
              frame #2 {
                w1408 = 15
                n910 = local read "NI DMM 2 Current output file"() -> (w1415:refnum<file>)
                n911 = Format Date/Time String(time format string (%c)="%H:%M:%S:%3u") -> (date/time string=w1410:string)  [unwired: 2 in]
                n912 = Number To Fractional String(number=w1403, width (-)=w1408, precision (6)=w1408) -> (F-format string=w1413:string)  [unwired: 1 in]
                n913 = local read "System Stop"() -> (w1405:bool)
                n914 = Concatenate Strings(w1410, "\t", w1413, "\r\n") -> (w1412:string)
                n915 = Format Into String(initial string=w1415, w1412) -> (resulting string=w1407:refnum<file>)  [unwired: 2 in, 1 out]
              }
            }
            n916 = Wait (ms)(milliseconds to wait="NI DMM 2 Current Wait") -> ()  [unwired: 1 out]
            n917 = call <vilib>:"Simple Error Handler.vi"("error in (no error)"=w1377) -> ("error out"=w1376:errorcluster)  [unwired: 1 in, 7 out]
          }
        }
        frame "Ohmmeter button" {
          n918 = while {
            tunnel: w1420 -> [w1432]
            tunnel: [w1430] -> w1418
            tunnel: [w1429] -> w1417
            tunnel: w1419 -> [w1427]
            tunnel: [w1423] -> w1416
            stop <- w1428 stop-if-true
            n919 = flat-sequence {
              tunnel: [w1439] -> w1433
              tunnel: w1432 -> [w1438]
              tunnel: w1427 -> [w1437]
              tunnel: [w1436] -> w1426
              tunnel: w1433 -> [w1444]
              tunnel: [w1443] -> w1431
              tunnel: w1426 -> [w1448]
              tunnel: [w1447] -> w1425
              tunnel: [w1442] -> w1421
              tunnel: w1431 -> [w1454]
              tunnel: [w1455] -> w1430
              tunnel: [w1454] -> w1429
              tunnel: [w1453] -> w1428
              tunnel: [w1452] -> w1424
              tunnel: w1425 -> [w1452]
              tunnel: w1421 -> [w1451]
              frame #0 {
                w1441 = T9 6.5 items=["3 1/2"=3.5, "4 1/2"=4.5, "5 1/2"=5.5, "6 1/2"=6.5, "7 1/2"=7.5] ("Resolution in Digits")
                n920 = Fract/Exp String To Number(string="NI DMM 2 Resistance Range") -> (number=w1435:dbl)  [unwired: 3 in, 1 out]
                n921 = call-poly <instrlib>:"niDMM Config Measurement.vi"("Range"=w1435, "Resolution in Digits"=w1441, "error in (no error)"=w1437, "Function"=niDMM_Function."2-wire Resistance" ("Measurement Type"), "instrument handle"=w1438) -> ("error out"=w1436:errorcluster, "instrument handle out"=w1439:refnum<k15>)  [unwired: 5 in]
              }
              frame #1 {
                n922 = call <instrlib>:"niDMM Read.vi"("error in (no error)"=w1448, "instrument handle"=w1444) -> ("error out"=w1447:errorcluster, "Measurement"=w1442:dbl, "instrument handle out"=w1443:refnum<k15>)  [unwired: 7 in]
                n923 = Fract/Exp String To Number(string="NI DMM 2 Resistance units") -> (number=w1445:dbl)  [unwired: 3 in, 1 out]
                n924 = Multiply(x=w1445, y=w1442) -> (x*y=→"NI DMM 2 Resistance" →"NI DMM 2 Resistance Char":dbl)
              }
              frame #2 {
                w1456 = 15
                n925 = local read "NI DMM 2 Resistance output file"() -> (w1462:refnum<file>)
                n926 = Format Date/Time String(time format string (%c)="%H:%M:%S:%3u") -> (date/time string=w1458:string)  [unwired: 2 in]
                n927 = Number To Fractional String(number=w1451, width (-)=w1456, precision (6)=w1456) -> (F-format string=w1450:string)  [unwired: 1 in]
                n928 = Concatenate Strings(w1458, "\t", w1450, "\r\n") -> (w1460:string)
                n929 = Format Into String(initial string=w1462, w1460) -> (resulting string=w1455:refnum<file>)  [unwired: 2 in, 1 out]
                n930 = local read "System Stop"() -> (w1453:bool)
              }
            }
            n931 = Wait (ms)(milliseconds to wait="NI DMM 2 Resistance Wait") -> ()  [unwired: 1 out]
            n932 = call <vilib>:"Simple Error Handler.vi"("error in (no error)"=w1424) -> ("error out"=w1423:errorcluster)  [unwired: 1 in, 7 out]
          }
        }
      }
      n933 = call <instrlib>:"niDMM Close.vi"("error in (no error)"=w1364, "instrument handle"=w1366) -> ("error out"=w1363:errorcluster)  [unwired: 9 in]
      n934 = local write "NI DMM 2 error out"(w1363) -> ()
      n935 = Close File(refnum=w1367) -> ()  [unwired: 1 in, 2 out]
      n936 = call <vilib>:"Simple Error Handler.vi"("error in (no error)"=w1363) -> ()  [unwired: 1 in, 8 out]
    }
  }
  n937 = case shown="True" w30 {
    tunnel: w35 -> [_ w1469]
    tunnel: w36 -> [_ w1466]
    tunnel: w2 -> [_ _]
    frame False {
    }
    frame True {
      n938 = local read "NI DMM 3 Option Return"() -> (w1463:enum32{"Ampermeter button", "Ohmmeter button"})
      n939 = case shown="\"Ampermeter button\", Default" w1463 {
        tunnel: w1469 -> [w1474 w1521]
        tunnel: [w1473 w1519] -> w1468
        tunnel: [w1472 w1518] -> w1467
        tunnel: w1466 -> [w1471 w1520]
        tunnel: [w1470 w1517] -> w1465
        frame "Ampermeter button", Default {
          n940 = while {
            tunnel: w1474 -> [w1486]
            tunnel: [w1484] -> w1473
            tunnel: [w1483] -> w1472
            tunnel: w1471 -> [w1481]
            tunnel: [w1477] -> w1470
            stop <- w1482 stop-if-true
            n941 = flat-sequence {
              tunnel: [w1490] -> w1487
              tunnel: w1486 -> [w1488]
              tunnel: w1481 -> [w1494]
              tunnel: [w1489] -> w1480
              tunnel: w1487 -> [w1496]
              tunnel: [w1502] -> w1485
              tunnel: w1480 -> [w1501]
              tunnel: [w1500] -> w1479
              tunnel: [w1497] -> w1475
              tunnel: w1485 -> [w1508]
              tunnel: [w1509] -> w1484
              tunnel: [w1508] -> w1483
              tunnel: [w1507] -> w1482
              tunnel: [w1506] -> w1478
              tunnel: w1479 -> [w1506]
              tunnel: w1475 -> [w1504]
              frame #0 {
                w1491 = T9 6.5 items=["3 1/2"=3.5, "4 1/2"=4.5, "5 1/2"=5.5, "6 1/2"=6.5, "7 1/2"=7.5] ("Resolution in Digits")
                n942 = Fract/Exp String To Number(string="NI DMM 3 Current Range") -> (number=w1493:dbl)  [unwired: 3 in, 1 out]
                n943 = call-poly <instrlib>:"niDMM Config Measurement.vi"("Range"=w1493, "Resolution in Digits"=w1491, "error in (no error)"=w1494, "Function"=niDMM_Function."DC Current" ("Measurement Type"), "instrument handle"=w1488) -> ("error out"=w1489:errorcluster, "instrument handle out"=w1490:refnum<k15>)  [unwired: 5 in]
              }
              frame #1 {
                n944 = call <instrlib>:"niDMM Read.vi"("error in (no error)"=w1501, "instrument handle"=w1496) -> ("error out"=w1500:errorcluster, "Measurement"=w1497:dbl, "instrument handle out"=w1502:refnum<k15>)  [unwired: 7 in]
                "DMM 3 Real Current" <- w1497
                n945 = Fract/Exp String To Number(string="NI DMM 3 units") -> (number=w1498:dbl)  [unwired: 3 in, 1 out]
                n946 = Multiply(x=w1498, y=w1497) -> (x*y=→"NI DMM 3 Current" →"NI DMM 3 Current Char":dbl)
              }
              frame #2 {
                w1510 = 15
                n947 = local read "NI DMM 3 Current output file"() -> (w1516:refnum<file>)
                n948 = Format Date/Time String(time format string (%c)="%H:%M:%S:%3u") -> (date/time string=w1512:string)  [unwired: 2 in]
                n949 = Number To Fractional String(number=w1504, width (-)=w1510, precision (6)=w1510) -> (F-format string=w1505:string)  [unwired: 1 in]
                n950 = Concatenate Strings(w1512, "\t", w1505, "\r\n") -> (w1514:string)
                n951 = Format Into String(initial string=w1516, w1514) -> (resulting string=w1509:refnum<file>)  [unwired: 2 in, 1 out]
                n952 = local read "System Stop"() -> (w1507:bool)
              }
            }
            n953 = Wait (ms)(milliseconds to wait="NI DMM 3 Current Wait") -> ()  [unwired: 1 out]
            n954 = call <vilib>:"Simple Error Handler.vi"("error in (no error)"=w1478) -> ("error out"=w1477:errorcluster)  [unwired: 1 in, 7 out]
          }
        }
        frame "Ohmmeter button" {
          n955 = while {
            tunnel: w1521 -> [w1533]
            tunnel: [w1531] -> w1519
            tunnel: [w1530] -> w1518
            tunnel: w1520 -> [w1528]
            tunnel: [w1524] -> w1517
            stop <- w1529 stop-if-true
            n956 = flat-sequence {
              tunnel: [w1540] -> w1534
              tunnel: w1533 -> [w1539]
              tunnel: w1528 -> [w1538]
              tunnel: [w1537] -> w1527
              tunnel: w1534 -> [w1545]
              tunnel: [w1544] -> w1532
              tunnel: w1527 -> [w1549]
              tunnel: [w1548] -> w1526
              tunnel: [w1543] -> w1522
              tunnel: w1532 -> [w1554]
              tunnel: [w1555] -> w1531
              tunnel: [w1554] -> w1530
              tunnel: [w1553] -> w1529
              tunnel: [w1552] -> w1525
              tunnel: w1526 -> [w1552]
              tunnel: w1522 -> [w1551]
              frame #0 {
                w1542 = T9 6.5 items=["3 1/2"=3.5, "4 1/2"=4.5, "5 1/2"=5.5, "6 1/2"=6.5, "7 1/2"=7.5] ("Resolution in Digits")
                n957 = Fract/Exp String To Number(string="NI DMM 3 Resistance Range") -> (number=w1536:dbl)  [unwired: 3 in, 1 out]
                n958 = call-poly <instrlib>:"niDMM Config Measurement.vi"("Range"=w1536, "Resolution in Digits"=w1542, "error in (no error)"=w1538, "Function"=niDMM_Function."2-wire Resistance" ("Measurement Type"), "instrument handle"=w1539) -> ("error out"=w1537:errorcluster, "instrument handle out"=w1540:refnum<k15>)  [unwired: 5 in]
              }
              frame #1 {
                n959 = call <instrlib>:"niDMM Read.vi"("error in (no error)"=w1549, "instrument handle"=w1545) -> ("error out"=w1548:errorcluster, "Measurement"=w1543:dbl, "instrument handle out"=w1544:refnum<k15>)  [unwired: 7 in]
                n960 = Fract/Exp String To Number(string="NI DMM 3 Resistance units") -> (number=w1546:dbl)  [unwired: 3 in, 1 out]
                n961 = Multiply(x=w1546, y=w1543) -> (x*y=→"NI DMM 3 Resistance" →"NI DMM 3 Resistance Char":dbl)
              }
              frame #2 {
                w1556 = 15
                n962 = local read "NI DMM 3 Resistance output file"() -> (w1563:refnum<file>)
                n963 = Format Date/Time String(time format string (%c)="%H:%M:%S:%3u") -> (date/time string=w1558:string)  [unwired: 2 in]
                n964 = Number To Fractional String(number=w1551, width (-)=w1556, precision (6)=w1556) -> (F-format string=w1561:string)  [unwired: 1 in]
                n965 = local read "System Stop"() -> (w1553:bool)
                n966 = Concatenate Strings(w1558, "\t", w1561, "\r\n") -> (w1560:string)
                n967 = Format Into String(initial string=w1563, w1560) -> (resulting string=w1555:refnum<file>)  [unwired: 2 in, 1 out]
              }
            }
            n968 = Wait (ms)(milliseconds to wait="NI DMM 3 Resistance Wait") -> ()  [unwired: 1 out]
            n969 = call <vilib>:"Simple Error Handler.vi"("error in (no error)"=w1525) -> ("error out"=w1524:errorcluster)  [unwired: 1 in, 7 out]
          }
        }
      }
      n970 = call <instrlib>:"niDMM Close.vi"("error in (no error)"=w1465, "instrument handle"=w1467) -> ("error out"=w1464:errorcluster)  [unwired: 9 in]
      n971 = local write "NI DMM 3 error out"(w1464) -> ()
      n972 = Close File(refnum=w1468) -> ()  [unwired: 1 in, 2 out]
      n973 = call <vilib>:"Simple Error Handler.vi"("error in (no error)"=w1464) -> ()  [unwired: 1 in, 8 out]
    }
  }
  n974 = case shown="True" w3 {
    tunnel: w2 -> [_ _]
    frame False {
    }
    frame True {
      n975 = while {
        stop <- w1565 stop-if-true
        n976 = local read "System Stop"() -> (w1572:bool)
        n977 = Wait (ms)(milliseconds to wait=u32 100) -> ()  [unwired: 1 out]
        n978 = Or(x="P1 CH0 Used", y=w1572) -> (x .or. y?=w1574:bool)
        n979 = case shown="True" w1574 {
          frame False {
            w1579 = T7."Disabled and Grayed Out" ("Disabled")
            n980 = property on="P1 CH0" class="Bool (strict)"("DisabledEnum"=w1579) -> ()  [unwired: 2 in, 2 out]
            n981 = property on="P1 CH0_char" class="WFChart (strict)"("DisabledEnum"=w1579) -> ()  [unwired: 2 in, 2 out]
            n982 = property on="P1 CH0, V" class="DigNum (strict)"("DisabledEnum"=w1579) -> ()  [unwired: 2 in, 2 out]
            n983 = property on="P1 CH0_curlim, A" class="DigNum (strict)"("DisabledEnum"=w1579) -> ()  [unwired: 2 in, 2 out]
            n984 = property on="P1 CH0_cur, A" class="DigNum (strict)"("DisabledEnum"=w1579) -> ()  [unwired: 2 in, 2 out]
            n985 = property on="P1 CH0_selcur, A" class="DigNum (strict)"("DisabledEnum"=w1579) -> ()  [unwired: 2 in, 2 out]
            n986 = property on="P1 CH0_counter" class="DigNum (strict)"("DisabledEnum"=w1579) -> ()  [unwired: 2 in, 2 out]
            n987 = property on="P1 CH0_warning" class="Bool (strict)"("DisabledEnum"=w1579) -> ()  [unwired: 2 in, 2 out]
          }
          frame True {
            w1580 = T7."Enabled" ("Disabled")
            n988 = property on="P1 CH0" class="Bool (strict)"("DisabledEnum"=w1580) -> ()  [unwired: 2 in, 2 out]
            n989 = property on="P1 CH0_char" class="WFChart (strict)"("DisabledEnum"=w1580) -> ()  [unwired: 2 in, 2 out]
            n990 = property on="P1 CH0, V" class="DigNum (strict)"("DisabledEnum"=w1580) -> ()  [unwired: 2 in, 2 out]
            n991 = property on="P1 CH0_curlim, A" class="DigNum (strict)"("DisabledEnum"=w1580) -> ()  [unwired: 2 in, 2 out]
            n992 = property on="P1 CH0_cur, A" class="DigNum (strict)"("DisabledEnum"=w1580) -> ()  [unwired: 2 in, 2 out]
            n993 = property on="P1 CH0_selcur, A" class="DigNum (strict)"("DisabledEnum"=w1580) -> ()  [unwired: 2 in, 2 out]
            n994 = property on="P1 CH0_counter" class="DigNum (strict)"("DisabledEnum"=w1580) -> ()  [unwired: 2 in, 2 out]
            n995 = property on="P1 CH0_warning" class="Bool (strict)"("DisabledEnum"=w1580) -> ()  [unwired: 2 in, 2 out]
          }
        }
        n996 = local read "System Stop"() -> (w1569:bool)
        n997 = Or(x="P1 CH1 Used", y=w1569) -> (x .or. y?=w1571:bool)
        n998 = case shown="True" w1571 {
          frame False {
            w1577 = T7."Disabled and Grayed Out" ("Disabled")
            n999 = property on="P1 CH1" class="Bool (strict)"("DisabledEnum"=w1577) -> ()  [unwired: 2 in, 2 out]
            n1000 = property on="P1 CH1_char" class="WFChart (strict)"("DisabledEnum"=w1577) -> ()  [unwired: 2 in, 2 out]
            n1001 = property on="P1 CH1, V" class="DigNum (strict)"("DisabledEnum"=w1577) -> ()  [unwired: 2 in, 2 out]
            n1002 = property on="P1 CH1_curlim, A" class="DigNum (strict)"("DisabledEnum"=w1577) -> ()  [unwired: 2 in, 2 out]
            n1003 = property on="P1 CH1_cur, A" class="DigNum (strict)"("DisabledEnum"=w1577) -> ()  [unwired: 2 in, 2 out]
            n1004 = property on="P1 CH1_selcur, A" class="DigNum (strict)"("DisabledEnum"=w1577) -> ()  [unwired: 2 in, 2 out]
            n1005 = property on="P1 CH1_counter" class="DigNum (strict)"("DisabledEnum"=w1577) -> ()  [unwired: 2 in, 2 out]
            n1006 = property on="P1 CH1_warning" class="Bool (strict)"("DisabledEnum"=w1577) -> ()  [unwired: 2 in, 2 out]
          }
          frame True {
            w1578 = T7."Enabled" ("Disabled")
            n1007 = property on="P1 CH1" class="Bool (strict)"("DisabledEnum"=w1578) -> ()  [unwired: 2 in, 2 out]
            n1008 = property on="P1 CH1_char" class="WFChart (strict)"("DisabledEnum"=w1578) -> ()  [unwired: 2 in, 2 out]
            n1009 = property on="P1 CH1, V" class="DigNum (strict)"("DisabledEnum"=w1578) -> ()  [unwired: 2 in, 2 out]
            n1010 = property on="P1 CH1_curlim, A" class="DigNum (strict)"("DisabledEnum"=w1578) -> ()  [unwired: 2 in, 2 out]
            n1011 = property on="P1 CH1_cur, A" class="DigNum (strict)"("DisabledEnum"=w1578) -> ()  [unwired: 2 in, 2 out]
            n1012 = property on="P1 CH1_selcur, A" class="DigNum (strict)"("DisabledEnum"=w1578) -> ()  [unwired: 2 in, 2 out]
            n1013 = property on="P1 CH1_counter" class="DigNum (strict)"("DisabledEnum"=w1578) -> ()  [unwired: 2 in, 2 out]
            n1014 = property on="P1 CH1_warning" class="Bool (strict)"("DisabledEnum"=w1578) -> ()  [unwired: 2 in, 2 out]
          }
        }
        n1015 = local read "System Stop"() -> (w1568:bool)
        n1016 = Or(x="P1 CH2 Used", y=w1568) -> (x .or. y?=w1566:bool)
        n1017 = case shown="True" w1566 {
          frame False {
            w1575 = T7."Disabled and Grayed Out" ("Disabled")
            n1018 = property on="P1 CH2" class="Bool (strict)"("DisabledEnum"=w1575) -> ()  [unwired: 2 in, 2 out]
            n1019 = property on="P1 CH2_char" class="WFChart (strict)"("DisabledEnum"=w1575) -> ()  [unwired: 2 in, 2 out]
            n1020 = property on="P1 CH2, V" class="DigNum (strict)"("DisabledEnum"=w1575) -> ()  [unwired: 2 in, 2 out]
            n1021 = property on="P1 CH2_curlim, A" class="DigNum (strict)"("DisabledEnum"=w1575) -> ()  [unwired: 2 in, 2 out]
            n1022 = property on="P1 CH2_cur, A" class="DigNum (strict)"("DisabledEnum"=w1575) -> ()  [unwired: 2 in, 2 out]
            n1023 = property on="P1 CH2_selcur, A" class="DigNum (strict)"("DisabledEnum"=w1575) -> ()  [unwired: 2 in, 2 out]
            n1024 = property on="P1 CH2_counter" class="DigNum (strict)"("DisabledEnum"=w1575) -> ()  [unwired: 2 in, 2 out]
            n1025 = property on="P1 CH2_warning" class="Bool (strict)"("DisabledEnum"=w1575) -> ()  [unwired: 2 in, 2 out]
          }
          frame True {
            w1576 = T7."Enabled" ("Disabled")
            n1026 = property on="P1 CH2_char" class="WFChart (strict)"("DisabledEnum"=w1576) -> ()  [unwired: 2 in, 2 out]
            n1027 = property on="P1 CH2, V" class="DigNum (strict)"("DisabledEnum"=w1576) -> ()  [unwired: 2 in, 2 out]
            n1028 = property on="P1 CH2_curlim, A" class="DigNum (strict)"("DisabledEnum"=w1576) -> ()  [unwired: 2 in, 2 out]
            n1029 = property on="P1 CH2_cur, A" class="DigNum (strict)"("DisabledEnum"=w1576) -> ()  [unwired: 2 in, 2 out]
            n1030 = property on="P1 CH2_selcur, A" class="DigNum (strict)"("DisabledEnum"=w1576) -> ()  [unwired: 2 in, 2 out]
            n1031 = property on="P1 CH2_counter" class="DigNum (strict)"("DisabledEnum"=w1576) -> ()  [unwired: 2 in, 2 out]
            n1032 = property on="P1 CH2_warning" class="Bool (strict)"("DisabledEnum"=w1576) -> ()  [unwired: 2 in, 2 out]
            n1033 = property on="P1 CH2" class="Bool (strict)"("DisabledEnum"=w1576) -> ()  [unwired: 2 in, 2 out]
          }
        }
        n1034 = local read "System Stop"() -> (w1565:bool)
      }
    }
  }
  n1035 = case shown="True" w4 {
    tunnel: w2 -> [_ _]
    frame False {
    }
    frame True {
      n1036 = while {
        stop <- w1582 stop-if-true
        n1037 = local read "System Stop"() -> (w1588:bool)
        n1038 = Wait (ms)(milliseconds to wait=u32 100) -> ()  [unwired: 1 out]
        n1039 = Or(x="P2 CH0 Used", y=w1588) -> (x .or. y?=w1586:bool)
        n1040 = case shown="True" w1586 {
          frame False {
            w1594 = T7."Disabled and Grayed Out" ("Disabled")
            n1041 = property on="P2 CH0" class="Bool (strict)"("DisabledEnum"=w1594) -> ()  [unwired: 2 in, 2 out]
            n1042 = property on="P2 CH0_char" class="WFChart (strict)"("DisabledEnum"=w1594) -> ()  [unwired: 2 in, 2 out]
            n1043 = property on="P2 CH0, V" class="DigNum (strict)"("DisabledEnum"=w1594) -> ()  [unwired: 2 in, 2 out]
            n1044 = property on="P2 CH0_curlim, A" class="DigNum (strict)"("DisabledEnum"=w1594) -> ()  [unwired: 2 in, 2 out]
            n1045 = property on="P2 CH0_cur, A" class="DigNum (strict)"("DisabledEnum"=w1594) -> ()  [unwired: 2 in, 2 out]
            n1046 = property on="P2 CH0_selcur, A" class="DigNum (strict)"("DisabledEnum"=w1594) -> ()  [unwired: 2 in, 2 out]
            n1047 = property on="P2 CH0_counter" class="DigNum (strict)"("DisabledEnum"=w1594) -> ()  [unwired: 2 in, 2 out]
            n1048 = property on="P2 CH0_warning" class="Bool (strict)"("DisabledEnum"=w1594) -> ()  [unwired: 2 in, 2 out]
          }
          frame True {
            w1595 = T7."Enabled" ("Disabled")
            n1049 = property on="P2 CH0" class="Bool (strict)"("DisabledEnum"=w1595) -> ()  [unwired: 2 in, 2 out]
            n1050 = property on="P2 CH0_char" class="WFChart (strict)"("DisabledEnum"=w1595) -> ()  [unwired: 2 in, 2 out]
            n1051 = property on="P2 CH0, V" class="DigNum (strict)"("DisabledEnum"=w1595) -> ()  [unwired: 2 in, 2 out]
            n1052 = property on="P2 CH0_curlim, A" class="DigNum (strict)"("DisabledEnum"=w1595) -> ()  [unwired: 2 in, 2 out]
            n1053 = property on="P2 CH0_cur, A" class="DigNum (strict)"("DisabledEnum"=w1595) -> ()  [unwired: 2 in, 2 out]
            n1054 = property on="P2 CH0_selcur, A" class="DigNum (strict)"("DisabledEnum"=w1595) -> ()  [unwired: 2 in, 2 out]
            n1055 = property on="P2 CH0_counter" class="DigNum (strict)"("DisabledEnum"=w1595) -> ()  [unwired: 2 in, 2 out]
            n1056 = property on="P2 CH0_warning" class="Bool (strict)"("DisabledEnum"=w1595) -> ()  [unwired: 2 in, 2 out]
          }
        }
        n1057 = local read "System Stop"() -> (w1585:bool)
        n1058 = Or(x="P2 CH1 Used", y=w1585) -> (x .or. y?=w1584:bool)
        n1059 = case shown="True" w1584 {
          frame False {
            w1596 = T7."Disabled and Grayed Out" ("Disabled")
            n1060 = property on="P2 CH1" class="Bool (strict)"("DisabledEnum"=w1596) -> ()  [unwired: 2 in, 2 out]
            n1061 = property on="P2 CH1_char" class="WFChart (strict)"("DisabledEnum"=w1596) -> ()  [unwired: 2 in, 2 out]
            n1062 = property on="P2 CH1, V" class="DigNum (strict)"("DisabledEnum"=w1596) -> ()  [unwired: 2 in, 2 out]
            n1063 = property on="P2 CH1_curlim, A" class="DigNum (strict)"("DisabledEnum"=w1596) -> ()  [unwired: 2 in, 2 out]
            n1064 = property on="P2 CH1_cur, A" class="DigNum (strict)"("DisabledEnum"=w1596) -> ()  [unwired: 2 in, 2 out]
            n1065 = property on="P2 CH1_selcur, A" class="DigNum (strict)"("DisabledEnum"=w1596) -> ()  [unwired: 2 in, 2 out]
            n1066 = property on="P2 CH1_counter" class="DigNum (strict)"("DisabledEnum"=w1596) -> ()  [unwired: 2 in, 2 out]
            n1067 = property on="P2 CH1_warning" class="Bool (strict)"("DisabledEnum"=w1596) -> ()  [unwired: 2 in, 2 out]
          }
          frame True {
            w1597 = T7."Enabled" ("Disabled")
            n1068 = property on="P2 CH1" class="Bool (strict)"("DisabledEnum"=w1597) -> ()  [unwired: 2 in, 2 out]
            n1069 = property on="P2 CH1_char" class="WFChart (strict)"("DisabledEnum"=w1597) -> ()  [unwired: 2 in, 2 out]
            n1070 = property on="P2 CH1, V" class="DigNum (strict)"("DisabledEnum"=w1597) -> ()  [unwired: 2 in, 2 out]
            n1071 = property on="P2 CH1_curlim, A" class="DigNum (strict)"("DisabledEnum"=w1597) -> ()  [unwired: 2 in, 2 out]
            n1072 = property on="P2 CH1_cur, A" class="DigNum (strict)"("DisabledEnum"=w1597) -> ()  [unwired: 2 in, 2 out]
            n1073 = property on="P2 CH1_selcur, A" class="DigNum (strict)"("DisabledEnum"=w1597) -> ()  [unwired: 2 in, 2 out]
            n1074 = property on="P2 CH1_counter" class="DigNum (strict)"("DisabledEnum"=w1597) -> ()  [unwired: 2 in, 2 out]
            n1075 = property on="P2 CH1_warning" class="Bool (strict)"("DisabledEnum"=w1597) -> ()  [unwired: 2 in, 2 out]
          }
        }
        n1076 = local read "System Stop"() -> (w1589:bool)
        n1077 = Or(x="P2 CH2 Used", y=w1589) -> (x .or. y?=w1590:bool)
        n1078 = case shown="True" w1590 {
          frame False {
            w1592 = T7."Disabled and Grayed Out" ("Disabled")
            n1079 = property on="P2 CH2" class="Bool (strict)"("DisabledEnum"=w1592) -> ()  [unwired: 2 in, 2 out]
            n1080 = property on="P2 CH2_char" class="WFChart (strict)"("DisabledEnum"=w1592) -> ()  [unwired: 2 in, 2 out]
            n1081 = property on="P2 CH2, V" class="DigNum (strict)"("DisabledEnum"=w1592) -> ()  [unwired: 2 in, 2 out]
            n1082 = property on="P2 CH2_curlim, A" class="DigNum (strict)"("DisabledEnum"=w1592) -> ()  [unwired: 2 in, 2 out]
            n1083 = property on="P2 CH2_cur, A" class="DigNum (strict)"("DisabledEnum"=w1592) -> ()  [unwired: 2 in, 2 out]
            n1084 = property on="P2 CH2_selcur, A" class="DigNum (strict)"("DisabledEnum"=w1592) -> ()  [unwired: 2 in, 2 out]
            n1085 = property on="P2 CH2_counter" class="DigNum (strict)"("DisabledEnum"=w1592) -> ()  [unwired: 2 in, 2 out]
            n1086 = property on="P2 CH2_warning" class="Bool (strict)"("DisabledEnum"=w1592) -> ()  [unwired: 2 in, 2 out]
          }
          frame True {
            w1593 = T7."Enabled" ("Disabled")
            n1087 = property on="P2 CH2" class="Bool (strict)"("DisabledEnum"=w1593) -> ()  [unwired: 2 in, 2 out]
            n1088 = property on="P2 CH2_char" class="WFChart (strict)"("DisabledEnum"=w1593) -> ()  [unwired: 2 in, 2 out]
            n1089 = property on="P2 CH2, V" class="DigNum (strict)"("DisabledEnum"=w1593) -> ()  [unwired: 2 in, 2 out]
            n1090 = property on="P2 CH2_curlim, A" class="DigNum (strict)"("DisabledEnum"=w1593) -> ()  [unwired: 2 in, 2 out]
            n1091 = property on="P2 CH2_cur, A" class="DigNum (strict)"("DisabledEnum"=w1593) -> ()  [unwired: 2 in, 2 out]
            n1092 = property on="P2 CH2_selcur, A" class="DigNum (strict)"("DisabledEnum"=w1593) -> ()  [unwired: 2 in, 2 out]
            n1093 = property on="P2 CH2_counter" class="DigNum (strict)"("DisabledEnum"=w1593) -> ()  [unwired: 2 in, 2 out]
            n1094 = property on="P2 CH2_warning" class="Bool (strict)"("DisabledEnum"=w1593) -> ()  [unwired: 2 in, 2 out]
          }
        }
        n1095 = local read "System Stop"() -> (w1582:bool)
      }
    }
  }
  n1096 = case shown="True" w6 {
    tunnel: w2 -> [_ _]
    frame False {
    }
    frame True {
      n1097 = while {
        stop <- w1608 stop-if-true
        n1098 = local read "System Stop"() -> (w1602:bool)
        n1099 = Wait (ms)(milliseconds to wait=u32 100) -> ()  [unwired: 1 out]
        n1100 = Or(x="P4 CH0 Used", y=w1602) -> (x .or. y?=w1604:bool)
        n1101 = case shown="True" w1604 {
          frame False {
            w1611 = T7."Disabled and Grayed Out" ("Disabled")
            n1102 = property on="P4 CH0" class="Bool (strict)"("DisabledEnum"=w1611) -> ()  [unwired: 2 in, 2 out]
            n1103 = property on="P4 CH0_char" class="WFChart (strict)"("DisabledEnum"=w1611) -> ()  [unwired: 2 in, 2 out]
            n1104 = property on="P4 CH0, V" class="DigNum (strict)"("DisabledEnum"=w1611) -> ()  [unwired: 2 in, 2 out]
            n1105 = property on="P4 CH0_curlim, A" class="DigNum (strict)"("DisabledEnum"=w1611) -> ()  [unwired: 2 in, 2 out]
            n1106 = property on="P4 CH0_cur, A" class="DigNum (strict)"("DisabledEnum"=w1611) -> ()  [unwired: 2 in, 2 out]
            n1107 = property on="P4 CH0_selcur, A" class="DigNum (strict)"("DisabledEnum"=w1611) -> ()  [unwired: 2 in, 2 out]
            n1108 = property on="P4 CH0_counter" class="DigNum (strict)"("DisabledEnum"=w1611) -> ()  [unwired: 2 in, 2 out]
            n1109 = property on="P4 CH0_warning" class="Bool (strict)"("DisabledEnum"=w1611) -> ()  [unwired: 2 in, 2 out]
          }
          frame True {
            w1612 = T7."Enabled" ("Disabled")
            n1110 = property on="P4 CH0" class="Bool (strict)"("DisabledEnum"=w1612) -> ()  [unwired: 2 in, 2 out]
            n1111 = property on="P4 CH0_char" class="WFChart (strict)"("DisabledEnum"=w1612) -> ()  [unwired: 2 in, 2 out]
            n1112 = property on="P4 CH0, V" class="DigNum (strict)"("DisabledEnum"=w1612) -> ()  [unwired: 2 in, 2 out]
            n1113 = property on="P4 CH0_curlim, A" class="DigNum (strict)"("DisabledEnum"=w1612) -> ()  [unwired: 2 in, 2 out]
            n1114 = property on="P4 CH0_cur, A" class="DigNum (strict)"("DisabledEnum"=w1612) -> ()  [unwired: 2 in, 2 out]
            n1115 = property on="P4 CH0_selcur, A" class="DigNum (strict)"("DisabledEnum"=w1612) -> ()  [unwired: 2 in, 2 out]
            n1116 = property on="P4 CH0_counter" class="DigNum (strict)"("DisabledEnum"=w1612) -> ()  [unwired: 2 in, 2 out]
            n1117 = property on="P4 CH0_warning" class="Bool (strict)"("DisabledEnum"=w1612) -> ()  [unwired: 2 in, 2 out]
          }
        }
        n1118 = local read "System Stop"() -> (w1605:bool)
        n1119 = Or(x="P4 CH1 Used", y=w1605) -> (x .or. y?=w1606:bool)
        n1120 = case shown="True" w1606 {
          frame False {
            w1613 = T7."Disabled and Grayed Out" ("Disabled")
            n1121 = property on="P4 CH1" class="Bool (strict)"("DisabledEnum"=w1613) -> ()  [unwired: 2 in, 2 out]
            n1122 = property on="P4 CH1_char" class="WFChart (strict)"("DisabledEnum"=w1613) -> ()  [unwired: 2 in, 2 out]
            n1123 = property on="P4 CH1, V" class="DigNum (strict)"("DisabledEnum"=w1613) -> ()  [unwired: 2 in, 2 out]
            n1124 = property on="P4 CH1_curlim, A" class="DigNum (strict)"("DisabledEnum"=w1613) -> ()  [unwired: 2 in, 2 out]
            n1125 = property on="P4 CH1_cur, A" class="DigNum (strict)"("DisabledEnum"=w1613) -> ()  [unwired: 2 in, 2 out]
            n1126 = property on="P4 CH1_selcur, A" class="DigNum (strict)"("DisabledEnum"=w1613) -> ()  [unwired: 2 in, 2 out]
            n1127 = property on="P4 CH1_counter" class="DigNum (strict)"("DisabledEnum"=w1613) -> ()  [unwired: 2 in, 2 out]
            n1128 = property on="P4 CH1_warning" class="Bool (strict)"("DisabledEnum"=w1613) -> ()  [unwired: 2 in, 2 out]
          }
          frame True {
            w1614 = T7."Enabled" ("Disabled")
            n1129 = property on="P4 CH1" class="Bool (strict)"("DisabledEnum"=w1614) -> ()  [unwired: 2 in, 2 out]
            n1130 = property on="P4 CH1_char" class="WFChart (strict)"("DisabledEnum"=w1614) -> ()  [unwired: 2 in, 2 out]
            n1131 = property on="P4 CH1, V" class="DigNum (strict)"("DisabledEnum"=w1614) -> ()  [unwired: 2 in, 2 out]
            n1132 = property on="P4 CH1_curlim, A" class="DigNum (strict)"("DisabledEnum"=w1614) -> ()  [unwired: 2 in, 2 out]
            n1133 = property on="P4 CH1_cur, A" class="DigNum (strict)"("DisabledEnum"=w1614) -> ()  [unwired: 2 in, 2 out]
            n1134 = property on="P4 CH1_selcur, A" class="DigNum (strict)"("DisabledEnum"=w1614) -> ()  [unwired: 2 in, 2 out]
            n1135 = property on="P4 CH1_counter" class="DigNum (strict)"("DisabledEnum"=w1614) -> ()  [unwired: 2 in, 2 out]
            n1136 = property on="P4 CH1_warning" class="Bool (strict)"("DisabledEnum"=w1614) -> ()  [unwired: 2 in, 2 out]
          }
        }
        n1137 = local read "System Stop"() -> (w1601:bool)
        n1138 = Or(x="P4 CH2 Used", y=w1601) -> (x .or. y?=w1600:bool)
        n1139 = case shown="True" w1600 {
          frame False {
            w1609 = T7."Disabled and Grayed Out" ("Disabled")
            n1140 = property on="P4 CH2" class="Bool (strict)"("DisabledEnum"=w1609) -> ()  [unwired: 2 in, 2 out]
            n1141 = property on="P4 CH2_char" class="WFChart (strict)"("DisabledEnum"=w1609) -> ()  [unwired: 2 in, 2 out]
            n1142 = property on="P4 CH2, V" class="DigNum (strict)"("DisabledEnum"=w1609) -> ()  [unwired: 2 in, 2 out]
            n1143 = property on="P4 CH2_curlim, A" class="DigNum (strict)"("DisabledEnum"=w1609) -> ()  [unwired: 2 in, 2 out]
            n1144 = property on="P4 CH2_cur, A" class="DigNum (strict)"("DisabledEnum"=w1609) -> ()  [unwired: 2 in, 2 out]
            n1145 = property on="P4 CH2_selcur, A" class="DigNum (strict)"("DisabledEnum"=w1609) -> ()  [unwired: 2 in, 2 out]
            n1146 = property on="P4 CH2_counter" class="DigNum (strict)"("DisabledEnum"=w1609) -> ()  [unwired: 2 in, 2 out]
            n1147 = property on="P4 CH2_warning" class="Bool (strict)"("DisabledEnum"=w1609) -> ()  [unwired: 2 in, 2 out]
          }
          frame True {
            w1610 = T7."Enabled" ("Disabled")
            n1148 = property on="P4 CH2" class="Bool (strict)"("DisabledEnum"=w1610) -> ()  [unwired: 2 in, 2 out]
            n1149 = property on="P4 CH2_char" class="WFChart (strict)"("DisabledEnum"=w1610) -> ()  [unwired: 2 in, 2 out]
            n1150 = property on="P4 CH2, V" class="DigNum (strict)"("DisabledEnum"=w1610) -> ()  [unwired: 2 in, 2 out]
            n1151 = property on="P4 CH2_curlim, A" class="DigNum (strict)"("DisabledEnum"=w1610) -> ()  [unwired: 2 in, 2 out]
            n1152 = property on="P4 CH2_cur, A" class="DigNum (strict)"("DisabledEnum"=w1610) -> ()  [unwired: 2 in, 2 out]
            n1153 = property on="P4 CH2_selcur, A" class="DigNum (strict)"("DisabledEnum"=w1610) -> ()  [unwired: 2 in, 2 out]
            n1154 = property on="P4 CH2_counter" class="DigNum (strict)"("DisabledEnum"=w1610) -> ()  [unwired: 2 in, 2 out]
            n1155 = property on="P4 CH2_warning" class="Bool (strict)"("DisabledEnum"=w1610) -> ()  [unwired: 2 in, 2 out]
          }
        }
        n1156 = local read "System Stop"() -> (w1608:bool)
      }
    }
  }
  n1157 = case shown="True" w5 {
    tunnel: w2 -> [_ _]
    frame False {
    }
    frame True {
      n1158 = while {
        stop <- w1625 stop-if-true
        n1159 = local read "System Stop"() -> (w1623:bool)
        n1160 = Wait (ms)(milliseconds to wait=u32 100) -> ()  [unwired: 1 out]
        n1161 = Or(x="P3 CH0 Used", y=w1623) -> (x .or. y?=w1624:bool)
        n1162 = case shown="False" w1624 {
          frame False {
            w1630 = T7."Disabled and Grayed Out" ("Disabled")
            n1163 = property on="P3 CH0" class="Bool (strict)"("DisabledEnum"=w1630) -> ()  [unwired: 2 in, 2 out]
            n1164 = property on="P3 CH0_char" class="WFChart (strict)"("DisabledEnum"=w1630) -> ()  [unwired: 2 in, 2 out]
            n1165 = property on="P3 CH0, V" class="DigNum (strict)"("DisabledEnum"=w1630) -> ()  [unwired: 2 in, 2 out]
            n1166 = property on="P3 CH0_curlim, A" class="DigNum (strict)"("DisabledEnum"=w1630) -> ()  [unwired: 2 in, 2 out]
            n1167 = property on="P3 CH0_cur, A" class="DigNum (strict)"("DisabledEnum"=w1630) -> ()  [unwired: 2 in, 2 out]
            n1168 = property on="P3 CH0_selcur, A" class="DigNum (strict)"("DisabledEnum"=w1630) -> ()  [unwired: 2 in, 2 out]
            n1169 = property on="P3 CH0_counter" class="DigNum (strict)"("DisabledEnum"=w1630) -> ()  [unwired: 2 in, 2 out]
            n1170 = property on="P3 CH0_warning" class="Bool (strict)"("DisabledEnum"=w1630) -> ()  [unwired: 2 in, 2 out]
          }
          frame True {
            w1631 = T7."Enabled" ("Disabled")
            n1171 = property on="P3 CH0" class="Bool (strict)"("DisabledEnum"=w1631) -> ()  [unwired: 2 in, 2 out]
            n1172 = property on="P3 CH0_char" class="WFChart (strict)"("DisabledEnum"=w1631) -> ()  [unwired: 2 in, 2 out]
            n1173 = property on="P3 CH0, V" class="DigNum (strict)"("DisabledEnum"=w1631) -> ()  [unwired: 2 in, 2 out]
            n1174 = property on="P3 CH0_curlim, A" class="DigNum (strict)"("DisabledEnum"=w1631) -> ()  [unwired: 2 in, 2 out]
            n1175 = property on="P3 CH0_cur, A" class="DigNum (strict)"("DisabledEnum"=w1631) -> ()  [unwired: 2 in, 2 out]
            n1176 = property on="P3 CH0_selcur, A" class="DigNum (strict)"("DisabledEnum"=w1631) -> ()  [unwired: 2 in, 2 out]
            n1177 = property on="P3 CH0_counter" class="DigNum (strict)"("DisabledEnum"=w1631) -> ()  [unwired: 2 in, 2 out]
            n1178 = property on="P3 CH0_warning" class="Bool (strict)"("DisabledEnum"=w1631) -> ()  [unwired: 2 in, 2 out]
          }
        }
        n1179 = local read "System Stop"() -> (w1620:bool)
        n1180 = Or(x="P3 CH1 Used", y=w1620) -> (x .or. y?=w1622:bool)
        n1181 = case shown="False" w1622 {
          frame False {
            w1628 = T7."Disabled and Grayed Out" ("Disabled")
            n1182 = property on="P3 CH1" class="Bool (strict)"("DisabledEnum"=w1628) -> ()  [unwired: 2 in, 2 out]
            n1183 = property on="P3 CH1_char" class="WFChart (strict)"("DisabledEnum"=w1628) -> ()  [unwired: 2 in, 2 out]
            n1184 = property on="P3 CH1, V" class="DigNum (strict)"("DisabledEnum"=w1628) -> ()  [unwired: 2 in, 2 out]
            n1185 = property on="P3 CH1_curlim, A" class="DigNum (strict)"("DisabledEnum"=w1628) -> ()  [unwired: 2 in, 2 out]
            n1186 = property on="P3 CH1_cur, A" class="DigNum (strict)"("DisabledEnum"=w1628) -> ()  [unwired: 2 in, 2 out]
            n1187 = property on="P3 CH1_selcur, A" class="DigNum (strict)"("DisabledEnum"=w1628) -> ()  [unwired: 2 in, 2 out]
            n1188 = property on="P3 CH1_counter" class="DigNum (strict)"("DisabledEnum"=w1628) -> ()  [unwired: 2 in, 2 out]
            n1189 = property on="P3 CH1_warning" class="Bool (strict)"("DisabledEnum"=w1628) -> ()  [unwired: 2 in, 2 out]
          }
          frame True {
            w1629 = T7."Enabled" ("Disabled")
            n1190 = property on="P3 CH1" class="Bool (strict)"("DisabledEnum"=w1629) -> ()  [unwired: 2 in, 2 out]
            n1191 = property on="P3 CH1_char" class="WFChart (strict)"("DisabledEnum"=w1629) -> ()  [unwired: 2 in, 2 out]
            n1192 = property on="P3 CH1, V" class="DigNum (strict)"("DisabledEnum"=w1629) -> ()  [unwired: 2 in, 2 out]
            n1193 = property on="P3 CH1_curlim, A" class="DigNum (strict)"("DisabledEnum"=w1629) -> ()  [unwired: 2 in, 2 out]
            n1194 = property on="P3 CH1_cur, A" class="DigNum (strict)"("DisabledEnum"=w1629) -> ()  [unwired: 2 in, 2 out]
            n1195 = property on="P3 CH1_selcur, A" class="DigNum (strict)"("DisabledEnum"=w1629) -> ()  [unwired: 2 in, 2 out]
            n1196 = property on="P3 CH1_counter" class="DigNum (strict)"("DisabledEnum"=w1629) -> ()  [unwired: 2 in, 2 out]
            n1197 = property on="P3 CH1_warning" class="Bool (strict)"("DisabledEnum"=w1629) -> ()  [unwired: 2 in, 2 out]
          }
        }
        n1198 = local read "System Stop"() -> (w1619:bool)
        n1199 = Or(x="P3 CH2 Used", y=w1619) -> (x .or. y?=w1617:bool)
        n1200 = case shown="False" w1617 {
          frame False {
            w1626 = T7."Disabled and Grayed Out" ("Disabled")
            n1201 = property on="P3 CH2_char" class="WFChart (strict)"("DisabledEnum"=w1626) -> ()  [unwired: 2 in, 2 out]
            n1202 = property on="P3 CH2, V" class="DigNum (strict)"("DisabledEnum"=w1626) -> ()  [unwired: 2 in, 2 out]
            n1203 = property on="P3 CH2_curlim, A" class="DigNum (strict)"("DisabledEnum"=w1626) -> ()  [unwired: 2 in, 2 out]
            n1204 = property on="P3 CH2_cur, A" class="DigNum (strict)"("DisabledEnum"=w1626) -> ()  [unwired: 2 in, 2 out]
            n1205 = property on="P3 CH2_selcur, A" class="DigNum (strict)"("DisabledEnum"=w1626) -> ()  [unwired: 2 in, 2 out]
            n1206 = property on="P3 CH2_counter" class="DigNum (strict)"("DisabledEnum"=w1626) -> ()  [unwired: 2 in, 2 out]
            n1207 = property on="P3 CH2_warning" class="Bool (strict)"("DisabledEnum"=w1626) -> ()  [unwired: 2 in, 2 out]
            n1208 = property on="P3 CH2" class="Bool (strict)"("DisabledEnum"=w1626) -> ()  [unwired: 2 in, 2 out]
          }
          frame True {
            w1627 = T7."Enabled" ("Disabled")
            n1209 = property on="P3 CH2_char" class="WFChart (strict)"("DisabledEnum"=w1627) -> ()  [unwired: 2 in, 2 out]
            n1210 = property on="P3 CH2, V" class="DigNum (strict)"("DisabledEnum"=w1627) -> ()  [unwired: 2 in, 2 out]
            n1211 = property on="P3 CH2_curlim, A" class="DigNum (strict)"("DisabledEnum"=w1627) -> ()  [unwired: 2 in, 2 out]
            n1212 = property on="P3 CH2_cur, A" class="DigNum (strict)"("DisabledEnum"=w1627) -> ()  [unwired: 2 in, 2 out]
            n1213 = property on="P3 CH2_selcur, A" class="DigNum (strict)"("DisabledEnum"=w1627) -> ()  [unwired: 2 in, 2 out]
            n1214 = property on="P3 CH2_counter" class="DigNum (strict)"("DisabledEnum"=w1627) -> ()  [unwired: 2 in, 2 out]
            n1215 = property on="P3 CH2_warning" class="Bool (strict)"("DisabledEnum"=w1627) -> ()  [unwired: 2 in, 2 out]
            n1216 = property on="P3 CH2" class="Bool (strict)"("DisabledEnum"=w1627) -> ()  [unwired: 2 in, 2 out]
          }
        }
        n1217 = local read "System Stop"() -> (w1625:bool)
      }
    }
  }
  n1218 = case shown="True" w41 {
    tunnel: w2 -> [_ w1637]
    tunnel: w47 -> [_ w1633]
    tunnel: w44 -> [_ w1632]
    frame False {
    }
    frame True {
      n1219 = while {
        tunnel: w1633 -> [w1664]
        tunnel: [w1669] -> w1636
        tunnel: [w1658] -> w1635
        tunnel: [w1643] -> w1634
        tunnel: w1637 -> [_]
        tunnel: w1632 -> [w1645]
        stop <- w1665 stop-if-true
        n1220 = flat-sequence {
          tunnel: w1664 -> [w1677]
          tunnel: [w1674] -> w1653
          tunnel: w1645 -> [w1671]
          tunnel: [w1670] -> w1651
          tunnel: [w1684] -> w1668
          tunnel: w1653 -> [w1683]
          tunnel: w1651 -> [w1680]
          tunnel: [w1679] -> w1650
          tunnel: [w1693] -> w1667
          tunnel: w1668 -> [w1692]
          tunnel: w1650 -> [w1691]
          tunnel: [w1690] -> w1649
          tunnel: w1667 -> [w1697]
          tunnel: [w1696] -> w1666
          tunnel: w1649 -> [w1695]
          tunnel: [w1694] -> w1648
          tunnel: [w1714] -> w1662
          tunnel: w1666 -> [w1716]
          tunnel: [w1713] -> w1660
          tunnel: [w1706] -> w1656
          tunnel: [w1708] -> w1655
          tunnel: [w1707] -> w1654
          tunnel: [w1703] -> w1652
          tunnel: w1648 -> [w1702]
          tunnel: [w1701] -> w1646
          tunnel: w1662 -> [w1778]
          tunnel: [w1778] -> w1661
          tunnel: w1660 -> [w1761]
          tunnel: [w1768] -> w1659
          tunnel: [w1766] -> w1657
          tunnel: w1656 -> [w1765]
          tunnel: w1655 -> [w1764]
          tunnel: w1654 -> [w1763]
          tunnel: w1652 -> [w1759]
          tunnel: [w1756] -> w1647
          tunnel: w1646 -> [w1756]
          tunnel: [w1784] -> w1669
          tunnel: w1661 -> [w1784]
          tunnel: [w1785] -> w1665
          tunnel: w1659 -> [w1783]
          tunnel: [w1783] -> w1658
          tunnel: w1657 -> [_]
          tunnel: w1647 -> [w1782]
          tunnel: [w1782] -> w1644
          frame #0 {
            n1221 = call <instrlib>:"niScope Configure Vertical.vi"("instrument handle"=w1677, "probe attenuation"=1.0 ("Probe Attenuation"), "vertical coupling"="AC/DC/Groun", "channels"="0" ("Channel Name"), "vertical range"="vertical range", "vertical offset"=0.0, "error in"=w1671) -> ("instrument handle out"=w1674:refnum<k15>, "error out"=w1670:errorcluster)  [unwired: 7 in]
          }
          frame #1 {
            w1689 = 0 items=["Positive", "Negative"] ("Trigger Slope")
            w1688 = u16 1 items=["AC"=0, "DC"=1, "HF Reject"=3, "LF Reject"=4, "AC Plus HF Reject"=1001] ("Coupling")
            n1222 = call-poly <instrlib>:"niScope Configure Trigger (poly).vi"("instrument handle"=w1683, "trigger window mode"=w1689, "trigger coupling"=w1688, "trigger source"="Trigger Source", "low level"="Low Level", "high level"="High Level", "error in"=w1680, "trigger holdoff"=0.0, "trigger delay"=0.0 ("Trigger Delay")) -> ("instrument handle out"=w1684:refnum<k15>, "error out"=w1679:errorcluster)  [unwired: 5 in]
          }
          frame #2 {
            n1223 = call <instrlib>:"niScope Initiate Acquisition.vi"("instrument handle"=w1692, "error in"=w1691) -> ("instrument handle out"=w1693:refnum<k15>, "error out"=w1690:errorcluster)  [unwired: 12 in]
          }
          frame #3 {
            n1224 = call-poly <instrlib>:"niScope Fetch (poly).vi"("timeout"=1.0, "error in"=w1695, "channels"="0", "instrument handle"=w1697) -> ("error out"=w1694:errorcluster, "waveform"=→"RealTime Waveform":T4, "instrument handle out"=w1696:refnum<k15>)  [unwired: 4 in, 1 out]
          }
          frame #4 {
            # "Во время триггера FALSE"
            n1225 = property class="niScope" props=["Auto Triggered", "Trigger Hysteresis"](reference=w1716) -> (reference out=w1715:refnum<k15>, "Auto Triggered"=w1712:bool)  [unwired: 1 in, 2 out]
            n1226 = case shown="\"Radio Selection P1 CH1\"" "Channel for SEU" {
              tunnel: [w1718 w1724 w1726 w1730] -> w1708
              tunnel: [w1719 w1723 w1727 w1731] -> w1707
              tunnel: [w1720 w1722 w1728 w1732] -> w1706
              tunnel: [w1717 w1721 w1725 w1729] -> w1704
              frame "Radio Selection P1 CH0", Default {
                n1227 = local read "P1 CH0_warning"() -> (w1717:bool)
                n1228 = local read "P1 CH0_cur, A"() -> (w1718:dbl)
                n1229 = local read "P1 CH0, V"() -> (w1719:dbl)
                n1230 = Get Date/Time In Seconds() -> (seconds since 1Jan1904=w1720:timestamp)
              }
              frame "Radio Selection P1 CH1" {
                n1231 = local read "P1 CH1_warning"() -> (w1721:bool)
                n1232 = local read "P1 CH1_cur, A"() -> (w1724:dbl)
                n1233 = local read "P1 CH1, V"() -> (w1723:dbl)
                n1234 = Get Date/Time In Seconds() -> (seconds since 1Jan1904=w1722:timestamp)
              }
              frame "Radio Selection P2 CH0" {
                n1235 = local read "P2 CH0_warning"() -> (w1725:bool)
                n1236 = local read "P2 CH0_cur, A"() -> (w1726:dbl)
                n1237 = local read "P2 CH0, V"() -> (w1727:dbl)
                n1238 = Get Date/Time In Seconds() -> (seconds since 1Jan1904=w1728:timestamp)
              }
              frame "Radio Selection P2 CH1" {
                n1239 = local read "P1 CH1_warning"() -> (w1729:bool)
                n1240 = local read "P2 CH1_cur, A"() -> (w1730:dbl)
                n1241 = local read "P2 CH1, V"() -> (w1731:dbl)
                n1242 = Get Date/Time In Seconds() -> (seconds since 1Jan1904=w1732:timestamp)
              }
            }
            n1243 = Not(x=w1712) -> (.not. x?=w1711:bool)
            n1244 = Not(x=w1704) -> (.not. x?=w1709:bool)
            n1245 = And(x=w1709, y=w1711) -> (x .and. y?=w1710:bool)
            n1246 = case shown="True" w1710 {
              tunnel: w1715 -> [w1736 w1751]
              tunnel: [w1736 w1743] -> w1714
              tunnel: [FALSE TRUE] -> w1713
              tunnel: ["" w1740] -> w1703
              tunnel: w1702 -> [w1733 w1739]
              tunnel: [w1733 w1737] -> w1701
              frame False {
              }
              frame True {
                w1742 = 6
                # "Регистрация SEU"
                n1247 = call-poly <instrlib>:"niScope Fetch (poly).vi"("timeout"=1.0, "error in"=w1739, "channels"="0", "instrument handle"=w1751) -> ("error out"=w1738:errorcluster, "waveform"=→"SEU Waveform":T4, "instrument handle out"=w1744:refnum<k15>)  [unwired: 4 in, 1 out]
                n1248 = call-poly <instrlib>:"niScope Fetch (poly).vi"("timeout"=1.0, "error in"=w1738, "numSamples"=1, "channels"="0", "instrument handle"=w1744) -> ("error out"=w1737:errorcluster, "wfm"=w1749:dbl[], "instrument handle out"=w1743:refnum<k15>)  [unwired: 3 in, 1 out]
                n1249 = Index Array(array=w1749, index=0) -> (element=w1741:dbl)
                "SEU Last Level" <- w1741
                n1250 = Number To Fractional String(number=w1741, width (-)=w1742, precision (6)=w1742) -> (F-format string=w1740:string)  [unwired: 1 in]
              }
            }
          }
          frame #5 {
            w1769 = 6
            w1773 = 0
            w1772 = 6
            w1760 = "\t"
            # "Регистрация SEU"
            n1251 = case shown="True" w1761 {
              tunnel: [w1779 w1780] -> w1762
              frame False {
                n1252 = local read "SEU_Counter"() -> (w1779:u32)
              }
              frame True {
                n1253 = local read "SEU_Counter"() -> (w1781:u32)
                n1254 = Increment(x=w1781) -> (x+1=w1780:u32)
                "SEU_Counter" <- w1780
              }
            }
            n1255 = Format Date/Time String(time format string (%c)="%H:%M:%S:%3u", seconds (now)=w1765) -> (date/time string=w1775:string)  [unwired: 1 in]
            n1256 = local read "SEU output file refnum"() -> (w1755:refnum<file>)
            n1257 = Number To Fractional String(number=w1763, width (-)=w1769, precision (6)=w1769) -> (F-format string=w1774:string)  [unwired: 1 in]
            n1258 = Number To Fractional String(number=w1764, width (-)=w1772, precision (6)=w1772) -> (F-format string=w1776:string)  [unwired: 1 in]
            n1259 = Number To Fractional String(number=w1762, width (-)=w1773, precision (6)=w1773) -> (F-format string=w1777:string)  [unwired: 1 in]
            n1260 = Select(t="???", s=w1761, f="") -> (s? t:f=w1758:string)
            n1261 = Concatenate Strings(w1775, w1760, w1774, w1760, w1776, w1760, w1777, w1760, w1759, w1760, w1758, "\r\n") -> (w1766:string)
            n1262 = Format Into String(initial string=w1755, w1766) -> (resulting string=w1768:refnum<file>)  [unwired: 2 in, 1 out]
            "SEU_warning" <- w1761
            "SEU" <- w1761
          }
          frame #6 {
            n1263 = local read "System Stop"() -> (w1785:bool)
          }
        }
        n1264 = Wait (ms)(milliseconds to wait=u32 1) -> ()  [unwired: 1 out]
        n1265 = call <vilib>:"Simple Error Handler.vi"("error in (no error)"=w1644) -> ("error out"=w1643:errorcluster)  [unwired: 1 in, 7 out]
        "NI Scope error out" <- w1643
      }
      n1266 = flat-sequence {
        tunnel: w1636 -> [w1642]
        tunnel: w1635 -> [w1641]
        tunnel: w1634 -> [w1640]
        frame #0 {
          n1267 = Close File(refnum=w1641) -> ()  [unwired: 1 in, 2 out]
          n1268 = call <instrlib>:"niScope Close.vi"("instrument handle"=w1642, "error in"=w1640) -> ("error out"=w1639:errorcluster)  [unwired: 13 in]
          n1269 = call <vilib>:"Simple Error Handler.vi"("error in (no error)"=w1639) -> ("error out"=w1638:errorcluster)  [unwired: 1 in, 7 out]
          n1270 = local write "NI Scope error out"(w1638) -> ()
        }
      }
    }
  }
  n1271 = while {
    shift-right: [w1829] -> _
    shift-left: w12 -> [w1835]
    shift-right: [w1828] -> _
    shift-left: w12 -> [w1834]
    shift-right: [w1830] -> _
    shift-left: w12 -> [w1833]
    shift-right: [w1831] -> _
    shift-left: w12 -> [w1832]
    shift-right: [w1824] -> _
    shift-left: w12 -> [w1825]
    shift-right: [w1822] -> _
    shift-left: w12 -> [w1823]
    shift-right: [w1820] -> _
    shift-left: w12 -> [w1821]
    shift-right: [w1818] -> _
    shift-left: w12 -> [w1819]
    tunnel: w2 -> [_]
    shift-right: [w1815] -> _
    shift-left: w12 -> [w1814]
    shift-right: [w1817] -> _
    shift-left: w12 -> [w1816]
    shift-right: [w1812] -> _
    shift-left: w12 -> [w1813]
    shift-right: [w1810] -> _
    shift-left: w12 -> [w1811]
    shift-right: [w1807] -> _
    shift-left: w12 -> [w1809]
    shift-right: [w1806] -> _
    shift-left: w12 -> [w1808]
    shift-right: [w1802] -> _
    shift-left: w12 -> [w1805]
    shift-right: [w1803] -> _
    shift-left: w12 -> [w1804]
    shift-right: [w1798] -> _
    shift-left: w12 -> [w1801]
    shift-right: [w1799] -> _
    shift-left: w12 -> [w1800]
    shift-right: [w1795] -> _
    shift-left: w12 -> [w1797]
    shift-right: [w1794] -> _
    shift-left: w12 -> [w1796]
    shift-right: [w1790] -> _
    shift-left: w12 -> [w1793]
    shift-right: [w1791] -> _
    shift-left: w12 -> [w1792]
    shift-right: [w1786] -> _
    shift-left: w12 -> [w1789]
    shift-right: [w1787] -> _
    shift-left: w12 -> [w1788]
    stop <- w1826 stop-if-true
    # "Включение / выключение каналов"
    n1272 = stacked-sequence {
      tunnel: w1835 -> [w1967 _]
      tunnel: [w1837 _] -> w1829
      tunnel: w1834 -> [w1960 _]
      tunnel: [w1838 _] -> w1828
      tunnel: w1833 -> [w1959 _]
      tunnel: w1832 -> [w1953 _]
      tunnel: ["POWER" _] -> w1831
      tunnel: [w1840 _] -> w1830
      tunnel: [_ w2016] -> w1826
      tunnel: w1825 -> [w1949 _]
      tunnel: [w1946 _] -> w1824
      tunnel: w1823 -> [w1945 _]
      tunnel: [w1940 _] -> w1822
      tunnel: w1821 -> [w1935 _]
      tunnel: [w1934 _] -> w1820
      tunnel: w1819 -> [w1929 _]
      tunnel: [w1930 _] -> w1818
      tunnel: w1814 -> [w1918 _]
      tunnel: [w1922 _] -> w1815
      tunnel: w1816 -> [w1926 _]
      tunnel: [w1925 _] -> w1817
      tunnel: w1813 -> [w1917 _]
      tunnel: [w1913 _] -> w1812
      tunnel: w1811 -> [w1909 _]
      tunnel: [w1910 _] -> w1810
      tunnel: w1809 -> [w1864 _]
      tunnel: w1808 -> [w1863 _]
      tunnel: [w1836 _] -> w1807
      tunnel: [w1862 _] -> w1806
      tunnel: w1805 -> [w1861 _]
      tunnel: w1804 -> [w1860 _]
      tunnel: [w1859 _] -> w1803
      tunnel: [w1858 _] -> w1802
      tunnel: w1801 -> [w1857 _]
      tunnel: w1800 -> [w1856 _]
      tunnel: [w1855 _] -> w1799
      tunnel: [w1854 _] -> w1798
      tunnel: w1797 -> [w1853 _]
      tunnel: w1796 -> [w1852 _]
      tunnel: [w1851 _] -> w1795
      tunnel: [w1850 _] -> w1794
      tunnel: w1793 -> [w1849 _]
      tunnel: w1792 -> [w1848 _]
      tunnel: [w1847 _] -> w1791
      tunnel: [w1846 _] -> w1790
      tunnel: w1789 -> [w1845 _]
      tunnel: w1788 -> [w1844 _]
      tunnel: [w1843 _] -> w1787
      tunnel: [w1842 _] -> w1786
      frame #0 {
        n1273 = local read "POWER"() -> (w1837:bool)
        n1274 = local read "POWER"() -> (w1836:bool)
        n1275 = local read "POWER"() -> (w1838:bool)
        n1276 = local read "POWER"() -> (w1840:bool)
        n1277 = local read "P1 CH0 Used"() -> (w1946:bool)
        n1278 = local read "P1 CH1 Used"() -> (w1940:bool)
        n1279 = local read "P1 CH2 Used"() -> (w1910:bool)
        n1280 = local read "P3 CH0 Used"() -> (w1862:bool)
        n1281 = local read "P2 CH0 Used"() -> (w1934:bool)
        n1282 = local read "P2 CH1 Used"() -> (w1930:bool)
        n1283 = local read "P2 CH2 Used"() -> (w1925:bool)
        n1284 = local read "P3 CH1 Used"() -> (w1859:bool)
        n1285 = local read "P3 CH2 Used"() -> (w1847:bool)
        n1286 = local read "P4 CH0 Used"() -> (w1855:bool)
        n1287 = local read "P4 CH1 Used"() -> (w1850:bool)
        n1288 = local read "P4 CH2 Used"() -> (w1843:bool)
        n1289 = local read "P1 CH2"() -> (w1913:bool)
        n1290 = local read "P2 CH2"() -> (w1922:bool)
        n1291 = local read "P3 CH1"() -> (w1858:bool)
        n1292 = local read "P3 CH2"() -> (w1846:bool)
        n1293 = local read "P4 CH1"() -> (w1851:bool)
        n1294 = local read "P4 CH2"() -> (w1842:bool)
        n1295 = local read "P4 CH0"() -> (w1854:bool)
        n1296 = local read "System Stop"() -> (w1942:bool)
        n1297 = local read "System Stop"() -> (w1907:bool)
        n1298 = local read "System Stop"() -> (w1883:bool)
        n1299 = local read "System Stop"() -> (w1906:bool)
        n1300 = local read "System Stop"() -> (w1904:bool)
        n1301 = local read "System Stop"() -> (w1937:bool)
        n1302 = local read "System Stop"() -> (w1841:bool)
        n1303 = local read "System Stop"() -> (w1905:bool)
        n1304 = local read "System Stop"() -> (w1950:bool)
        n1305 = local read "System Stop"() -> (w1887:bool)
        n1306 = local read "System Stop"() -> (w1878:bool)
        n1307 = Less?(x=w1840, y=w1959) -> (x < y?=w1943:bool)
        n1308 = Less?(x=w1913, y=w1917) -> (x < y?=w1912:bool)
        n1309 = Less?(x=w1858, y=w1861) -> (x < y?=w1882:bool)
        n1310 = Less?(x=w1837, y=w1967) -> (x < y?=w1933:bool)
        n1311 = Less?(x=w1922, y=w1918) -> (x < y?=w1923:bool)
        n1312 = Less?(x=w1838, y=w1960) -> (x < y?=w1939:bool)
        n1313 = Less?(x=w1846, y=w1849) -> (x < y?=w1901:bool)
        n1314 = Less?(x=w1934, y=w1935) -> (x < y?=w1936:bool)
        n1315 = Less?(x=w1851, y=w1853) -> (x < y?=w1889:bool)
        n1316 = Less?(x=w1842, y=w1845) -> (x < y?=w1894:bool)
        n1317 = Less?(x="POWER", y=w1953) -> (x < y?=w1951:bool)
        n1318 = Less?(x=w1854, y=w1857) -> (x < y?=w1885:bool)
        n1319 = Less?(x=w1855, y=w1856) -> (x < y?=w1888:bool)
        n1320 = Less?(x=w1836, y=w1864) -> (x < y?=w1877:bool)
        n1321 = Not(x=w1942) -> (.not. x?=w1958:bool)
        n1322 = Greater?(x=w1840, y=w1959) -> (0:w1957:bool)
        n1323 = Not(x=w1907) -> (.not. x?=w1915:bool)
        n1324 = Not(x=w1883) -> (.not. x?=w1871:bool)
        n1325 = Not(x="System Stop") -> (.not. x?=w1965:bool)
        n1326 = Not(x=w1906) -> (.not. x?=w1920:bool)
        n1327 = Not(x=w1937) -> (.not. x?=w1962:bool)
        n1328 = Greater?(x=w1913, y=w1917) -> (0:w1914:bool)
        n1329 = Greater?(x=w1858, y=w1861) -> (0:w1872:bool)
        n1330 = Not(x=w1904) -> (.not. x?=w1899:bool)
        n1331 = Greater?(x=w1837, y=w1967) -> (0:w1964:bool)
        n1332 = Greater?(x=w1922, y=w1918) -> (0:w1921:bool)
        n1333 = Not(x=w1841) -> (.not. x?=w1866:bool)
        n1334 = Not(x=w1905) -> (.not. x?=w1896:bool)
        n1335 = Not(x=w1950) -> (.not. x?=w1954:bool)
        n1336 = Greater?(x=w1838, y=w1960) -> (0:w1963:bool)
        n1337 = Not(x=w1887) -> (.not. x?=w1869:bool)
        n1338 = Greater?(x=w1846, y=w1849) -> (0:w1900:bool)
        n1339 = Greater?(x=w1851, y=w1853) -> (0:w1867:bool)
        n1340 = Greater?(x=w1842, y=w1845) -> (0:w1895:bool)
        n1341 = Greater?(x="POWER", y=w1953) -> (0:w1955:bool)
        n1342 = Not(x=w1878) -> (.not. x?=w1875:bool)
        n1343 = Greater?(x=w1854, y=w1857) -> (0:w1868:bool)
        n1344 = Less?(x=w1910, y=w1909) -> (x < y?=w1908:bool)
        n1345 = Less?(x=w1930, y=w1929) -> (x < y?=w1928:bool)
        n1346 = Less?(x=w1925, y=w1926) -> (x < y?=w1927:bool)
        n1347 = Less?(x=w1946, y=w1949) -> (x < y?=w1948:bool)
        n1348 = Less?(x=w1940, y=w1945) -> (x < y?=w1941:bool)
        n1349 = Greater?(x=w1836, y=w1864) -> (0:w1874:bool)
        n1350 = Less?(x=w1847, y=w1848) -> (x < y?=w1903:bool)
        n1351 = Less?(x=w1850, y=w1852) -> (x < y?=w1891:bool)
        n1352 = Less?(x=w1843, y=w1844) -> (x < y?=w1892:bool)
        n1353 = Less?(x=w1862, y=w1863) -> (x < y?=w1879:bool)
        n1354 = Less?(x=w1859, y=w1860) -> (x < y?=w1884:bool)
        n1355 = And(x=w1958, y=w1957) -> (x .and. y?=w1956:bool)
        n1356 = And(x=w1915, y=w1914) -> (x .and. y?=w1916:bool)
        n1357 = And(x=w1871, y=w1872) -> (x .and. y?=w1873:bool)
        n1358 = Compound Arithmetic op=OR(w1939, w1937, w1936) -> (w1938:bool)
        n1359 = And(x=w1965, y=w1964) -> (x .and. y?=w1966:bool)
        n1360 = And(x=w1920, y=w1921) -> (x .and. y?=w1919:bool)
        n1361 = And(x=w1962, y=w1963) -> (x .and. y?=w1961:bool)
        n1362 = Compound Arithmetic op=OR(w1912, w1907, w1908) -> (w1911:bool)
        n1363 = And(x=w1899, y=w1900) -> (x .and. y?=w1898:bool)
        n1364 = Compound Arithmetic op=OR(w1933, "System Stop", w1928) -> (w1931:bool)
        n1365 = Compound Arithmetic op=OR(w1923, w1906, w1927) -> (w1924:bool)
        n1366 = Compound Arithmetic op=OR(w1885, w1887, w1888) -> (w1886:bool)
        n1367 = And(x=w1866, y=w1867) -> (x .and. y?=w1865:bool)
        n1368 = And(x=w1896, y=w1895) -> (x .and. y?=w1897:bool)
        n1369 = And(x=w1954, y=w1955) -> (x .and. y?=w1952:bool)
        n1370 = And(x=w1869, y=w1868) -> (x .and. y?=w1870:bool)
        n1371 = Compound Arithmetic op=OR(w1901, w1904, w1903) -> (w1902:bool)
        n1372 = Compound Arithmetic op=OR(w1889, w1841, w1891) -> (w1890:bool)
        n1373 = Compound Arithmetic op=OR(w1894, w1905, w1892) -> (w1893:bool)
        n1374 = Compound Arithmetic op=OR(w1951, w1950, w1948) -> (w1947:bool)
        n1375 = And(x=w1875, y=w1874) -> (x .and. y?=w1876:bool)
        n1376 = Compound Arithmetic op=OR(w1943, w1942, w1941) -> (w1944:bool)
        n1377 = Compound Arithmetic op=OR(w1877, w1878, w1879) -> (w1880:bool)
        n1378 = Compound Arithmetic op=OR(w1882, w1883, w1884) -> (w1881:bool)
        n1379 = stacked-sequence {
          tunnel: w1952 -> [w2005]
          tunnel: w1947 -> [w2004]
          frame #0 {
            n1380 = case shown="True" w2005 {
              frame False {
              }
              frame True {
                # "ON"
                n1381 = local write "P1 CH0"(TRUE ("P1 CH0")) -> ()
              }
            }
            n1382 = case shown="True" w2004 {
              frame False {
              }
              frame True {
                # "OFF"
                n1383 = local write "P1 CH0"(FALSE ("P1 CH0")) -> ()
              }
            }
          }
        }
        n1384 = stacked-sequence {
          tunnel: w1956 -> [w2001]
          tunnel: w1944 -> [w2000]
          frame #0 {
            n1385 = case shown="True" w2001 {
              frame False {
              }
              frame True {
                # "ON"
                n1386 = local write "P1 CH1"(TRUE ("P1 CH1")) -> ()
              }
            }
            n1387 = case shown="True" w2000 {
              frame False {
              }
              frame True {
                # "OFF"
                n1388 = local write "P1 CH1"(FALSE ("P1 CH0")) -> ()
              }
            }
          }
        }
        n1389 = stacked-sequence {
          tunnel: w1961 -> [w2009]
          tunnel: w1938 -> [w2008]
          frame #0 {
            n1390 = case shown="True" w2009 {
              frame False {
              }
              frame True {
                # "ON"
                n1391 = local write "P2 CH0"(TRUE ("P2 CH0")) -> ()
              }
            }
            n1392 = case shown="True" w2008 {
              frame False {
              }
              frame True {
                # "OFF"
                n1393 = local write "P2 CH0"(FALSE ("P1 CH0")) -> ()
              }
            }
          }
        }
        n1394 = stacked-sequence {
          tunnel: w1916 -> [w1993]
          tunnel: w1911 -> [w1992]
          frame #0 {
            n1395 = case shown="True" w1993 {
              frame False {
              }
              frame True {
                # "ON"
                n1396 = local write "P1 CH2"(TRUE ("P2 CH1")) -> ()
              }
            }
            n1397 = case shown="True" w1992 {
              frame False {
              }
              frame True {
                # "OFF"
                n1398 = local write "P1 CH2"(FALSE ("P1 CH0")) -> ()
              }
            }
          }
        }
        n1399 = stacked-sequence {
          tunnel: w1966 -> [w2013]
          tunnel: w1931 -> [w2012]
          frame #0 {
            n1400 = case shown="True" w2013 {
              frame False {
              }
              frame True {
                # "ON"
                n1401 = local write "P2 CH1"(TRUE ("P2 CH1")) -> ()
              }
            }
            n1402 = case shown="True" w2012 {
              frame False {
              }
              frame True {
                # "OFF"
                n1403 = local write "P2 CH1"(FALSE ("P1 CH0")) -> ()
              }
            }
          }
        }
        n1404 = stacked-sequence {
          tunnel: w1919 -> [w1997]
          tunnel: w1924 -> [w1996]
          frame #0 {
            n1405 = case shown="True" w1997 {
              frame False {
              }
              frame True {
                # "ON"
                n1406 = local write "P2 CH2"(TRUE ("P2 CH1")) -> ()
              }
            }
            n1407 = case shown="True" w1996 {
              frame False {
              }
              frame True {
                # "OFF"
                n1408 = local write "P2 CH2"(FALSE ("P1 CH0")) -> ()
              }
            }
          }
        }
        n1409 = stacked-sequence {
          tunnel: w1876 -> [w1981]
          tunnel: w1880 -> [w1980]
          frame #0 {
            n1410 = case shown="True" w1981 {
              frame False {
              }
              frame True {
                # "ON"
                n1411 = local write "P3 CH0"(TRUE ("P1 CH0")) -> ()
              }
            }
            n1412 = case shown="True" w1980 {
              frame False {
              }
              frame True {
                # "OFF"
                n1413 = local write "P3 CH0"(FALSE ("P1 CH0")) -> ()
              }
            }
          }
        }
        n1414 = stacked-sequence {
          tunnel: w1873 -> [w1977]
          tunnel: w1881 -> [w1976]
          frame #0 {
            n1415 = case shown="True" w1977 {
              frame False {
              }
              frame True {
                # "ON"
                n1416 = local write "P3 CH1"(TRUE ("P1 CH1")) -> ()
              }
            }
            n1417 = case shown="True" w1976 {
              frame False {
              }
              frame True {
                # "OFF"
                n1418 = local write "P3 CH1"(FALSE ("P1 CH0")) -> ()
              }
            }
          }
        }
        n1419 = stacked-sequence {
          tunnel: w1870 -> [w1985]
          tunnel: w1886 -> [w1984]
          frame #0 {
            n1420 = case shown="True" w1985 {
              frame False {
              }
              frame True {
                # "ON"
                n1421 = local write "P4 CH0"(TRUE ("P2 CH0")) -> ()
              }
            }
            n1422 = case shown="True" w1984 {
              frame False {
              }
              frame True {
                # "OFF"
                n1423 = local write "P4 CH0"(FALSE ("P1 CH0")) -> ()
              }
            }
          }
        }
        n1424 = stacked-sequence {
          tunnel: w1898 -> [w1969]
          tunnel: w1902 -> [w1968]
          frame #0 {
            n1425 = case shown="True" w1969 {
              frame False {
              }
              frame True {
                # "ON"
                n1426 = local write "P3 CH2"(TRUE ("P2 CH1")) -> ()
              }
            }
            n1427 = case shown="True" w1968 {
              frame False {
              }
              frame True {
                # "OFF"
                n1428 = local write "P3 CH2"(FALSE ("P1 CH0")) -> ()
              }
            }
          }
        }
        n1429 = stacked-sequence {
          tunnel: w1865 -> [w1989]
          tunnel: w1890 -> [w1988]
          frame #0 {
            n1430 = case shown="True" w1989 {
              frame False {
              }
              frame True {
                # "ON"
                n1431 = local write "P4 CH1"(TRUE ("P2 CH1")) -> ()
              }
            }
            n1432 = case shown="True" w1988 {
              frame False {
              }
              frame True {
                # "OFF"
                n1433 = local write "P4 CH1"(FALSE ("P1 CH0")) -> ()
              }
            }
          }
        }
        n1434 = stacked-sequence {
          tunnel: w1897 -> [w1973]
          tunnel: w1893 -> [w1972]
          frame #0 {
            n1435 = case shown="True" w1973 {
              frame False {
              }
              frame True {
                # "ON"
                n1436 = local write "P4 CH2"(TRUE ("P2 CH1")) -> ()
              }
            }
            n1437 = case shown="True" w1972 {
              frame False {
              }
              frame True {
                # "OFF"
                n1438 = local write "P4 CH2"(FALSE ("P1 CH0")) -> ()
              }
            }
          }
        }
      }
      frame #1 {
        n1439 = local read "System Stop"() -> (w2016:bool)
      }
    }
    "Power OFF" <- w1826
    n1440 = Wait (ms)(milliseconds to wait=u32 1) -> ()  [unwired: 1 out]
  }
  n1441 = case shown="True" w24 {
    selector: w24 -> [w2017 w2020]
    tunnel: w29 -> [w2018 w2024]
    tunnel: w28 -> [w2019 w2023]
    tunnel: [w2019 w2022] -> w27
    tunnel: [w2018 w2021] -> w26
    tunnel: [w2017 w2020] -> w19
    tunnel: w1 -> [_ _]
    frame False {
    }
    frame True {
      n1442 = while {
        tunnel: [w2030] -> _
        tunnel: w2024 -> [w2029]
        tunnel: w2023 -> [w2028]
        tunnel: [w2027] -> w2022
        tunnel: [w2025] -> w2021
        stop <- w2030 stop-if-true
        n1443 = Wait (ms)(milliseconds to wait=u32 1) -> ()  [unwired: 1 out]
        n1444 = flat-sequence {
          tunnel: [w2036] -> w2030
          tunnel: w2029 -> [w2035]
          tunnel: w2028 -> [w2034]
          tunnel: [w2033] -> w2027
          tunnel: [w2032] -> w2026
          frame #0 {
            w2037 = T10 0 items=["Current", "Voltage"] ("measurement type")
            n1445 = call <instrlib>:"niDCPower Configure Current Limit.vi"("current limit"="P2 CH0_curlim, A", "channel name"="0", "instrument handle"=w2034) -> ("error out"=w2062:errorcluster, "instrument handle out"=w2081:refnum<k15>)  [unwired: 7 in]
            n1446 = call <instrlib>:"niDCPower Configure Current Limit.vi"("error in (no error)"=w2035, "current limit"="P2 CH1_curlim, A", "channel name"="1", "instrument handle"=w2034) -> ("instrument handle out"=w2067:refnum<k15>)  [unwired: 6 in, 1 out]
            n1447 = call <instrlib>:"niDCPower Configure Current Limit.vi"("current limit"="P2 CH2_curlim, A", "channel name"="2", "instrument handle"=w2034) -> ("instrument handle out"=w2047:refnum<k15>)  [unwired: 7 in, 1 out]
            n1448 = local read "Power OFF"() -> (w2064:bool)
            n1449 = local read "Power OFF"() -> (w2050:bool)
            n1450 = local read "Power OFF"() -> (w2074:bool)
            n1451 = call <instrlib>:"niDCPower Configure Voltage Level.vi"("error in (no error)"=w2062, "voltage level"="P2 CH0, V", "channel name"="0", "instrument handle"=w2081) -> ("error out"=w2078:errorcluster, "instrument handle out"=w2077:refnum<k15>)  [unwired: 6 in]
            n1452 = call <instrlib>:"niDCPower Configure Voltage Level.vi"("voltage level"="P2 CH1, V", "channel name"="1", "instrument handle"=w2067) -> ("instrument handle out"=w2070:refnum<k15>)  [unwired: 7 in, 1 out]
            n1453 = call <instrlib>:"niDCPower Configure Voltage Level.vi"("voltage level"="P2 CH2, V", "channel name"="2", "instrument handle"=w2047) -> ("instrument handle out"=w2044:refnum<k15>)  [unwired: 7 in, 1 out]
            n1454 = Select(t=FALSE, s=w2064, f="P2 CH1") -> (s? t:f=w2063:bool)
            n1455 = Select(t=FALSE, s=w2050, f="P2 CH2") -> (s? t:f=w2051:bool)
            n1456 = Select(t=FALSE, s=w2074, f="P2 CH0") -> (s? t:f=w2073:bool)
            n1457 = call <instrlib>:"niDCPower Configure Output Enabled.vi"("error in (no error)"=w2078, "output enabled"=w2073, "channel name"="0", "instrument handle"=w2077) -> ("error out"=w2075:errorcluster, "instrument handle out"=w2076:refnum<k15>)  [unwired: 6 in]
            n1458 = call <instrlib>:"niDCPower Configure Output Enabled.vi"("output enabled"=w2063, "channel name"="1", "instrument handle"=w2070) -> ("instrument handle out"=w2071:refnum<k15>)  [unwired: 7 in, 1 out]
            n1459 = call <instrlib>:"niDCPower Configure Output Enabled.vi"("output enabled"=w2051, "channel name"="2", "instrument handle"=w2044) -> ("instrument handle out"=w2043:refnum<k15>)  [unwired: 7 in, 1 out]
            n1460 = call <instrlib>:"niDCPower Measure.vi"("error in (no error)"=w2075, "measurement type"=w2037, "channel name"="0", "instrument handle"=w2076) -> ("error out"=w2032:errorcluster, "measurement"=→"P2 CH0_cur, A" →"P2 CH0_char":dbl, "instrument handle out"=w2033:refnum<k15>)  [unwired: 5 in]
            n1461 = call <instrlib>:"niDCPower Measure.vi"("measurement type"=w2037, "channel name"="1", "instrument handle"=w2071) -> ("measurement"=→"P2 CH1_cur, A" →"P2 CH1_char":dbl)  [unwired: 6 in, 2 out]
            n1462 = call <instrlib>:"niDCPower Measure.vi"("measurement type"=w2037, "channel name"="2", "instrument handle"=w2043) -> ("measurement"=→"P2 CH2_cur, A" →"P2 CH2_char":dbl)  [unwired: 6 in, 2 out]
            n1463 = local read "Power OFF"() -> (w2036:bool)
          }
        }
        n1464 = call <vilib>:"Simple Error Handler.vi"("error in (no error)"=w2026) -> ("error out"=w2025:errorcluster)  [unwired: 1 in, 7 out]
        "DC Power 2 error out" <- w2025
      }
    }
  }
  n1465 = case shown="True" w16 {
    selector: w16 -> [w2083 w2086]
    tunnel: w21 -> [w2084 w2090]
    tunnel: w22 -> [w2085 w2089]
    tunnel: [w2085 w2088] -> w18
    tunnel: [w2084 w2087] -> w17
    tunnel: w1 -> [_ _]
    tunnel: [w2083 w2086] -> w11
    frame False {
    }
    frame True {
      n1466 = while {
        tunnel: [w2096] -> _
        tunnel: w2090 -> [w2095]
        tunnel: w2089 -> [w2094]
        tunnel: [w2093] -> w2088
        tunnel: [w2091] -> w2087
        stop <- w2096 stop-if-true
        n1467 = Wait (ms)(milliseconds to wait=u32 1) -> ()  [unwired: 1 out]
        n1468 = flat-sequence {
          tunnel: [w2102] -> w2096
          tunnel: w2095 -> [w2101]
          tunnel: w2094 -> [w2100]
          tunnel: [w2099] -> w2093
          tunnel: [w2098] -> w2092
          frame #0 {
            w2103 = T10 0 items=["Current", "Voltage"] ("measurement type")
            n1469 = call <instrlib>:"niDCPower Configure Current Limit.vi"("current limit"="P3 CH0_curlim, A", "channel name"="0", "instrument handle"=w2100) -> ("error out"=w2128:errorcluster, "instrument handle out"=w2147:refnum<k15>)  [unwired: 7 in]
            n1470 = call <instrlib>:"niDCPower Configure Current Limit.vi"("error in (no error)"=w2101, "current limit"="P3 CH1_curlim, A", "channel name"="1", "instrument handle"=w2100) -> ("instrument handle out"=w2133:refnum<k15>)  [unwired: 6 in, 1 out]
            n1471 = call <instrlib>:"niDCPower Configure Current Limit.vi"("current limit"="P3 CH2_curlim, A", "channel name"="2", "instrument handle"=w2100) -> ("instrument handle out"=w2113:refnum<k15>)  [unwired: 7 in, 1 out]
            n1472 = local read "Power OFF"() -> (w2130:bool)
            n1473 = local read "Power OFF"() -> (w2116:bool)
            n1474 = local read "Power OFF"() -> (w2140:bool)
            n1475 = call <instrlib>:"niDCPower Configure Voltage Level.vi"("error in (no error)"=w2128, "voltage level"="P3 CH0, V", "channel name"="0", "instrument handle"=w2147) -> ("error out"=w2144:errorcluster, "instrument handle out"=w2143:refnum<k15>)  [unwired: 6 in]
            n1476 = call <instrlib>:"niDCPower Configure Voltage Level.vi"("voltage level"="P3 CH1, V", "channel name"="1", "instrument handle"=w2133) -> ("instrument handle out"=w2136:refnum<k15>)  [unwired: 7 in, 1 out]
            n1477 = call <instrlib>:"niDCPower Configure Voltage Level.vi"("voltage level"="P3 CH2, V", "channel name"="2", "instrument handle"=w2113) -> ("instrument handle out"=w2110:refnum<k15>)  [unwired: 7 in, 1 out]
            n1478 = Select(t=FALSE, s=w2130, f="P3 CH1") -> (s? t:f=w2129:bool)
            n1479 = Select(t=FALSE, s=w2116, f="P3 CH2") -> (s? t:f=w2117:bool)
            n1480 = Select(t=FALSE, s=w2140, f="P3 CH0") -> (s? t:f=w2139:bool)
            n1481 = call <instrlib>:"niDCPower Configure Output Enabled.vi"("error in (no error)"=w2144, "output enabled"=w2139, "channel name"="0", "instrument handle"=w2143) -> ("error out"=w2141:errorcluster, "instrument handle out"=w2142:refnum<k15>)  [unwired: 6 in]
            n1482 = call <instrlib>:"niDCPower Configure Output Enabled.vi"("output enabled"=w2129, "channel name"="1", "instrument handle"=w2136) -> ("instrument handle out"=w2137:refnum<k15>)  [unwired: 7 in, 1 out]
            n1483 = call <instrlib>:"niDCPower Configure Output Enabled.vi"("output enabled"=w2117, "channel name"="2", "instrument handle"=w2110) -> ("instrument handle out"=w2109:refnum<k15>)  [unwired: 7 in, 1 out]
            n1484 = call <instrlib>:"niDCPower Measure.vi"("error in (no error)"=w2141, "measurement type"=w2103, "channel name"="0", "instrument handle"=w2142) -> ("error out"=w2098:errorcluster, "measurement"=→"P3 CH0_cur, A" →"P3 CH0_char":dbl, "instrument handle out"=w2099:refnum<k15>)  [unwired: 5 in]
            n1485 = call <instrlib>:"niDCPower Measure.vi"("measurement type"=w2103, "channel name"="1", "instrument handle"=w2137) -> ("measurement"=→"P3 CH1_cur, A" →"P3 CH1_char":dbl)  [unwired: 6 in, 2 out]
            n1486 = call <instrlib>:"niDCPower Measure.vi"("measurement type"=w2103, "channel name"="2", "instrument handle"=w2109) -> ("measurement"=→"P3 CH2_cur, A" →"P3 CH2_char":dbl)  [unwired: 6 in, 2 out]
            n1487 = local read "Power OFF"() -> (w2102:bool)
          }
        }
        n1488 = call <vilib>:"Simple Error Handler.vi"("error in (no error)"=w2092) -> ("error out"=w2091:errorcluster)  [unwired: 1 in, 7 out]
        "DC Power 3 error out" <- w2091
      }
    }
  }
  n1489 = case shown="True" w25 {
    selector: w25 -> [w2149 w2152]
    tunnel: [w2151 w2157] -> w51
    tunnel: w50 -> [w2151 w2156]
    tunnel: [w2150 w2155] -> w49
    tunnel: w48 -> [w2150 w2154]
    tunnel: w1 -> [_ w2153]
    tunnel: [w2149 w2152] -> w20
    frame False {
    }
    frame True {
      n1490 = while {
        tunnel: w2156 -> [w2164]
        tunnel: [w2163] -> _
        tunnel: [w2161] -> w2157
        tunnel: [w2158] -> w2155
        tunnel: w2154 -> [w2160]
        tunnel: w2153 -> [_]
        stop <- w2163 stop-if-true
        # "Инициализация источников"
        n1491 = Wait (ms)(milliseconds to wait=u32 1) -> ()  [unwired: 1 out]
        n1492 = flat-sequence {
          tunnel: w2164 -> [w2165]
          tunnel: [w2193] -> w2163
          tunnel: [w2184] -> w2161
          tunnel: [w2183] -> w2159
          tunnel: w2160 -> [w2182]
          frame #0 {
            w2166 = T10 0 items=["Current", "Voltage"] ("measurement type")
            n1493 = local read "Power OFF"() -> (w2186:bool)
            n1494 = call <instrlib>:"niDCPower Configure Current Limit.vi"("current limit"="P1 CH2_curlim, A", "channel name"="2", "instrument handle"=w2165) -> ("instrument handle out"=w2172:refnum<k15>)  [unwired: 7 in, 1 out]
            n1495 = call <instrlib>:"niDCPower Configure Current Limit.vi"("error in (no error)"=w2182, "current limit"="P1 CH0_curlim, A", "channel name"="0", "instrument handle"=w2165) -> ("error out"=w2181:errorcluster, "instrument handle out"=w2207:refnum<k15>)  [unwired: 6 in]
            n1496 = call <instrlib>:"niDCPower Configure Current Limit.vi"("current limit"="P1 CH1_curlim, A", "channel name"="1", "instrument handle"=w2165) -> ("instrument handle out"=w2204:refnum<k15>)  [unwired: 7 in, 1 out]
            n1497 = local read "Power OFF"() -> (w2192:bool)
            n1498 = local read "Power OFF"() -> (w2178:bool)
            n1499 = call <instrlib>:"niDCPower Configure Voltage Level.vi"("voltage level"="P1 CH2, V", "channel name"="2", "instrument handle"=w2172) -> ("instrument handle out"=w2175:refnum<k15>)  [unwired: 7 in, 1 out]
            n1500 = call <instrlib>:"niDCPower Configure Voltage Level.vi"("error in (no error)"=w2181, "voltage level"="P1 CH0, V", "channel name"="0", "instrument handle"=w2207) -> ("error out"=w2211:errorcluster, "instrument handle out"=w2212:refnum<k15>)  [unwired: 6 in]
            n1501 = call <instrlib>:"niDCPower Configure Voltage Level.vi"("voltage level"="P1 CH1, V", "channel name"="1", "instrument handle"=w2204) -> ("instrument handle out"=w2210:refnum<k15>)  [unwired: 7 in, 1 out]
            n1502 = Select(t=FALSE, s=w2186, f="P1 CH0") -> (s? t:f=w2185:bool)
            n1503 = Select(t=FALSE, s=w2192, f="P1 CH1") -> (s? t:f=w2189:bool)
            n1504 = Select(t=FALSE, s=w2178, f="P1 CH2") -> (s? t:f=w2179:bool)
            n1505 = call <instrlib>:"niDCPower Configure Output Enabled.vi"("output enabled"=w2179, "channel name"="2", "instrument handle"=w2175) -> ("instrument handle out"=w2176:refnum<k15>)  [unwired: 7 in, 1 out]
            n1506 = call <instrlib>:"niDCPower Configure Output Enabled.vi"("error in (no error)"=w2211, "output enabled"=w2185, "channel name"="0", "instrument handle"=w2212) -> ("error out"=w2214:errorcluster, "instrument handle out"=w2213:refnum<k15>)  [unwired: 6 in]
            n1507 = call <instrlib>:"niDCPower Configure Output Enabled.vi"("output enabled"=w2189, "channel name"="1", "instrument handle"=w2210) -> ("instrument handle out"=w2215:refnum<k15>)  [unwired: 7 in, 1 out]
            n1508 = call <instrlib>:"niDCPower Measure.vi"("measurement type"=w2166, "channel name"="2", "instrument handle"=w2176) -> ("measurement"=→"P1 CH2_cur, A" →"P1 CH2_char":dbl)  [unwired: 6 in, 2 out]
            n1509 = call <instrlib>:"niDCPower Measure.vi"("error in (no error)"=w2214, "measurement type"=w2166, "channel name"="0", "instrument handle"=w2213) -> ("error out"=w2183:errorcluster, "measurement"=→"P1 CH0_cur, A" →"P1 CH0_char":dbl, "instrument handle out"=w2184:refnum<k15>)  [unwired: 5 in]
            n1510 = call <instrlib>:"niDCPower Measure.vi"("measurement type"=w2166, "channel name"="1", "instrument handle"=w2215) -> ("measurement"=→"P1 CH1_cur, A" →"P1 CH1_char":dbl)  [unwired: 6 in, 2 out]
            n1511 = local read "Power OFF"() -> (w2193:bool)
          }
        }
        n1512 = call <vilib>:"Simple Error Handler.vi"("error in (no error)"=w2159) -> ("error out"=w2158:errorcluster)  [unwired: 1 in, 7 out]
        "DC Power 1 error out" <- w2158
      }
    }
  }
  n1513 = case shown="True" w13 {
    selector: w13 -> [w2216 w2219]
    tunnel: w14 -> [w2217 w2223]
    tunnel: w15 -> [w2218 w2222]
    tunnel: [w2218 w2221] -> w10
    tunnel: [w2217 w2220] -> w9
    tunnel: w1 -> [_ _]
    tunnel: [w2216 w2219] -> w8
    frame False {
    }
    frame True {
      n1514 = while {
        tunnel: [w2229] -> _
        tunnel: w2223 -> [w2228]
        tunnel: w2222 -> [w2227]
        tunnel: [w2226] -> w2221
        tunnel: [w2224] -> w2220
        stop <- w2229 stop-if-true
        n1515 = Wait (ms)(milliseconds to wait=u32 1) -> ()  [unwired: 1 out]
        n1516 = flat-sequence {
          tunnel: [w2235] -> w2229
          tunnel: w2228 -> [w2234]
          tunnel: w2227 -> [w2233]
          tunnel: [w2232] -> w2226
          tunnel: [w2231] -> w2225
          frame #0 {
            w2236 = T10 0 items=["Current", "Voltage"] ("measurement type")
            n1517 = call <instrlib>:"niDCPower Configure Current Limit.vi"("current limit"="P4 CH0_curlim, A", "channel name"="0", "instrument handle"=w2233) -> ("error out"=w2261:errorcluster, "instrument handle out"=w2280:refnum<k15>)  [unwired: 7 in]
            n1518 = call <instrlib>:"niDCPower Configure Current Limit.vi"("error in (no error)"=w2234, "current limit"="P4 CH1_curlim, A", "channel name"="1", "instrument handle"=w2233) -> ("instrument handle out"=w2266:refnum<k15>)  [unwired: 6 in, 1 out]
            n1519 = call <instrlib>:"niDCPower Configure Current Limit.vi"("current limit"="P4 CH2_curlim, A", "channel name"="2", "instrument handle"=w2233) -> ("instrument handle out"=w2246:refnum<k15>)  [unwired: 7 in, 1 out]
            n1520 = local read "Power OFF"() -> (w2263:bool)
            n1521 = local read "Power OFF"() -> (w2249:bool)
            n1522 = local read "Power OFF"() -> (w2273:bool)
            n1523 = call <instrlib>:"niDCPower Configure Voltage Level.vi"("error in (no error)"=w2261, "voltage level"="P4 CH0, V", "channel name"="0", "instrument handle"=w2280) -> ("error out"=w2277:errorcluster, "instrument handle out"=w2276:refnum<k15>)  [unwired: 6 in]
            n1524 = call <instrlib>:"niDCPower Configure Voltage Level.vi"("voltage level"="P4 CH1, V", "channel name"="1", "instrument handle"=w2266) -> ("instrument handle out"=w2269:refnum<k15>)  [unwired: 7 in, 1 out]
            n1525 = call <instrlib>:"niDCPower Configure Voltage Level.vi"("voltage level"="P4 CH2, V", "channel name"="2", "instrument handle"=w2246) -> ("instrument handle out"=w2243:refnum<k15>)  [unwired: 7 in, 1 out]
            n1526 = Select(t=FALSE, s=w2263, f="P4 CH1") -> (s? t:f=w2262:bool)
            n1527 = Select(t=FALSE, s=w2249, f="P4 CH2") -> (s? t:f=w2250:bool)
            n1528 = Select(t=FALSE, s=w2273, f="P4 CH0") -> (s? t:f=w2272:bool)
            n1529 = call <instrlib>:"niDCPower Configure Output Enabled.vi"("error in (no error)"=w2277, "output enabled"=w2272, "channel name"="0", "instrument handle"=w2276) -> ("error out"=w2274:errorcluster, "instrument handle out"=w2275:refnum<k15>)  [unwired: 6 in]
            n1530 = call <instrlib>:"niDCPower Configure Output Enabled.vi"("output enabled"=w2262, "channel name"="1", "instrument handle"=w2269) -> ("instrument handle out"=w2270:refnum<k15>)  [unwired: 7 in, 1 out]
            n1531 = call <instrlib>:"niDCPower Configure Output Enabled.vi"("output enabled"=w2250, "channel name"="2", "instrument handle"=w2243) -> ("instrument handle out"=w2242:refnum<k15>)  [unwired: 7 in, 1 out]
            n1532 = call <instrlib>:"niDCPower Measure.vi"("error in (no error)"=w2274, "measurement type"=w2236, "channel name"="0", "instrument handle"=w2275) -> ("error out"=w2231:errorcluster, "measurement"=→"P4 CH0_cur, A" →"P4 CH0_char":dbl, "instrument handle out"=w2232:refnum<k15>)  [unwired: 5 in]
            n1533 = call <instrlib>:"niDCPower Measure.vi"("measurement type"=w2236, "channel name"="1", "instrument handle"=w2270) -> ("measurement"=→"P4 CH1_cur, A" →"P4 CH1_char":dbl)  [unwired: 6 in, 2 out]
            n1534 = call <instrlib>:"niDCPower Measure.vi"("measurement type"=w2236, "channel name"="2", "instrument handle"=w2242) -> ("measurement"=→"P4 CH2_cur, A" →"P4 CH2_char":dbl)  [unwired: 6 in, 2 out]
            n1535 = local read "Power OFF"() -> (w2235:bool)
          }
        }
        n1536 = call <vilib>:"Simple Error Handler.vi"("error in (no error)"=w2225) -> ("error out"=w2224:errorcluster)  [unwired: 1 in, 7 out]
        "DC Power 4 error out" <- w2224
      }
    }
  }
  n1537 = while {
    shift-right: [w2306] -> _
    shift-left: w7 -> [w2308]
    tunnel: [w2298] -> w23
    tunnel: [w2307] -> w52
    shift-right: [w2304] -> _
    shift-left: w7 -> [w2305]
    shift-right: [w2302] -> _
    shift-left: w7 -> [w2303]
    shift-right: [w2301] -> _
    shift-left: w7 -> [w2300]
    tunnel: w2 -> [_]
    tunnel: w2 -> [_]
    tunnel: w2 -> [_]
    shift-right: [w2295] -> _
    shift-left: w7 -> [w2297]
    shift-right: [w2294] -> _
    shift-left: w7 -> [w2296]
    shift-right: [w2287] -> _
    shift-left: w7 -> [w2293]
    shift-right: [w2285] -> _
    shift-left: w7 -> [w2292]
    shift-right: [w2286] -> _
    shift-left: w7 -> [w2291]
    shift-right: [w2284] -> _
    shift-left: w7 -> [w2290]
    shift-right: [w2283] -> _
    shift-left: w7 -> [w2289]
    shift-right: [w2282] -> _
    shift-left: w7 -> [w2288]
    stop <- w2298 stop-if-true
    n1538 = Wait (ms)(milliseconds to wait="SEL Time Cycle") -> ()  [unwired: 1 out]
    n1539 = stacked-sequence {
      seq-local: [w2336 _ _ _] -> [_ _ w2805 _]
      seq-local: [w2335 _ _ _] -> [_ _ w2802 _]
      seq-local: [w2334 _ _ _] -> [_ _ w2800 _]
      seq-local: [w2333 _ _ _] -> [_ _ w2799 _]
      seq-local: [w2332 _ _ _] -> [_ _ w2792 _]
      seq-local: [w2327 _ _ _] -> [_ _ w2793 _]
      seq-local: [w2320 _ _ _] -> [_ _ w2784 _]
      seq-local: [w2317 _ _ _] -> [_ _ w2781 _]
      seq-local: [w2315 _ _ _] -> [_ _ w2783 _]
      seq-local: [w2313 _ _ _] -> [_ _ w2782 _]
      seq-local: [w2311 _ _ _] -> [_ _ w2780 _]
      seq-local: [w2310 _ _ _] -> [_ _ w2779 _]
      tunnel: w2308 -> [w2344 _ _ _]
      tunnel: [_ _ _ w2880] -> w2298
      tunnel: [_ w2764 _ _] -> w2307
      tunnel: [_ _ w2807 _] -> w2306
      tunnel: w2305 -> [w2342 _ _ _]
      tunnel: [_ _ w2801 _] -> w2304
      tunnel: w2303 -> [w2341 _ _ _]
      tunnel: [_ _ w2803 _] -> w2302
      tunnel: [_ _ w2804 _] -> w2301
      tunnel: w2300 -> [w2337 _ _ _]
      tunnel: w2297 -> [w2331 _ _ _]
      tunnel: w2296 -> [w2328 _ _ _]
      tunnel: [_ _ w2791 _] -> w2295
      tunnel: [_ _ w2790 _] -> w2294
      tunnel: w2293 -> [w2319 _ _ _]
      tunnel: w2292 -> [w2318 _ _ _]
      tunnel: w2291 -> [w2316 _ _ _]
      tunnel: w2290 -> [w2314 _ _ _]
      tunnel: w2289 -> [w2312 _ _ _]
      tunnel: w2288 -> [w2309 _ _ _]
      tunnel: [_ _ w2778 _] -> w2287
      tunnel: [_ _ w2777 _] -> w2286
      tunnel: [_ _ w2776 _] -> w2285
      tunnel: [_ _ w2775 _] -> w2284
      tunnel: [_ _ w2774 _] -> w2283
      tunnel: [_ _ w2773 _] -> w2282
      frame #0 {
        # "Детектирование SEL"
        # "Детектирование SEL"
        n1540 = local read "P2 CH0"() -> (w2335:bool)
        n1541 = local read "P2 CH2"() -> (w2327:bool)
        n1542 = local read "P4 CH0"() -> (w2317:bool)
        n1543 = local read "P1 CH1"() -> (w2334:bool)
        n1544 = local read "P2 CH1"() -> (w2336:bool)
        n1545 = local read "P2 CH2"() -> (w2310:bool)
        n1546 = local read "P1 CH2"() -> (w2332:bool)
        n1547 = local read "P3 CH1"() -> (w2315:bool)
        n1548 = local read "P4 CH1"() -> (w2313:bool)
        n1549 = local read "P3 CH2"() -> (w2311:bool)
        n1550 = flat-sequence {
          tunnel: w2339 -> [w2505]
          frame #0 {
            n1551 = case shown="True" w2505 {
              frame False {
              }
              frame True {
                n1552 = Wait (ms)(milliseconds to wait=u32 50) -> ()  [unwired: 1 out]
              }
            }
          }
          frame #1 {
            n1553 = local read "P1 CH1_cur, A"() -> (w2510:dbl)
            n1554 = local read "SIM_SEL"() -> (w2508:bool)
            n1555 = Greater Or Equal?(x=w2510, y="P1 CH1_selcur, A") -> (x >= y?=w2511:bool)
            n1556 = Or(x=w2508, y=w2511) -> (x .or. y?=→"P1 CH1_warning":bool)
          }
          frame #2 {
            n1557 = local read "Считать SIM_SEL"() -> (w2517:bool)
            n1558 = local read "SIM_SEL"() -> (w2516:bool)
            n1559 = local read "P1 CH1_warning"() -> (w2512:bool)
            n1560 = Not(x=w2516) -> (.not. x?=w2515:bool)
            n1561 = Select(t=TRUE, s=w2517, f=w2515) -> (s? t:f=w2513:bool)
            n1562 = And(x=w2512, y=w2513) -> (x .and. y?=w2518:bool)
            n1563 = case shown="True" w2518 {
              frame False {
              }
              frame True {
                n1564 = local read "P1 CH1_counter"() -> (w2520:u32)
                n1565 = Increment(x=w2520) -> (x+1=→"P1 CH1_counter":u32)
              }
            }
          }
        }
        n1566 = flat-sequence {
          tunnel: w2340 -> [w2489]
          frame #0 {
            n1567 = case shown="True" w2489 {
              frame False {
              }
              frame True {
                n1568 = Wait (ms)(milliseconds to wait=u32 50) -> ()  [unwired: 1 out]
              }
            }
          }
          frame #1 {
            n1569 = local read "P2 CH0_cur, A"() -> (w2495:dbl)
            n1570 = local read "SIM_SEL"() -> (w2492:bool)
            n1571 = Greater Or Equal?(x=w2495, y="P2 CH0_selcur, A") -> (x >= y?=w2494:bool)
            n1572 = Or(x=w2492, y=w2494) -> (x .or. y?=→"P2 CH0_warning":bool)
          }
          frame #2 {
            n1573 = local read "Считать SIM_SEL"() -> (w2499:bool)
            n1574 = local read "SIM_SEL"() -> (w2500:bool)
            n1575 = local read "P2 CH0_warning"() -> (w2496:bool)
            n1576 = Not(x=w2500) -> (.not. x?=w2501:bool)
            n1577 = Select(t=TRUE, s=w2499, f=w2501) -> (s? t:f=w2498:bool)
            n1578 = And(x=w2496, y=w2498) -> (x .and. y?=w2497:bool)
            n1579 = case shown="True" w2497 {
              frame False {
              }
              frame True {
                n1580 = local read "P2 CH0_counter"() -> (w2504:u32)
                n1581 = Increment(x=w2504) -> (x+1=→"P2 CH0_counter":u32)
              }
            }
          }
        }
        n1582 = flat-sequence {
          tunnel: w2343 -> [w2521]
          frame #0 {
            n1583 = case shown="True" w2521 {
              frame False {
              }
              frame True {
                n1584 = Wait (ms)(milliseconds to wait=u32 50) -> ()  [unwired: 1 out]
              }
            }
          }
          frame #1 {
            n1585 = local read "P1 CH0_cur, A"() -> (w2527:dbl)
            n1586 = Greater Or Equal?(x=w2527, y="P1 CH0_selcur, A") -> (x >= y?=w2526:bool)
            n1587 = Or(x="SIM_SEL", y=w2526) -> (x .or. y?=→"P1 CH0_warning":bool)
          }
          frame #2 {
            n1588 = local read "SIM_SEL"() -> (w2533:bool)
            n1589 = local read "P1 CH0_warning"() -> (w2528:bool)
            n1590 = Not(x=w2533) -> (.not. x?=w2532:bool)
            n1591 = Select(t=TRUE, s="Считать SIM_SEL", f=w2532) -> (s? t:f=w2529:bool)
            n1592 = And(x=w2528, y=w2529) -> (x .and. y?=w2534:bool)
            n1593 = case shown="True" w2534 {
              frame False {
              }
              frame True {
                n1594 = local read "P1 CH0_counter"() -> (w2536:u32)
                n1595 = Increment(x=w2536) -> (x+1=→"P1 CH0_counter":u32)
              }
            }
          }
        }
        n1596 = flat-sequence {
          tunnel: w2329 -> [w2441]
          frame #0 {
            n1597 = case shown="True" w2441 {
              frame False {
              }
              frame True {
                n1598 = Wait (ms)(milliseconds to wait=u32 50) -> ()  [unwired: 1 out]
              }
            }
          }
          frame #1 {
            n1599 = local read "P2 CH2_cur, A"() -> (w2445:dbl)
            n1600 = local read "SIM_SEL"() -> (w2443:bool)
            n1601 = Greater Or Equal?(x=w2445, y="P2 CH2_selcur, A") -> (x >= y?=w2446:bool)
            n1602 = Or(x=w2443, y=w2446) -> (x .or. y?=→"P2 CH2_warning":bool)
          }
          frame #2 {
            n1603 = local read "Считать SIM_SEL"() -> (w2454:bool)
            n1604 = local read "SIM_SEL"() -> (w2453:bool)
            n1605 = local read "P2 CH2_warning"() -> (w2448:bool)
            n1606 = Not(x=w2453) -> (.not. x?=w2452:bool)
            n1607 = Select(t=TRUE, s=w2454, f=w2452) -> (s? t:f=w2450:bool)
            n1608 = And(x=w2448, y=w2450) -> (x .and. y?=w2449:bool)
            n1609 = case shown="True" w2449 {
              frame False {
              }
              frame True {
                n1610 = local read "P2 CH2_counter"() -> (w2456:u32)
                n1611 = Increment(x=w2456) -> (x+1=→"P2 CH2_counter":u32)
              }
            }
          }
        }
        n1612 = flat-sequence {
          tunnel: w2321 -> [w2425]
          frame #0 {
            n1613 = case shown="True" w2425 {
              frame False {
              }
              frame True {
                n1614 = Wait (ms)(milliseconds to wait=u32 50) -> ()  [unwired: 1 out]
              }
            }
          }
          frame #1 {
            n1615 = local read "P3 CH0_cur, A"() -> (w2431:dbl)
            n1616 = local read "SIM_SEL"() -> (w2427:bool)
            n1617 = Greater Or Equal?(x=w2431, y="P3 CH0_selcur, A") -> (x >= y?=w2430:bool)
            n1618 = Or(x=w2427, y=w2430) -> (x .or. y?=→"P3 CH0_warning":bool)
          }
          frame #2 {
            n1619 = local read "Считать SIM_SEL"() -> (w2432:bool)
            n1620 = local read "SIM_SEL"() -> (w2437:bool)
            n1621 = local read "P3 CH0_warning"() -> (w2433:bool)
            n1622 = Not(x=w2437) -> (.not. x?=w2436:bool)
            n1623 = Select(t=TRUE, s=w2432, f=w2436) -> (s? t:f=w2434:bool)
            n1624 = And(x=w2433, y=w2434) -> (x .and. y?=w2438:bool)
            n1625 = case shown="True" w2438 {
              frame False {
              }
              frame True {
                n1626 = local read "P3 CH0_counter"() -> (w2440:u32)
                n1627 = Increment(x=w2440) -> (x+1=→"P3 CH0_counter":u32)
              }
            }
          }
        }
        n1628 = flat-sequence {
          tunnel: w2323 -> [w2409]
          frame #0 {
            n1629 = case shown="True" w2409 {
              frame False {
              }
              frame True {
                n1630 = Wait (ms)(milliseconds to wait=u32 50) -> ()  [unwired: 1 out]
              }
            }
          }
          frame #1 {
            n1631 = local read "P3 CH1_cur, A"() -> (w2414:dbl)
            n1632 = local read "SIM_SEL"() -> (w2412:bool)
            n1633 = Greater Or Equal?(x=w2414, y="P3 CH1_selcur, A") -> (x >= y?=w2415:bool)
            n1634 = Or(x=w2412, y=w2415) -> (x .or. y?=→"P3 CH1_warning":bool)
          }
          frame #2 {
            n1635 = local read "Считать SIM_SEL"() -> (w2421:bool)
            n1636 = local read "SIM_SEL"() -> (w2420:bool)
            n1637 = local read "P3 CH1_warning"() -> (w2416:bool)
            n1638 = Not(x=w2420) -> (.not. x?=w2419:bool)
            n1639 = Select(t=TRUE, s=w2421, f=w2419) -> (s? t:f=w2417:bool)
            n1640 = And(x=w2416, y=w2417) -> (x .and. y?=w2422:bool)
            n1641 = case shown="True" w2422 {
              frame False {
              }
              frame True {
                n1642 = local read "P3 CH1_counter"() -> (w2424:u32)
                n1643 = Increment(x=w2424) -> (x+1=→"P3 CH1_counter":u32)
              }
            }
          }
        }
        n1644 = flat-sequence {
          tunnel: w2322 -> [w2393]
          frame #0 {
            n1645 = case shown="True" w2393 {
              frame False {
              }
              frame True {
                n1646 = Wait (ms)(milliseconds to wait=u32 50) -> ()  [unwired: 1 out]
              }
            }
          }
          frame #1 {
            n1647 = local read "P4 CH0_cur, A"() -> (w2399:dbl)
            n1648 = local read "SIM_SEL"() -> (w2396:bool)
            n1649 = Greater Or Equal?(x=w2399, y="P4 CH0_selcur, A") -> (x >= y?=w2398:bool)
            n1650 = Or(x=w2396, y=w2398) -> (x .or. y?=→"P4 CH0_warning":bool)
          }
          frame #2 {
            n1651 = local read "Считать SIM_SEL"() -> (w2403:bool)
            n1652 = local read "SIM_SEL"() -> (w2404:bool)
            n1653 = local read "P4 CH0_warning"() -> (w2400:bool)
            n1654 = Not(x=w2404) -> (.not. x?=w2405:bool)
            n1655 = Select(t=TRUE, s=w2403, f=w2405) -> (s? t:f=w2402:bool)
            n1656 = And(x=w2400, y=w2402) -> (x .and. y?=w2401:bool)
            n1657 = case shown="True" w2401 {
              frame False {
              }
              frame True {
                n1658 = local read "P4 CH0_counter"() -> (w2408:u32)
                n1659 = Increment(x=w2408) -> (x+1=→"P4 CH0_counter":u32)
              }
            }
          }
        }
        n1660 = flat-sequence {
          tunnel: w2338 -> [w2473]
          frame #0 {
            n1661 = case shown="True" w2473 {
              frame False {
              }
              frame True {
                n1662 = Wait (ms)(milliseconds to wait=u32 50) -> ()  [unwired: 1 out]
              }
            }
          }
          frame #1 {
            n1663 = local read "P2 CH1_cur, A"() -> (w2477:dbl)
            n1664 = local read "SIM_SEL"() -> (w2475:bool)
            n1665 = Greater Or Equal?(x=w2477, y="P2 CH1_selcur, A") -> (x >= y?=w2478:bool)
            n1666 = Or(x=w2475, y=w2478) -> (x .or. y?=→"P2 CH1_warning":bool)
          }
          frame #2 {
            n1667 = local read "Считать SIM_SEL"() -> (w2486:bool)
            n1668 = local read "SIM_SEL"() -> (w2485:bool)
            n1669 = local read "P2 CH1_warning"() -> (w2480:bool)
            n1670 = Not(x=w2485) -> (.not. x?=w2484:bool)
            n1671 = Select(t=TRUE, s=w2486, f=w2484) -> (s? t:f=w2482:bool)
            n1672 = And(x=w2480, y=w2482) -> (x .and. y?=w2481:bool)
            n1673 = case shown="True" w2481 {
              frame False {
              }
              frame True {
                n1674 = local read "P2 CH1_counter"() -> (w2488:u32)
                n1675 = Increment(x=w2488) -> (x+1=→"P2 CH1_counter":u32)
              }
            }
          }
        }
        n1676 = flat-sequence {
          tunnel: w2326 -> [w2345]
          frame #0 {
            n1677 = case shown="True" w2345 {
              frame False {
              }
              frame True {
                n1678 = Wait (ms)(milliseconds to wait=u32 50) -> ()  [unwired: 1 out]
              }
            }
          }
          frame #1 {
            n1679 = local read "P4 CH2_cur, A"() -> (w2349:dbl)
            n1680 = local read "SIM_SEL"() -> (w2347:bool)
            n1681 = Greater Or Equal?(x=w2349, y="P4 CH2_selcur, A") -> (x >= y?=w2350:bool)
            n1682 = Or(x=w2347, y=w2350) -> (x .or. y?=→"P4 CH2_warning":bool)
          }
          frame #2 {
            n1683 = local read "Считать SIM_SEL"() -> (w2358:bool)
            n1684 = local read "SIM_SEL"() -> (w2357:bool)
            n1685 = local read "P4 CH2_warning"() -> (w2352:bool)
            n1686 = Not(x=w2357) -> (.not. x?=w2356:bool)
            n1687 = Select(t=TRUE, s=w2358, f=w2356) -> (s? t:f=w2354:bool)
            n1688 = And(x=w2352, y=w2354) -> (x .and. y?=w2353:bool)
            n1689 = case shown="True" w2353 {
              frame False {
              }
              frame True {
                n1690 = local read "P4 CH2_counter"() -> (w2360:u32)
                n1691 = Increment(x=w2360) -> (x+1=→"P4 CH2_counter":u32)
              }
            }
          }
        }
        n1692 = local read "P1 CH0"() -> (w2333:bool)
        n1693 = flat-sequence {
          tunnel: w2330 -> [w2457]
          frame #0 {
            n1694 = case shown="True" w2457 {
              frame False {
              }
              frame True {
                n1695 = Wait (ms)(milliseconds to wait=u32 50) -> ()  [unwired: 1 out]
              }
            }
          }
          frame #1 {
            n1696 = local read "P1 CH2_cur, A"() -> (w2461:dbl)
            n1697 = local read "SIM_SEL"() -> (w2459:bool)
            n1698 = Greater Or Equal?(x=w2461, y="P1 CH2_selcur, A") -> (x >= y?=w2462:bool)
            n1699 = Or(x=w2459, y=w2462) -> (x .or. y?=→"P1 CH2_warning":bool)
          }
          frame #2 {
            n1700 = local read "Считать SIM_SEL"() -> (w2470:bool)
            n1701 = local read "SIM_SEL"() -> (w2469:bool)
            n1702 = local read "P1 CH2_warning"() -> (w2464:bool)
            n1703 = Not(x=w2469) -> (.not. x?=w2468:bool)
            n1704 = Select(t=TRUE, s=w2470, f=w2468) -> (s? t:f=w2466:bool)
            n1705 = And(x=w2464, y=w2466) -> (x .and. y?=w2465:bool)
            n1706 = case shown="True" w2465 {
              frame False {
              }
              frame True {
                n1707 = local read "P1 CH2_counter"() -> (w2472:u32)
                n1708 = Increment(x=w2472) -> (x+1=→"P1 CH2_counter":u32)
              }
            }
          }
        }
        n1709 = flat-sequence {
          tunnel: w2324 -> [w2377]
          frame #0 {
            n1710 = case shown="True" w2377 {
              frame False {
              }
              frame True {
                n1711 = Wait (ms)(milliseconds to wait=u32 50) -> ()  [unwired: 1 out]
              }
            }
          }
          frame #1 {
            n1712 = local read "P4 CH1_cur, A"() -> (w2381:dbl)
            n1713 = local read "SIM_SEL"() -> (w2379:bool)
            n1714 = Greater Or Equal?(x=w2381, y="P4 CH1_selcur, A") -> (x >= y?=w2382:bool)
            n1715 = Or(x=w2379, y=w2382) -> (x .or. y?=→"P4 CH1_warning":bool)
          }
          frame #2 {
            n1716 = local read "Считать SIM_SEL"() -> (w2390:bool)
            n1717 = local read "SIM_SEL"() -> (w2389:bool)
            n1718 = local read "P4 CH1_warning"() -> (w2384:bool)
            n1719 = Not(x=w2389) -> (.not. x?=w2388:bool)
            n1720 = Select(t=TRUE, s=w2390, f=w2388) -> (s? t:f=w2386:bool)
            n1721 = And(x=w2384, y=w2386) -> (x .and. y?=w2385:bool)
            n1722 = case shown="True" w2385 {
              frame False {
              }
              frame True {
                n1723 = local read "P4 CH1_counter"() -> (w2392:u32)
                n1724 = Increment(x=w2392) -> (x+1=→"P4 CH1_counter":u32)
              }
            }
          }
        }
        n1725 = local read "P3 CH0"() -> (w2320:bool)
        n1726 = flat-sequence {
          tunnel: w2325 -> [w2361]
          frame #0 {
            n1727 = case shown="True" w2361 {
              frame False {
              }
              frame True {
                n1728 = Wait (ms)(milliseconds to wait=u32 50) -> ()  [unwired: 1 out]
              }
            }
          }
          frame #1 {
            n1729 = local read "P3 CH2_cur, A"() -> (w2365:dbl)
            n1730 = local read "SIM_SEL"() -> (w2363:bool)
            n1731 = Greater Or Equal?(x=w2365, y="P3 CH2_selcur, A") -> (x >= y?=w2366:bool)
            n1732 = Or(x=w2363, y=w2366) -> (x .or. y?=→"P3 CH2_warning":bool)
          }
          frame #2 {
            n1733 = local read "Считать SIM_SEL"() -> (w2374:bool)
            n1734 = local read "SIM_SEL"() -> (w2373:bool)
            n1735 = local read "P3 CH2_warning"() -> (w2368:bool)
            n1736 = Not(x=w2373) -> (.not. x?=w2372:bool)
            n1737 = Select(t=TRUE, s=w2374, f=w2372) -> (s? t:f=w2370:bool)
            n1738 = And(x=w2368, y=w2370) -> (x .and. y?=w2369:bool)
            n1739 = case shown="True" w2369 {
              frame False {
              }
              frame True {
                n1740 = local read "P3 CH2_counter"() -> (w2376:u32)
                n1741 = Increment(x=w2376) -> (x+1=→"P3 CH2_counter":u32)
              }
            }
          }
        }
        n1742 = Greater?(x=w2335, y=w2341) -> (0:w2340:bool)
        n1743 = Greater?(x=w2333, y=w2344) -> (0:w2343:bool)
        n1744 = Greater?(x=w2327, y=w2328) -> (0:w2329:bool)
        n1745 = Greater?(x=w2317, y=w2318) -> (0:w2322:bool)
        n1746 = Greater?(x=w2334, y=w2342) -> (0:w2339:bool)
        n1747 = Greater?(x=w2336, y=w2337) -> (0:w2338:bool)
        n1748 = Greater?(x=w2320, y=w2319) -> (0:w2321:bool)
        n1749 = Greater?(x=w2310, y=w2309) -> (0:w2326:bool)
        n1750 = Greater?(x=w2332, y=w2331) -> (0:w2330:bool)
        n1751 = Greater?(x=w2315, y=w2316) -> (0:w2323:bool)
        n1752 = Greater?(x=w2313, y=w2314) -> (0:w2324:bool)
        n1753 = Greater?(x=w2311, y=w2312) -> (0:w2325:bool)
      }
      frame #1 {
        w2634 = "\t"
        w2651 = "\t"
        w2648 = 0
        w2647 = 6
        w2643 = 6
        w2617 = "\t"
        w2633 = "\t"
        w2631 = 0
        w2630 = 6
        w2625 = 6
        w2615 = "\t"
        w2608 = "\t"
        w2606 = "\t"
        w2604 = "\t"
        w2614 = "\t"
        w2613 = "\t"
        w2612 = "\t"
        w2611 = "\t"
        w2573 = 0
        w2574 = 6
        w2578 = 6
        w2568 = 0
        w2567 = 6
        w2563 = 6
        w2554 = 0
        w2555 = 6
        w2560 = 6
        w2551 = 0
        w2550 = 6
        w2545 = 6
        w2673 = "\t"
        w2656 = "\t"
        w2659 = 0
        w2660 = 6
        w2664 = 6
        w2690 = "\t"
        w2674 = "\t"
        w2676 = 0
        w2677 = 6
        w2682 = 6
        w2693 = "\t"
        w2703 = "\t"
        w2705 = "\t"
        w2707 = "\t"
        w2694 = "\t"
        w2695 = "\t"
        w2696 = "\t"
        w2697 = "\t"
        w2738 = 0
        w2737 = 6
        w2733 = 6
        w2743 = 0
        w2744 = 6
        w2748 = 6
        w2757 = 0
        w2756 = 6
        w2751 = 6
        w2760 = 0
        w2761 = 6
        w2767 = 6
        # "Запись логов"
        n1754 = local read "P3 CH2_cur, A"() -> (w2629:dbl)
        n1755 = local read "P1 CH2_cur, A"() -> (w2678:dbl)
        n1756 = local read "P3 CH1_cur, A"() -> (w2556:dbl)
        n1757 = local read "P3 CH2, V"() -> (w2627:dbl)
        n1758 = local read "P3 CH2_counter"() -> (w2632:u32)
        n1759 = local read "P3 CH2_warning"() -> (w2628:bool)
        n1760 = local read "P4 CH1, V"() -> (w2571:dbl)
        n1761 = local read "P4 CH1_cur, A"() -> (w2575:dbl)
        n1762 = local read "P4 CH1_counter"() -> (w2572:u32)
        n1763 = local read "P4 CH1_warning"() -> (w2576:bool)
        n1764 = local read "P4 CH2, V"() -> (w2650:dbl)
        n1765 = local read "P4 CH2_cur, A"() -> (w2646:dbl)
        n1766 = local read "P4 CH2_counter"() -> (w2649:u32)
        n1767 = local read "P4 CH2_warning"() -> (w2645:bool)
        n1768 = local read "P1 CH1_cur, A"() -> (w2755:dbl)
        n1769 = local read "P1 CH2, V"() -> (w2680:dbl)
        n1770 = local read "P1 CH2_counter"() -> (w2675:u32)
        n1771 = local read "P1 CH2_warning"() -> (w2679:bool)
        n1772 = local read "P2 CH1, V"() -> (w2740:dbl)
        n1773 = local read "P2 CH1_cur, A"() -> (w2736:dbl)
        n1774 = local read "P2 CH1_counter"() -> (w2739:u32)
        n1775 = local read "P2 CH1_warning"() -> (w2735:bool)
        n1776 = local read "P2 CH2, V"() -> (w2657:dbl)
        n1777 = local read "P2 CH2_cur, A"() -> (w2661:dbl)
        n1778 = local read "P2 CH2_counter"() -> (w2658:u32)
        n1779 = local read "P2 CH2_warning"() -> (w2662:bool)
        n1780 = local read "P3 CH0, V"() -> (w2547:dbl)
        n1781 = local read "P3 CH0_cur, A"() -> (w2549:dbl)
        n1782 = local read "P3 CH0_counter"() -> (w2552:u32)
        n1783 = local read "P3 CH0_warning"() -> (w2548:bool)
        n1784 = local read "P3 CH1, V"() -> (w2558:dbl)
        n1785 = local read "P3 CH1_counter"() -> (w2553:u32)
        n1786 = local read "P3 CH1_warning"() -> (w2557:bool)
        n1787 = local read "P4 CH0, V"() -> (w2570:dbl)
        n1788 = local read "P4 CH0_cur, A"() -> (w2566:dbl)
        n1789 = local read "P4 CH0_counter"() -> (w2569:u32)
        n1790 = local read "P4 CH0_warning"() -> (w2565:bool)
        n1791 = local read "P1 CH0, V"() -> (w2765:dbl)
        n1792 = local read "P1 CH0_cur, A"() -> (w2762:dbl)
        n1793 = local read "P1 CH0_counter"() -> (w2759:u32)
        n1794 = local read "P1 CH0_warning"() -> (w2763:bool)
        n1795 = local read "P1 CH1, V"() -> (w2753:dbl)
        n1796 = local read "P1 CH1_counter"() -> (w2758:u32)
        n1797 = local read "P1 CH1_warning"() -> (w2754:bool)
        n1798 = local read "P2 CH0, V"() -> (w2741:dbl)
        n1799 = local read "P2 CH0_cur, A"() -> (w2745:dbl)
        n1800 = local read "P2 CH0_counter"() -> (w2742:u32)
        n1801 = local read "P2 CH0_warning"() -> (w2746:bool)
        n1802 = Number To Fractional String(number=w2627, width (-)=w2625, precision (6)=w2625) -> (F-format string=w2623:string)  [unwired: 1 in]
        n1803 = Number To Fractional String(number=w2629, width (-)=w2630, precision (6)=w2630) -> (F-format string=w2622:string)  [unwired: 1 in]
        n1804 = Number To Fractional String(number=w2632, width (-)=w2631, precision (6)=w2631) -> (F-format string=w2621:string)  [unwired: 1 in]
        n1805 = Number To Fractional String(number=w2571, width (-)=w2578, precision (6)=w2578) -> (F-format string=w2592:string)  [unwired: 1 in]
        n1806 = Number To Fractional String(number=w2575, width (-)=w2574, precision (6)=w2574) -> (F-format string=w2593:string)  [unwired: 1 in]
        n1807 = Number To Fractional String(number=w2572, width (-)=w2573, precision (6)=w2573) -> (F-format string=w2594:string)  [unwired: 1 in]
        n1808 = Number To Fractional String(number=w2650, width (-)=w2643, precision (6)=w2643) -> (F-format string=w2641:string)  [unwired: 1 in]
        n1809 = Number To Fractional String(number=w2646, width (-)=w2647, precision (6)=w2647) -> (F-format string=w2640:string)  [unwired: 1 in]
        n1810 = Number To Fractional String(number=w2649, width (-)=w2648, precision (6)=w2648) -> (F-format string=w2639:string)  [unwired: 1 in]
        n1811 = Number To Fractional String(number=w2680, width (-)=w2682, precision (6)=w2682) -> (F-format string=w2684:string)  [unwired: 1 in]
        n1812 = Number To Fractional String(number=w2678, width (-)=w2677, precision (6)=w2677) -> (F-format string=w2685:string)  [unwired: 1 in]
        n1813 = Number To Fractional String(number=w2675, width (-)=w2676, precision (6)=w2676) -> (F-format string=w2686:string)  [unwired: 1 in]
        n1814 = Number To Fractional String(number=w2740, width (-)=w2733, precision (6)=w2733) -> (F-format string=w2719:string)  [unwired: 1 in]
        n1815 = Number To Fractional String(number=w2736, width (-)=w2737, precision (6)=w2737) -> (F-format string=w2718:string)  [unwired: 1 in]
        n1816 = Number To Fractional String(number=w2739, width (-)=w2738, precision (6)=w2738) -> (F-format string=w2717:string)  [unwired: 1 in]
        n1817 = Number To Fractional String(number=w2657, width (-)=w2664, precision (6)=w2664) -> (F-format string=w2666:string)  [unwired: 1 in]
        n1818 = Number To Fractional String(number=w2661, width (-)=w2660, precision (6)=w2660) -> (F-format string=w2667:string)  [unwired: 1 in]
        n1819 = Number To Fractional String(number=w2658, width (-)=w2659, precision (6)=w2659) -> (F-format string=w2668:string)  [unwired: 1 in]
        n1820 = Number To Fractional String(number=w2547, width (-)=w2545, precision (6)=w2545) -> (F-format string=w2580:string)  [unwired: 1 in]
        n1821 = Number To Fractional String(number=w2549, width (-)=w2550, precision (6)=w2550) -> (F-format string=w2581:string)  [unwired: 1 in]
        n1822 = Number To Fractional String(number=w2552, width (-)=w2551, precision (6)=w2551) -> (F-format string=w2582:string)  [unwired: 1 in]
        n1823 = Number To Fractional String(number=w2558, width (-)=w2560, precision (6)=w2560) -> (F-format string=w2584:string)  [unwired: 1 in]
        n1824 = Number To Fractional String(number=w2556, width (-)=w2555, precision (6)=w2555) -> (F-format string=w2585:string)  [unwired: 1 in]
        n1825 = Number To Fractional String(number=w2553, width (-)=w2554, precision (6)=w2554) -> (F-format string=w2586:string)  [unwired: 1 in]
        n1826 = Number To Fractional String(number=w2570, width (-)=w2563, precision (6)=w2563) -> (F-format string=w2588:string)  [unwired: 1 in]
        n1827 = Number To Fractional String(number=w2566, width (-)=w2567, precision (6)=w2567) -> (F-format string=w2589:string)  [unwired: 1 in]
        n1828 = Number To Fractional String(number=w2569, width (-)=w2568, precision (6)=w2568) -> (F-format string=w2590:string)  [unwired: 1 in]
        n1829 = Number To Fractional String(number=w2765, width (-)=w2767, precision (6)=w2767) -> (F-format string=w2731:string)  [unwired: 1 in]
        n1830 = Number To Fractional String(number=w2762, width (-)=w2761, precision (6)=w2761) -> (F-format string=w2730:string)  [unwired: 1 in]
        n1831 = Number To Fractional String(number=w2759, width (-)=w2760, precision (6)=w2760) -> (F-format string=w2729:string)  [unwired: 1 in]
        n1832 = Number To Fractional String(number=w2753, width (-)=w2751, precision (6)=w2751) -> (F-format string=w2727:string)  [unwired: 1 in]
        n1833 = Number To Fractional String(number=w2755, width (-)=w2756, precision (6)=w2756) -> (F-format string=w2726:string)  [unwired: 1 in]
        n1834 = Number To Fractional String(number=w2758, width (-)=w2757, precision (6)=w2757) -> (F-format string=w2725:string)  [unwired: 1 in]
        n1835 = Number To Fractional String(number=w2741, width (-)=w2748, precision (6)=w2748) -> (F-format string=w2723:string)  [unwired: 1 in]
        n1836 = Number To Fractional String(number=w2745, width (-)=w2744, precision (6)=w2744) -> (F-format string=w2722:string)  [unwired: 1 in]
        n1837 = Number To Fractional String(number=w2742, width (-)=w2743, precision (6)=w2743) -> (F-format string=w2721:string)  [unwired: 1 in]
        n1838 = Select(t="!!!3_2", s=w2628, f="") -> (s? t:f=w2620:string)
        n1839 = Select(t="!!!4_1", s=w2576, f="") -> (s? t:f=w2595:string)
        n1840 = Select(t="!!!4_2", s=w2645, f="") -> (s? t:f=w2638:string)
        n1841 = Select(t="!!!1_2", s=w2679, f="") -> (s? t:f=w2687:string)
        n1842 = Select(t="!!!2_1", s=w2735, f="") -> (s? t:f=w2716:string)
        n1843 = Select(t="!!!2_2", s=w2662, f="") -> (s? t:f=w2669:string)
        n1844 = Select(t="!!!3_0", s=w2548, f="") -> (s? t:f=w2583:string)
        n1845 = Select(t="!!!3_1", s=w2557, f="") -> (s? t:f=w2587:string)
        n1846 = Select(t="!!!4_0", s=w2565, f="") -> (s? t:f=w2591:string)
        n1847 = Select(t="!!!1_0", s=w2763, f="") -> (s? t:f=w2728:string)
        n1848 = Select(t="!!!1_1", s=w2754, f="") -> (s? t:f=w2724:string)
        n1849 = Select(t="!!!2_0", s=w2746, f="") -> (s? t:f=w2720:string)
        n1850 = local read "P3 CH2 Used"() -> (w2618:bool)
        n1851 = local read "P1 CH2 Used"() -> (w2689:bool)
        n1852 = local read "P3 CH0 Used"() -> (w2599:bool)
        n1853 = local read "P3 CH1 Used"() -> (w2600:bool)
        n1854 = local read "P4 CH0 Used"() -> (w2601:bool)
        n1855 = local read "P4 CH1 Used"() -> (w2602:bool)
        n1856 = local read "P4 CH2 Used"() -> (w2637:bool)
        n1857 = local read "P1 CH0 Used"() -> (w2712:bool)
        n1858 = local read "P1 CH1 Used"() -> (w2711:bool)
        n1859 = local read "P2 CH0 Used"() -> (w2710:bool)
        n1860 = local read "P2 CH1 Used"() -> (w2709:bool)
        n1861 = local read "P2 CH2 Used"() -> (w2670:bool)
        n1862 = Concatenate Strings(w2633, w2623, w2633, w2622, w2633, w2621, w2633, w2620) -> (w2619:string)
        n1863 = Concatenate Strings(w2674, w2684, w2674, w2685, w2674, w2686, w2674, w2687) -> (w2688:string)
        n1864 = Concatenate Strings(w2611, w2580, w2611, w2581, w2611, w2582, w2611, w2583) -> (w2597:string)
        n1865 = Concatenate Strings(w2612, w2584, w2612, w2585, w2612, w2586, w2612, w2587) -> (w2596:string)
        n1866 = Concatenate Strings(w2613, w2588, w2613, w2589, w2613, w2590, w2613, w2591) -> (w2598:string)
        n1867 = Concatenate Strings(w2614, w2592, w2614, w2593, w2614, w2594, w2614, w2595) -> (w2603:string)
        n1868 = Concatenate Strings(w2651, w2641, w2651, w2640, w2651, w2639, w2651, w2638) -> (w2636:string)
        n1869 = Concatenate Strings(w2697, w2731, w2697, w2730, w2697, w2729, w2697, w2728) -> (w2714:string)
        n1870 = Concatenate Strings(w2696, w2727, w2696, w2726, w2696, w2725, w2696, w2724) -> (w2715:string)
        n1871 = Concatenate Strings(w2695, w2723, w2695, w2722, w2695, w2721, w2695, w2720) -> (w2713:string)
        n1872 = Concatenate Strings(w2694, w2719, w2694, w2718, w2694, w2717, w2694, w2716) -> (w2708:string)
        n1873 = Concatenate Strings(w2656, w2666, w2656, w2667, w2656, w2668, w2656, w2669) -> (w2671:string)
        n1874 = Concatenate Strings(w2617, w2617, w2617, w2617) -> (w2616:string)
        n1875 = Concatenate Strings(w2690, w2690, w2690, w2690) -> (w2691:string)
        n1876 = Concatenate Strings(w2604, w2604, w2604, w2604) -> (w2605:string)
        n1877 = Concatenate Strings(w2606, w2606, w2606, w2606) -> (w2607:string)
        n1878 = Concatenate Strings(w2608, w2608, w2608, w2608) -> (w2609:string)
        n1879 = Concatenate Strings(w2615, w2615, w2615, w2615) -> (w2610:string)
        n1880 = Concatenate Strings(w2634, w2634, w2634, w2634) -> (w2635:string)
        n1881 = Concatenate Strings(w2707, w2707, w2707, w2707) -> (w2706:string)
        n1882 = Concatenate Strings(w2705, w2705, w2705, w2705) -> (w2704:string)
        n1883 = Concatenate Strings(w2703, w2703, w2703, w2703) -> (w2702:string)
        n1884 = Concatenate Strings(w2693, w2693, w2693, w2693) -> (w2701:string)
        n1885 = Concatenate Strings(w2673, w2673, w2673, w2673) -> (w2672:string)
        n1886 = Select(t=w2619, s=w2618, f=w2616) -> (s? t:f=w2541:string)
        n1887 = Select(t=w2688, s=w2689, f=w2691) -> (s? t:f=w2655:string)
        n1888 = Select(t=w2597, s=w2599, f=w2605) -> (s? t:f=w2543:string)
        n1889 = Select(t=w2596, s=w2600, f=w2607) -> (s? t:f=w2542:string)
        n1890 = Select(t=w2598, s=w2601, f=w2609) -> (s? t:f=w2540:string)
        n1891 = Select(t=w2603, s=w2602, f=w2610) -> (s? t:f=w2539:string)
        n1892 = Select(t=w2636, s=w2637, f=w2635) -> (s? t:f=w2538:string)
        n1893 = Select(t=w2714, s=w2712, f=w2706) -> (s? t:f=w2700:string)
        n1894 = Select(t=w2715, s=w2711, f=w2704) -> (s? t:f=w2699:string)
        n1895 = Select(t=w2713, s=w2710, f=w2702) -> (s? t:f=w2654:string)
        n1896 = Select(t=w2708, s=w2709, f=w2701) -> (s? t:f=w2653:string)
        n1897 = Select(t=w2671, s=w2670, f=w2672) -> (s? t:f=w2652:string)
        n1898 = Get Date/Time In Seconds() -> (seconds since 1Jan1904=w2770:timestamp)
        n1899 = Format Date/Time String(time format string (%c)="%H:%M:%S:%3u", seconds (now)=w2770) -> (date/time string=w2768:string)  [unwired: 1 in]
        n1900 = local read "SEL output file refnum"() -> (w2692:refnum<file>)
        n1901 = Concatenate Strings(w2768, w2700, w2699, w2655, w2654, w2653, w2652, w2543, w2542, w2541, w2540, w2539, w2538, "\r\n") -> (w2698:string)
        n1902 = Format Into String(initial string=w2692, w2698) -> (resulting string=w2764:refnum<file>)  [unwired: 2 in, 1 out]
      }
      frame #2 {
        n1903 = local read "P1 CH0_warning"() -> (w2806:bool)
        "SEL" <- w2806
        n1904 = local read "P1 CH1_warning"() -> (w2798:bool)
        n1905 = local read "P2 CH0_warning"() -> (w2796:bool)
        n1906 = local read "P2 CH1_warning"() -> (w2797:bool)
        n1907 = local read "P1 CH2_warning"() -> (w2795:bool)
        n1908 = local read "P2 CH2_warning"() -> (w2794:bool)
        n1909 = local read "P3 CH0_warning"() -> (w2772:bool)
        n1910 = local read "P3 CH1_warning"() -> (w2785:bool)
        n1911 = local read "P4 CH0_warning"() -> (w2787:bool)
        n1912 = local read "P4 CH1_warning"() -> (w2786:bool)
        n1913 = local read "P3 CH2_warning"() -> (w2788:bool)
        n1914 = local read "P4 CH2_warning"() -> (w2789:bool)
        n1915 = local write "SEL"(w2796) -> ()
        n1916 = local write "SEL"(w2798) -> ()
        n1917 = local write "SEL"(w2787) -> ()
        n1918 = local write "SEL"(w2797) -> ()
        n1919 = local write "SEL"(w2795) -> ()
        n1920 = local write "SEL"(w2794) -> ()
        n1921 = local write "SEL"(w2785) -> ()
        n1922 = local write "SEL"(w2772) -> ()
        n1923 = local write "SEL"(w2786) -> ()
        n1924 = local write "SEL"(w2788) -> ()
        n1925 = local write "SEL"(w2789) -> ()
        n1926 = case shown="True" w2806 {
          tunnel: [w2874 w2875] -> w2807
          tunnel: w2799 -> [w2874 _]
          frame False {
          }
          frame True {
            n1927 = flat-sequence {
              tunnel: [FALSE] -> w2875
              frame #0 {
                n1928 = local write "P1 CH0"(FALSE ("Power")) -> ()
              }
              frame #1 {
                n1929 = Wait (ms)(milliseconds to wait=u32 100 ("Wait_parry, ms")) -> ()  [unwired: 1 out]
              }
              frame #2 {
                n1930 = local write "P1 CH0"(TRUE ("Power")) -> ()
              }
            }
          }
        }
        n1931 = case shown="True" w2798 {
          tunnel: [w2868 w2869] -> w2801
          tunnel: w2800 -> [w2868 _]
          frame False {
          }
          frame True {
            n1932 = flat-sequence {
              tunnel: [FALSE] -> w2869
              frame #0 {
                n1933 = local write "P1 CH1"(FALSE ("Power")) -> ()
              }
              frame #1 {
                n1934 = Wait (ms)(milliseconds to wait=u32 100 ("Wait_parry, ms")) -> ()  [unwired: 1 out]
              }
              frame #2 {
                n1935 = local write "P1 CH1"(TRUE ("Power")) -> ()
              }
            }
          }
        }
        n1936 = case shown="True" w2796 {
          tunnel: [w2862 w2863] -> w2803
          tunnel: w2802 -> [w2862 _]
          frame False {
          }
          frame True {
            n1937 = flat-sequence {
              tunnel: [FALSE] -> w2863
              frame #0 {
                n1938 = local write "P2 CH0"(FALSE ("Power")) -> ()
              }
              frame #1 {
                n1939 = Wait (ms)(milliseconds to wait=u32 100 ("Wait_parry, ms")) -> ()  [unwired: 1 out]
              }
              frame #2 {
                n1940 = local write "P2 CH0"(TRUE ("Power")) -> ()
              }
            }
          }
        }
        n1941 = case shown="True" w2797 {
          tunnel: [w2856 w2857] -> w2804
          tunnel: w2805 -> [w2856 _]
          frame False {
          }
          frame True {
            n1942 = flat-sequence {
              tunnel: [FALSE] -> w2857
              frame #0 {
                n1943 = local write "P2 CH1"(FALSE ("Power")) -> ()
              }
              frame #1 {
                n1944 = Wait (ms)(milliseconds to wait=u32 100 ("Wait_parry, ms")) -> ()  [unwired: 1 out]
              }
              frame #2 {
                n1945 = local write "P2 CH1"(TRUE ("Power")) -> ()
              }
            }
          }
        }
        n1946 = case shown="True" w2795 {
          tunnel: [w2850 w2851] -> w2791
          tunnel: w2792 -> [w2850 _]
          frame False {
          }
          frame True {
            n1947 = flat-sequence {
              tunnel: [FALSE] -> w2851
              frame #0 {
                n1948 = local write "P1 CH2"(FALSE ("Power")) -> ()
              }
              frame #1 {
                n1949 = Wait (ms)(milliseconds to wait=u32 100 ("Wait_parry, ms")) -> ()  [unwired: 1 out]
              }
              frame #2 {
                n1950 = local write "P1 CH2"(TRUE ("Power")) -> ()
              }
            }
          }
        }
        n1951 = case shown="True" w2794 {
          tunnel: [w2844 w2845] -> w2790
          tunnel: w2793 -> [w2844 _]
          frame False {
          }
          frame True {
            n1952 = flat-sequence {
              tunnel: [FALSE] -> w2845
              frame #0 {
                n1953 = local write "P2 CH2"(FALSE ("Power")) -> ()
              }
              frame #1 {
                n1954 = Wait (ms)(milliseconds to wait=u32 100 ("Wait_parry, ms")) -> ()  [unwired: 1 out]
              }
              frame #2 {
                n1955 = local write "P2 CH2"(TRUE ("Power")) -> ()
              }
            }
          }
        }
        n1956 = case shown="True" w2772 {
          tunnel: [w2838 w2839] -> w2778
          tunnel: w2784 -> [w2838 _]
          frame False {
          }
          frame True {
            n1957 = flat-sequence {
              tunnel: [FALSE] -> w2839
              frame #0 {
                n1958 = local write "P3 CH0"(FALSE ("Power")) -> ()
              }
              frame #1 {
                n1959 = Wait (ms)(milliseconds to wait=u32 100 ("Wait_parry, ms")) -> ()  [unwired: 1 out]
              }
              frame #2 {
                n1960 = local write "P3 CH0"(TRUE ("Power")) -> ()
              }
            }
          }
        }
        n1961 = case shown="True" w2785 {
          tunnel: [w2832 w2833] -> w2777
          tunnel: w2783 -> [w2832 _]
          frame False {
          }
          frame True {
            n1962 = flat-sequence {
              tunnel: [FALSE] -> w2833
              frame #0 {
                n1963 = local write "P3 CH1"(FALSE ("Power")) -> ()
              }
              frame #1 {
                n1964 = Wait (ms)(milliseconds to wait=u32 100 ("Wait_parry, ms")) -> ()  [unwired: 1 out]
              }
              frame #2 {
                n1965 = local write "P3 CH1"(TRUE ("Power")) -> ()
              }
            }
          }
        }
        n1966 = case shown="True" w2787 {
          tunnel: [w2826 w2827] -> w2776
          tunnel: w2781 -> [w2826 _]
          frame False {
          }
          frame True {
            n1967 = flat-sequence {
              tunnel: [FALSE] -> w2827
              frame #0 {
                n1968 = local write "P4 CH0"(FALSE ("Power")) -> ()
              }
              frame #1 {
                n1969 = Wait (ms)(milliseconds to wait=u32 100 ("Wait_parry, ms")) -> ()  [unwired: 1 out]
              }
              frame #2 {
                n1970 = local write "P4 CH0"(TRUE ("Power")) -> ()
              }
            }
          }
        }
        n1971 = case shown="True" w2786 {
          tunnel: [w2820 w2821] -> w2775
          tunnel: w2782 -> [w2820 _]
          frame False {
          }
          frame True {
            n1972 = flat-sequence {
              tunnel: [FALSE] -> w2821
              frame #0 {
                n1973 = local write "P4 CH1"(FALSE ("Power")) -> ()
              }
              frame #1 {
                n1974 = Wait (ms)(milliseconds to wait=u32 100 ("Wait_parry, ms")) -> ()  [unwired: 1 out]
              }
              frame #2 {
                n1975 = local write "P4 CH1"(TRUE ("Power")) -> ()
              }
            }
          }
        }
        n1976 = case shown="True" w2788 {
          tunnel: [w2814 w2815] -> w2774
          tunnel: w2780 -> [w2814 _]
          frame False {
          }
          frame True {
            n1977 = flat-sequence {
              tunnel: [FALSE] -> w2815
              frame #0 {
                n1978 = local write "P3 CH2"(FALSE ("Power")) -> ()
              }
              frame #1 {
                n1979 = Wait (ms)(milliseconds to wait=u32 100 ("Wait_parry, ms")) -> ()  [unwired: 1 out]
              }
              frame #2 {
                n1980 = local write "P3 CH2"(TRUE ("Power")) -> ()
              }
            }
          }
        }
        n1981 = case shown="True" w2789 {
          tunnel: [w2808 w2809] -> w2773
          tunnel: w2779 -> [w2808 _]
          frame False {
          }
          frame True {
            n1982 = flat-sequence {
              tunnel: [FALSE] -> w2809
              frame #0 {
                n1983 = local write "P4 CH2"(FALSE ("Power")) -> ()
              }
              frame #1 {
                n1984 = Wait (ms)(milliseconds to wait=u32 100 ("Wait_parry, ms")) -> ()  [unwired: 1 out]
              }
              frame #2 {
                n1985 = local write "P4 CH2"(TRUE ("Power")) -> ()
              }
            }
          }
        }
      }
      frame #3 {
        n1986 = local read "System Stop"() -> (w2880:bool)
      }
    }
  }
  n1987 = while {
    tunnel: w1 -> [_]
    stop <- w2883 stop-if-true
    n1988 = Wait (ms)(milliseconds to wait=u32 100) -> ()  [unwired: 1 out]
    n1989 = case shown="False" "HMI Stop" {
      selector: "HMI Stop" -> [w2884 _]
      tunnel: [w2884 w2885] -> w2883
      frame False {
      }
      frame True {
        n1990 = local read "Glass Meas Cycle Running"() -> (w2890:bool)
        n1991 = local read "Meas Running"() -> (w2888:bool)
        n1992 = Not(x=w2890) -> (.not. x?=w2887:bool)
        n1993 = Not(x=w2888) -> (.not. x?=w2889:bool)
        n1994 = Compound Arithmetic op=AND(w2887, w2889) -> (w2886:bool)
        n1995 = case shown="False" w2886 {
          selector: w2886 -> [w2891 w2896]
          tunnel: [w2891 w2896] -> w2885
          frame False {
            n1996 = One Button Dialog(message="Please, wait for the measurement to complete.", button name ("OK")="Oh, shit, I'm sorry.") -> (true=w2895:bool)
            n1997 = Not(x=w2895) -> (.not. x?=w2894:bool)
            n1998 = local write "HMI Stop"(w2894) -> ()
          }
          frame True {
            n1999 = local write "System Stop"(w2896) -> ()
          }
        }
      }
    }
  }
  n2000 = flat-sequence {
    tunnel: w52 -> [w2910]
    tunnel: w51 -> [w2909]
    tunnel: w27 -> [w2908]
    tunnel: w23 -> [_]
    tunnel: w49 -> [w2907]
    tunnel: w26 -> [w2906]
    tunnel: w20 -> [w2905]
    tunnel: w19 -> [w2904]
    tunnel: w18 -> [w2903]
    tunnel: w17 -> [w2902]
    tunnel: w11 -> [w2901]
    tunnel: w10 -> [w2900]
    tunnel: w9 -> [w2899]
    tunnel: w8 -> [w2898]
    frame #0 {
      w2897 = T7."Enabled" ("Disabled")
      # "STOP"
      n2001 = case shown="True" w2905 {
        tunnel: w2909 -> [_ w2927]
        tunnel: w2907 -> [_ w2926]
        frame False {
        }
        frame True {
          n2002 = call <instrlib>:"niDCPower Close.vi"("error in (no error)"=w2926, "instrument handle"=w2927) -> ("error out"=w2925:errorcluster)  [unwired: 9 in]
          n2003 = call <vilib>:"Simple Error Handler.vi"("error in (no error)"=w2925) -> ("error out"=w2924:errorcluster)  [unwired: 1 in, 7 out]
          n2004 = local write "DC Power 1 error out"(w2924) -> ()
        }
      }
      n2005 = case shown="True" w2901 {
        tunnel: w2903 -> [_ w2919]
        tunnel: w2902 -> [_ w2918]
        frame False {
        }
        frame True {
          n2006 = call <instrlib>:"niDCPower Close.vi"("error in (no error)"=w2918, "instrument handle"=w2919) -> ("error out"=w2917:errorcluster)  [unwired: 9 in]
          n2007 = call <vilib>:"Simple Error Handler.vi"("error in (no error)"=w2917) -> ("error out"=w2916:errorcluster)  [unwired: 1 in, 7 out]
          n2008 = local write "DC Power 3 error out"(w2916) -> ()
        }
      }
      n2009 = Close File(refnum=w2910) -> ()  [unwired: 1 in, 2 out]
      n2010 = case shown="True" w2904 {
        tunnel: w2908 -> [_ w2923]
        tunnel: w2906 -> [_ w2922]
        frame False {
        }
        frame True {
          n2011 = call <instrlib>:"niDCPower Close.vi"("error in (no error)"=w2922, "instrument handle"=w2923) -> ("error out"=w2921:errorcluster)  [unwired: 9 in]
          n2012 = call <vilib>:"Simple Error Handler.vi"("error in (no error)"=w2921) -> ("error out"=w2920:errorcluster)  [unwired: 1 in, 7 out]
          n2013 = local write "DC Power 2 error out"(w2920) -> ()
        }
      }
      n2014 = case shown="True" w2898 {
        tunnel: w2900 -> [_ w2915]
        tunnel: w2899 -> [_ w2914]
        frame False {
        }
        frame True {
          n2015 = call <instrlib>:"niDCPower Close.vi"("error in (no error)"=w2914, "instrument handle"=w2915) -> ("error out"=w2913:errorcluster)  [unwired: 9 in]
          n2016 = call <vilib>:"Simple Error Handler.vi"("error in (no error)"=w2913) -> ("error out"=w2912:errorcluster)  [unwired: 1 in, 7 out]
          n2017 = local write "DC Power 4 error out"(w2912) -> ()
        }
      }
      n2018 = property on="NI Scope Tab" class="TabCtl (strict)"("DisabledEnum"=w2897) -> ()  [unwired: 2 in, 2 out]
      n2019 = property on="NI DMM 1 Tab" class="TabCtl (strict)"("DisabledEnum"=w2897) -> ()  [unwired: 2 in, 2 out]
      n2020 = property on="NI DMM 2 Tab" class="TabCtl (strict)"("DisabledEnum"=w2897) -> ()  [unwired: 2 in, 2 out]
      n2021 = property on="NI DMM 3 Tab" class="TabCtl (strict)"("DisabledEnum"=w2897) -> ()  [unwired: 2 in, 2 out]
      n2022 = property on="Tab DC Power 1" class="TabCtl (strict)"("DisabledEnum"=w2897) -> ()  [unwired: 2 in, 2 out]
      n2023 = property on="Tab DC Power 2" class="TabCtl (strict)"("DisabledEnum"=w2897) -> ()  [unwired: 2 in, 2 out]
      n2024 = property on="Tab DC Power 3" class="TabCtl (strict)"("DisabledEnum"=w2897) -> ()  [unwired: 2 in, 2 out]
      n2025 = property on="Tab DC Power 4" class="TabCtl (strict)"("DisabledEnum"=w2897) -> ()  [unwired: 2 in, 2 out]
      n2026 = property on="Ophir 1 Tab" class="TabCtl (strict)"("DisabledEnum"=w2897) -> ()  [unwired: 2 in, 2 out]
      n2027 = property on="Ophir 2 Tab" class="TabCtl (strict)"("DisabledEnum"=w2897) -> ()  [unwired: 2 in, 2 out]
      n2028 = property on="Stepper Motor Control" class="TabCtl (strict)"("DisabledEnum"=w2897) -> ()  [unwired: 2 in, 2 out]
      n2029 = property on="Table Tab" class="TabCtl (strict)"("DisabledEnum"=w2897) -> ()  [unwired: 2 in, 2 out]
      n2030 = Wait (ms)(milliseconds to wait=u32 1) -> ()  [unwired: 1 out]
    }
  }
  n2031 = case shown="True" w37 {
    tunnel: w2 -> [_ w2929]
    frame False {
    }
    frame True {
      n2032 = local read "Ophir 2 dup Visa Session"() -> (w2931:refnum<visa-resource-name>)
      n2033 = local read "Ophir 2 error out"() -> (w2930:errorcluster)
      n2034 = while {
        tunnel: [w2942] -> w2933
        tunnel: [w2936] -> w2932
        tunnel: w2931 -> [w2940]
        tunnel: w2930 -> [w2939]
        tunnel: w2929 -> [_]
        shift-right: [w2937] -> _
        shift-left: 0.0 -> [w2938]
        stop <- w2941 stop-if-true
        n2035 = Wait (ms)(milliseconds to wait="Ophir 2 Wait") -> ()  [unwired: 1 out]
        n2036 = stacked-sequence {
          tunnel: [w2958] -> w2942
          tunnel: [w2943] -> w2941
          tunnel: w2940 -> [w2944]
          tunnel: w2939 -> [w2953]
          tunnel: w2938 -> [w2947]
          tunnel: [w2945] -> w2937
          tunnel: [w2944] -> w2936
          frame #0 {
            n2037 = Fract/Exp String To Number(string="Ophir 2 units") -> (number=w2946:dbl)  [unwired: 3 in, 1 out]
            n2038 = call "Ophir SendPower.vi"("Visa Session"=w2944, "error in (no error)"=w2953) -> ("Value Number"=w2955:dbl, "Value String"=w2956:string, "error out"=w2958:errorcluster)  [unwired: 1 out]
            "Ophir 2 Real Optical Power" <- w2955
            n2039 = call "Ophir Over.vi"("Value String"=w2956) -> ("Overrange"=→"Ophir 2 Over Range":bool)
            n2040 = Multiply(x=w2955, y=w2946) -> (x*y=w2951:dbl)
            "Ophir 2 Char" <- w2951
            "Ophir 2 Optical Power" <- w2951
            n2041 = Greater Or Equal?(x=w2951, y=w2947) -> (x >= y?=w2952:bool)
            n2042 = Select(t=0.0, s="Ophir 2 Clear", f=w2947) -> (s? t:f=w2950:dbl)
            n2043 = Select(t=w2951, s=w2952, f=w2950) -> (s? t:f=w2945:dbl)
            "Ophir 2 MAX" <- w2945
            n2044 = local read "System Stop"() -> (w2943:bool)
          }
        }
      }
      n2045 = VISA Close(VISA resource name=w2932, error in (no error)=w2933) -> (error out=w2934:errorcluster)
      n2046 = call "Ophir Error Message.vi"("error in (no error)"=w2934) -> ()  [unwired: 3 in, 4 out]
    }
  }
  n2047 = case shown="True" w38 {
    tunnel: w2 -> [_ w2960]
    frame False {
    }
    frame True {
      n2048 = local read "Ophir 1 dup Visa Session"() -> (w2962:refnum<visa-resource-name>)
      n2049 = local read "Ophir 1 error out"() -> (w2961:errorcluster)
      n2050 = while {
        tunnel: [w2973] -> w2964
        tunnel: [w2967] -> w2963
        tunnel: w2962 -> [w2971]
        tunnel: w2961 -> [w2970]
        tunnel: w2960 -> [_]
        shift-right: [w2968] -> _
        shift-left: 0.0 -> [w2969]
        stop <- w2972 stop-if-true
        n2051 = Wait (ms)(milliseconds to wait="Ophir 1 Wait") -> ()  [unwired: 1 out]
        n2052 = stacked-sequence {
          tunnel: [w2989] -> w2973
          tunnel: [w2974] -> w2972
          tunnel: w2971 -> [w2976]
          tunnel: w2970 -> [w2985]
          tunnel: w2969 -> [w2979]
          tunnel: [w2977] -> w2968
          tunnel: [w2976] -> w2967
          frame #0 {
            n2053 = Fract/Exp String To Number(string="Ophir 1 units") -> (number=w2978:dbl)  [unwired: 3 in, 1 out]
            n2054 = call "Ophir SendPower.vi"("Visa Session"=w2976, "error in (no error)"=w2985) -> ("Value Number"=w2975:dbl, "Value String"=w2987:string, "error out"=w2989:errorcluster)  [unwired: 1 out]
            "Ophir 1 Real Optical Power" <- w2975
            n2055 = call "Ophir Over.vi"("Value String"=w2987) -> ("Overrange"=→"Ophir 1 Over Range":bool)
            n2056 = Multiply(x=w2975, y=w2978) -> (x*y=w2983:dbl)
            "Ophir 1 Char" <- w2983
            "Ophir 1 Optical Power" <- w2983
            n2057 = Greater Or Equal?(x=w2983, y=w2979) -> (x >= y?=w2984:bool)
            n2058 = Select(t=0.0, s="Ophir 1 Clear", f=w2979) -> (s? t:f=w2982:dbl)
            n2059 = Select(t=w2983, s=w2984, f=w2982) -> (s? t:f=w2977:dbl)
            "Ophir 1 MAX" <- w2977
            n2060 = local read "System Stop"() -> (w2974:bool)
          }
        }
      }
      n2061 = VISA Close(VISA resource name=w2963, error in (no error)=w2964) -> (error out=w2965:errorcluster)
      n2062 = call "Ophir Error Message.vi"("error in (no error)"=w2965) -> ()  [unwired: 3 in, 4 out]
    }
  }
